vi "Maintenance.vi"() -> ()   [LabVIEW 2020]
doc: "Maintanence VI for FLS imaging system.\n[Covers: REQ9]\n[Covers: REQ10]"
uses:
  <userlib>/_OpenG.lib/file/file.llb/openg_file.lvlib
  <vilib>/event_ctls.llb/usereventprio.ctl
  <instrlib>/niScope/Acquire/Fetch/niScope Multi Fetch Binary 16.vi
  <instrlib>/niScope/Controls/niScope trigger source.ctl
  <userlib>/_OpenG.lib/time/time.llb/openg_time.lvlib
  SubVI/GlobalVariables.vi
  SubVI/LabJack/LJ Pin Setting.ctl
  <vilib>/Utility/error.llb/DialogType.ctl
  <vilib>/Analysis/NI_AALBase.lvlib
  <vilib>/Utility/miscctls.llb/LVMinMaxIncTypeDef.ctl
  <vilib>/Analysis/baseanly.llb/Mean (DBL).vi
  LaguerreDeconLib/DeconEngineClass/LaguerreDeconEngineClass.lvclass
  <vilib>/Utility/miscctls.llb/LVPointTypeDef.ctl
  <vilib>/addons/_JKI.lib/Serialization/JSON/JKI JSON Serialization.lvlib
  SubVI/APD/APDClass.lvclass
  <vilib>/Utility/miscctls.llb/LVRowAndColumnTypeDef.ctl
  SubVI/APD/GainData.ctl
  SubVI/APD/iRFData.ctl
  <vilib>/addons/control/pid/NI_PID_autopid.lvlib
  <vilib>/addons/control/pid/NI_PID_pid.lvlib
  <vilib>/addons/control/pid/pid.llb/PID Advanced (DBL).vi
  <vilib>/addons/control/pid/autopid.llb/PID Online Autotuning (Step Closed Loop).vi
  <vilib>/Instr/_visa.llb/VISA Configure Serial Port (Instr).vi
  SubVI/DigitizerConfiguration/FLImDAQ.ctl
  <vilib>/addons/control/pid/autopid.llb/PID autotuning parameters.ctl
panel:
  in  "Duty Cycle (%)":u32=25
  in  "AB Rep Rate":u16 caption="Rep Rate" max=1000 step=1 format="%.0dHz"
  in  "Current":dbl=1.0 min=1.0 max=63.0 step=1.0 format="%#.1fA"
  out "GainIndicator":dbl caption="Gain"
  out "Noise\n(std of DC)":dbl format="%0.6f"
  in  "BG flag?":bool
  out "DC":dbl format="%0.2f"
  out "Amplitude":dbl
  in  "Gain High":dbl max=4.5
  in  "Gain low":dbl=3.0
  in  "Step":dbl=0.1
  in  "Num WF to acquire":u64=18446744073709551615
  in  "Channel":enum32{"Ch1", "Ch2", "Ch3"}(radio)
  in  "Task":enum32{"iRFAndGain", "Alignment"}(radio)
  in  "Aiming beam toggle":bool caption="445nm 100Hz"
  in  "Laser Rep Rate":u16=120 caption="Rep Rate" min=5 max=4000 step=1 format="%.0dHz"
  in  "355nm Laser toggle":bool caption="355nm 460Hz"
  out "appended path":path
  out "Current State":string
  out "WF max value":dbl
  out "Disclamer":picture
  out "Calibration #":i8
  out "BG #":i8
  in  "TCP Connect":bool
  out "Help":string
  in  "Auto gain":bool=TRUE
  out "Run #":i8
  in  "StopButton":bool caption="Stop"
  out "System Status:":bool
  in  "StartButton":bool caption="Start"
  in  "Ctrl V":dbl=0.05 min=0.0 max=5.5 step=0.1 format="%#.3f"
  out "System Hardware Connection Status":T1
  out "Waveform (no average)":dbl[](graph)
  in  "Tab Control":T2(tab)
  out "Ch1 Max CtrlV":dbl
  out "Ch1 iRF Graph":dbl[][](graph)
  out "Ch1 Gain":cluster{"CtrlV":dbl[], "Gain":dbl[]}(graph)
  out "Serial Number Ch1":string caption="Serial Number"
  out "DateTimeCh1":string caption="DateTime"
  out "Ch2 Gain":cluster{"CtrlV":dbl[], "Gain":dbl[]}(graph)
  out "Ch2 iRF Graph":dbl[][](graph)
  out "Ch2 Max CtrlV":dbl
  out "Serial Number Ch2":string caption="Serial Number"
  out "DateTimeCh2":string caption="DateTime"
  out "Ch3 iRF Graph":dbl[][](graph)
  out "Ch3 Gain":cluster{"CtrlV":dbl[], "Gain":dbl[]}(graph)
  out "Serial Number Ch3":string caption="Serial Number"
  out "Ch3 Max CtrlV":dbl
  out "DateTimeCh3":string caption="DateTime"
  out "display loop timing(ms)":u32
  out "Aquisition loop timing(ms)":u32
  out "DisplayLoop":i32
  out "processing loop":i32
  out "processing loop timing(ms)":dbl
  out "laser EM lamp V":dbl format="%0.6f"
  out "aquisition loop Error Out":errorcluster
  out "Aq Loop?":bool
  out "processing Error Out":errorcluster
  out "Triggering:Trigger Delay":dbl
  out "Foot Pedal":bool
  out "LJ Pinout":T3={"Ch1 Bias"="DAC0", "Ch2 Bias"="DAC1", "Ch3 Bias"="DAC2", "Ch4 Bias"="DAC0", "355 PWM"="FIO0", "AimingBeam PWM"="FIO2", "Laser Ready"="FIO3", "Interlock"="FIO1", "Laser Start/Stop"="FIO1", "Red LED"="FIO1", "Green LED"="DIO3", "Foot Pedal"="DIO15"}
  out "FLImDAQ":T4={"Digitizer 1"="", "Digitizer 2"="", "Channel"=enum."Channel 0", "trigger source"="VAL_EXTERNAL", "trigger level"=0.5, "trigger delay"=1.35e-07, "min sample rate"=12500000000.0, "min record length"=2500, "vertical range"=1.0, "vertical offset"=-0.25, "Waveform to Avg"=2000} caption="FLIm DAQ Configuration" {"trigger delay" format="%^#.4e"; "trigger level" min=0.0 max=3.5 step=0.5 format="%.2f"; "vertical offset" format="%.4f"; "vertical range" format="%.2f"; "min sample rate" format="%#.2p"}
  out "Dig1 Temp":dbl
  out "Dig2 Temp":dbl
  in  "Sys Reconfig":bool
  out "Fetch Record #":i32
  out "Record Backlog":i32
  out "Fetch:Records Done":i32
  out "dt (s)":dbl format="%#_6p"
  in  "SaveData?":bool
  out "data Size":i32[](array[numeric])
  out "numWFInQ":i32
  in  "Clear WF Chart History":bool
  out "Waveform Chart":dbl(graph)
  in  "SaveiRFData":bool
  out "iRFDataTable":string[][](table)
  in  "SetIRFCtrlV":bool
  in  "ClearIRFData":bool
  in  "AcquireIRF":bool
  out "iRFInstSting":string="To aquire gain data, please start data aquisition! \nPlace blue (Ch1&2) or Green(Ch3) Chroma slide as close as possible to the fiber port! \nPlease remove channel 3 bandpass filter as well!"
  out "iRFSigInRange":bool caption="Signal  In Range?"
  out "Current iRF":dbl[](graph)
  out "iRFCtrlV":dbl[](array[numeric])
  in  "SaveGainData":bool
  out "GainInstSting":string="To aquire gain data, please start data aquisition! \nPlace blue (Ch1&2) or Green(Ch3) Chroma slide as close as possible to the fiber port! \nPlease remove channel 3 bandpass filter as well!"
  in  "ClearGainData":bool
  out "Gain":dbl[](array[numeric])
  in  "ComputeGain":bool
  out "Int Corr AUC":dbl[](array[numeric])
  out "AUC Std":dbl[](array[numeric])
  out "GainSigInRange":bool caption="Signal  In Range?"
  in  "AcquireGain":bool
  out "GainDataTable":string[][](table)
  out "Intensity Factor":dbl[](array[numeric])
  out "AUC":dbl[](array[numeric])
  out "Ctrl V":dbl[](array[numeric])
  out "XY Graph":cluster{"Ctrl V":dbl[], dbl[]}(graph)
  out "Parameters":T6(graph)
  in  "Save PID":bool
  out "Targer and Max":cluster{"V target(1.0)":dbl, dbl}(graph)
  out "Completed?":bool
  out "Gain(Log10)":dbl(graph)
  in  "Gain(Log)":dbl=1.0
  in  "Ch1 PID gains":T6={"proportional gain (Kc)"=0.5, "integral time (Ti, min)"=0.0003, "derivative time (Td, min)"=1e-05} {"derivative time (Td, min)" format="%.6f"; "integral time (Ti, min)" format="%.6f"; "proportional gain (Kc)" format="%.6f"}
  in  "autotune? (F)":bool
  in  "PID dt (s)":dbl=-1.0
  out "dt out (s)":dbl format="%.3f"
  in  "V target(1.0)":dbl=1.0 format="%#_2f"
  in  "Accept?":bool
  out "tuned PID gains":T6={"proportional gain (Kc)"=1.0, "integral time (Ti, min)"=0.01, "derivative time (Td, min)"=0.0} {"derivative time (Td, min)" format="%_6f"; "integral time (Ti, min)" format="%.6f"; "proportional gain (Kc)" format="%.6f"}
  in  "autotuning parameters":T7={"type of controller"=2, "relay cycles"=100, "relay amplitude"=0.25, "control specifications"=1, "PV noise level"=0.01} {"PV noise level" format="%.5f"; "control specifications" items=["normal", "fast", "slow"]; "relay amplitude" format="%.2f"; "type of controller" items=["P", "PI", "PID"]}
  in  "Ch2 PID gains":T6={"proportional gain (Kc)"=0.5, "integral time (Ti, min)"=0.0003, "derivative time (Td, min)"=1e-05} {"derivative time (Td, min)" format="%.6f"; "integral time (Ti, min)" format="%.6f"; "proportional gain (Kc)" format="%.6f"}
  in  "Ch3 PID gains":T6={"proportional gain (Kc)"=0.5, "integral time (Ti, min)"=0.0003, "derivative time (Td, min)"=1e-05} {"derivative time (Td, min)" format="%.6f"; "integral time (Ti, min)" format="%.6f"; "proportional gain (Kc)" format="%.6f"}
  in  "gamma":dbl=1.0 format="%.2f"
  in  "alpha":dbl=nan format="%.2f"
  in  "Quit":bool
  # "440nm Laser Setting"
  # "355nm Laser Setting"
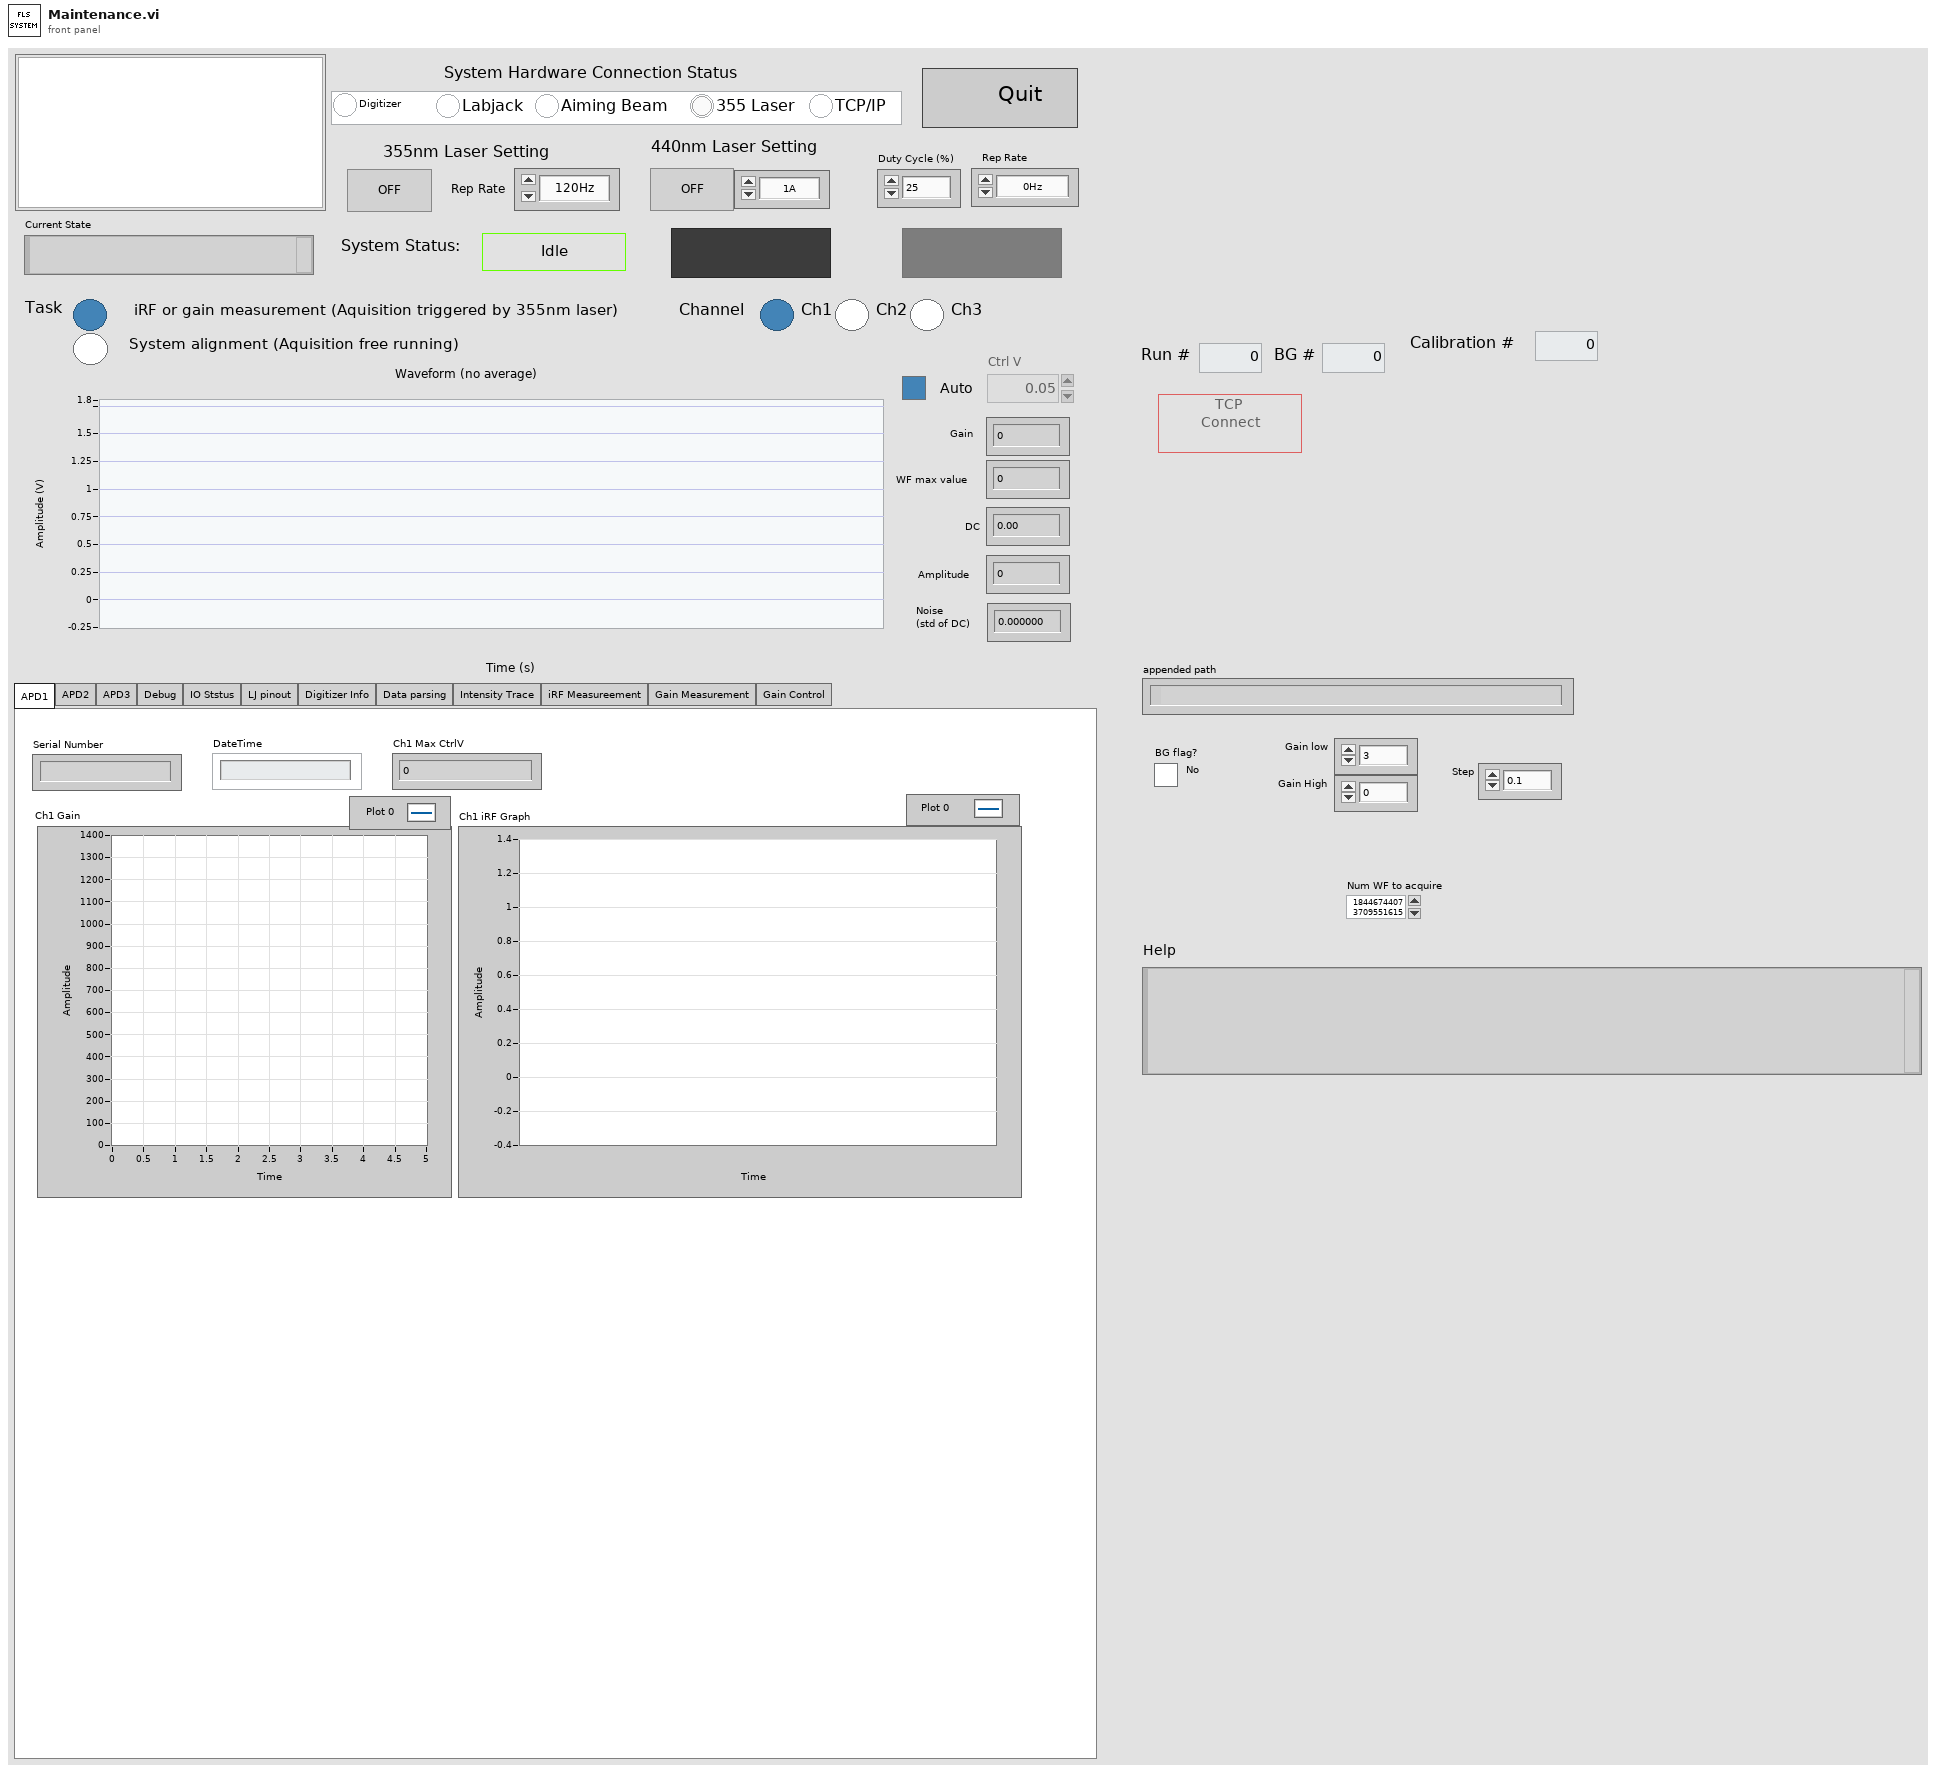
[diagram p1: front panel]
types:
  T1 = cluster{"Digitizer":bool, "Labjack":bool, "Aiming Beam":bool, "355 Laser":bool, "TCP/IP":bool}
  T2 = enum32{"APD1", "APD2", "APD3", "Debug", "IO Ststus", "LJ pinout", "Digitizer Info", "Data parsing", "Intensity Trace", "iRF Measureement", "Gain Measurement", "Gain Control"}
  T3 = typedef "LJ Pin Setting.ctl" = cluster{"Ch1 Bias":string, "Ch2 Bias":string, "Ch3 Bias":string, "Ch4 Bias":string, "355 PWM":string, "AimingBeam PWM":string, "Laser Ready":string, "Interlock":string, "Laser Start/Stop":string, "Red LED":string, "Green LED":string, "Foot Pedal":string}
  T4 = typedef "FLImDAQ.ctl" = cluster{"Digitizer 1":refnum<k15>, "Digitizer 2":refnum<k15>, "Channel":enum16{"Channel 0", "Channel 1", "Channel 0&1"}, "trigger source":T5, "trigger level":dbl, "trigger delay":dbl, "min sample rate":dbl, "min record length":i32, "vertical range":dbl, "vertical offset":dbl, "Waveform to Avg":i16}
  T5 = typedef "niScope trigger source.ctl" = string
  T6 = cluster{"proportional gain (Kc)":dbl, "integral time (Ti, min)":dbl, "derivative time (Td, min)":dbl}
  T7 = typedef "PID autotuning parameters.ctl" = cluster{"type of controller":u16, "relay cycles":i32, "relay amplitude":dbl, "control specifications":u16, "PV noise level":dbl}
  T8 = cluster{"CtrlV":dbl, "WFs":dbl[][], "WFavg":dbl[]}
  T9 = enum16{"open", "replace", "create", "open or create", "replace or create", "replace or create with confirmation"}
  T10 = typedef "LVPointTypeDef.ctl" = cluster{"Horizontal":i16, "Vertical":i16}
  T11 = enum8{"Enabled", "Disabled", "Disabled and Grayed Out"}
  T12 = enum32{"APD1", "APD2", "APD3", "Debug", "IO Ststus", "LJ pinout", "Digitizer Info", "Data parsing"}
  T13 = cluster{"CtrlV":dbl, "PeakV":dbl, "PeakV Std":dbl, "IntFactor":dbl, "IntCorrPeakV":dbl}
  T14 = enum16{"open", "open or create", "create or replace", "create", "open (read-only)"}
  T15 = enum32{"Invalid", "Standard", "Closed", "Hidden", "Minimized", "Maximized"}
  T16 = enum32{"invalid app kind", "Development System", "Run Time System", "Student Edition", "Embedded LabVIEW", "Evaluation", "Custom"}
  T17 = typedef "usereventprio.ctl" = enum32{"high priority", "normal priority"}
  T18 = enum32{"Bad", "Idle", "Run top level", "Running"}
  T19 = typedef "LVRowAndColumnTypeDef.ctl" = cluster{"Row":i32, "Column":i32}
  T20 = typedef "LVMinMaxIncTypeDef.ctl" = cluster{"Minimum":dbl, "Maximum":dbl, "Increment":dbl}
  T21 = cluster{"Aiming Beam COM Port":refnum<visa-resource-name>, "Min Current":dbl, "Max Current":dbl, "Default Current":dbl, "Frequency(Hz)":i32}
  T22 = cluster{"Core":cluster{"Current VI Reference":refnum<vi>, "Close Panel on Exit?":bool}, "SysConfigCluster":cluster{"Ch1Enable?":bool, "Ch2Enable?":bool, "Ch3Enable?":bool, "Ch1AutoGain?":bool, "Ch2AutoGain?":bool, "Ch3AutoGain?":bool, "AimingBeamEnable?":bool}, "System Status":cluster{"Digitizer":bool, "Labjack":bool, "Aiming Beam":bool, "355 Laser":bool, "TCP/IP":bool}, "IDs":cluster{"RunID":i8, "BG ID":i8, "Cali ID":i8}, "DefaultPath":path, "Pathes":cluster{"DataPath":path, "BG Path":path, "iRFPath":path, "CaliPath":path}, "FLImDAQ":cluster{"resource name":refnum<k15>, "resource name 2":refnum<k15>, "Channel":enum16{"Channel 0", "Channel 1", "Channel 0&1"}, "trigger source":T5, "trigger level":dbl, "trigger delay":dbl, "min sample rate":dbl, "min record length":i32, "vertical range":dbl, "vertical offset":dbl, "Waveform to Avg":i32}, "SysRunning?":bool, "AB Cluster":cluster{"Aiming Beam COM Port":refnum<visa-resource-name>, "Min Current":dbl, "Max Current":dbl, "Default Current":dbl, "Frequency(Hz)":i32}, "LJ Pinout":T3, "355 PWM setting":cluster{"DIO_EF_CLOCK1_DIVISOR":i16, "DIO_EF_CLOCK1_ROLL_VALUE":i32, "DIO#_EF_INDEX":i16, "DIO#_EF_OPTIONS":i16, "DIO#_EF_CONFIG_A":i32}, "AB PWM setting":cluster{"DIO_EF_CLOCK1_DIVISOR":i16, "DIO_EF_CLOCK1_ROLL_VALUE":i32, "DIO#_EF_INDEX":i16, "DIO#_EF_OPTIONS":i16, "DIO#_EF_CONFIG_A":i32}, "Last Trigger":u32, "niTClk sessions":refnum<k20>[], "Laser start tic":u32, "TCP attempt count":i32, "iRFAllGain":dbl[][], "SlowTimer":u32, "FastTimer":u32, "TempPath":path, "LED vi reference":refnum<vi>, "APDSerials":cluster{"Ch1Serial":string, "Ch2Serial":string, "Ch3Serial":string}, "LedViRefOpen":bool, "GainBGRaw":dbl[][], "GainDataTemp":cluster{"CtrlV":dbl, "AUC":dbl, "AUC Std":dbl, "IntFactor":dbl, "IntCorrAUC":dbl}, "iRFIdx":i32}
  T23 = cluster{"CtrlV":dbl, "AUC":dbl, "AUC Std":dbl, "IntFactor":dbl, "IntCorrAUC":dbl}
  T24 = cluster{"Ch1Serial":string, "Ch2Serial":string, "Ch3Serial":string}
  T25 = cluster{"DataPath":path, "BG Path":path, "iRFPath":path, "CaliPath":path}
  T26 = cluster{"DIO_EF_CLOCK1_DIVISOR":i16, "DIO_EF_CLOCK1_ROLL_VALUE":i32, "DIO#_EF_INDEX":i16, "DIO#_EF_OPTIONS":i16, "DIO#_EF_CONFIG_A":i32}
  T27 = cluster{"resource name":refnum<k15>, "resource name 2":refnum<k15>, "Channel":enum16{"Channel 0", "Channel 1", "Channel 0&1"}, "trigger source":T5, "trigger level":dbl, "trigger delay":dbl, "min sample rate":dbl, "min record length":i32, "vertical range":dbl, "vertical offset":dbl, "Waveform to Avg":i32}
  T28 = cluster{"Ch1Enable?":bool, "Ch2Enable?":bool, "Ch3Enable?":bool, "Ch1AutoGain?":bool, "Ch2AutoGain?":bool, "Ch3AutoGain?":bool, "AimingBeamEnable?":bool}
  T29 = cluster{"Current VI Reference":refnum<vi>, "Close Panel on Exit?":bool}
  T30 = typedef "DialogType.ctl" = u16
  T31 = typedef "LJ PWM Setting.ctl" = cluster{"DIO_EF_CLOCK1_DIVISOR":i16, "DIO_EF_CLOCK1_ROLL_VALUE":i32, "DIO#_EF_INDEX":i16, "DIO#_EF_OPTIONS":i16, "DIO#_EF_CONFIG_A":i32}
  T32 = typedef "AimingBeam.ctl" = cluster{"Aiming Beam COM Port":refnum<visa-resource-name>, "Min Current":dbl, "Max Current":dbl, "Default Current":dbl, "Frequency(Hz)":u32}
  T33 = typedef "LVBoundsTypeDef.ctl" = cluster{"Width":u32, "Height":u32}
  T34 = typedef "imagedata.ctl" = cluster{"image type":i32, "image depth":i32, "image":u8[], "mask":u8[], "colors":u32[], "Rectangle":cluster{"left":i16, "top":i16, "right":i16, "bottom":i16}}
  T35 = typedef "LVCursorListTypeDef.ctl" = cluster{"Name":string, "Color":u32, "Style":u8, "Point Style":u8, "Name Visible":bool, "Allow Drag":bool, "Cursor Mode":u32, "Plot":i32, "Index":i32, "Position":cluster{"X":dbl, "Y":dbl}, "X Scale":u32, "Y Scale":u32, "Watch Plots":i32[], "Watch All Plots":bool, "Plot Area":i32, "Label Offset":cluster{"X":dbl, "Y":dbl}}[]
  T36 = cluster{"Name":string, "Color":u32, "Style":u8, "Point Style":u8, "Name Visible":bool, "Allow Drag":bool, "Cursor Mode":u32, "Plot":i32, "Index":i32, "Position":cluster{"X":dbl, "Y":dbl}, "X Scale":u32, "Y Scale":u32, "Watch Plots":i32[], "Watch All Plots":bool, "Plot Area":i32, "Label Offset":cluster{"X":dbl, "Y":dbl}}
  T37 = cluster{"Name":string, "Color":u32, "Style":u8, "Point Style":u8, "Name Visible":bool, "Allow Drag":bool, "Cursor Mode":u32, "Plot":i32, "Index":i32, "Position":cluster{"X":dbl, "Y":dbl}, "X Scale":u32, "Y Scale":u32, "Watch Plots":i32[], "Watch All Plots":bool, "Plot Area":i32, "Label Offset":cluster{"X":dbl, "Y":dbl}}[]
  T38 = cluster{"Ch1APDSerial#":string, "Ch2APDSerial#":string, "Ch3APDSerial#":string, "Ch4APDSerial#":string}
  T39 = cluster{"Ch1APDSerial#":string, "Ch2APDSerial#":string, "Ch3APDSerial#":string}
  T40 = typedef "GainData.ctl" = cluster{"CtrlV":dbl[], "NumOfWFs":i32, "WF length":i32, "Gain":dbl[], "GainRaw":dbl[][], "GainBGRaw":dbl[][]}
  T41 = typedef "iRFData.ctl" = cluster{"dt":dbl, "NumOfWFs":i32, "WFLength":i32, "iRFCtrlV":dbl[], "iRFWFsAvg":dbl[][], "iRFRaw":dbl[][]}
  T42 = cluster{"CtrlV":dbl, "WFs":dbl[][], "WFavg":dbl[]}[]
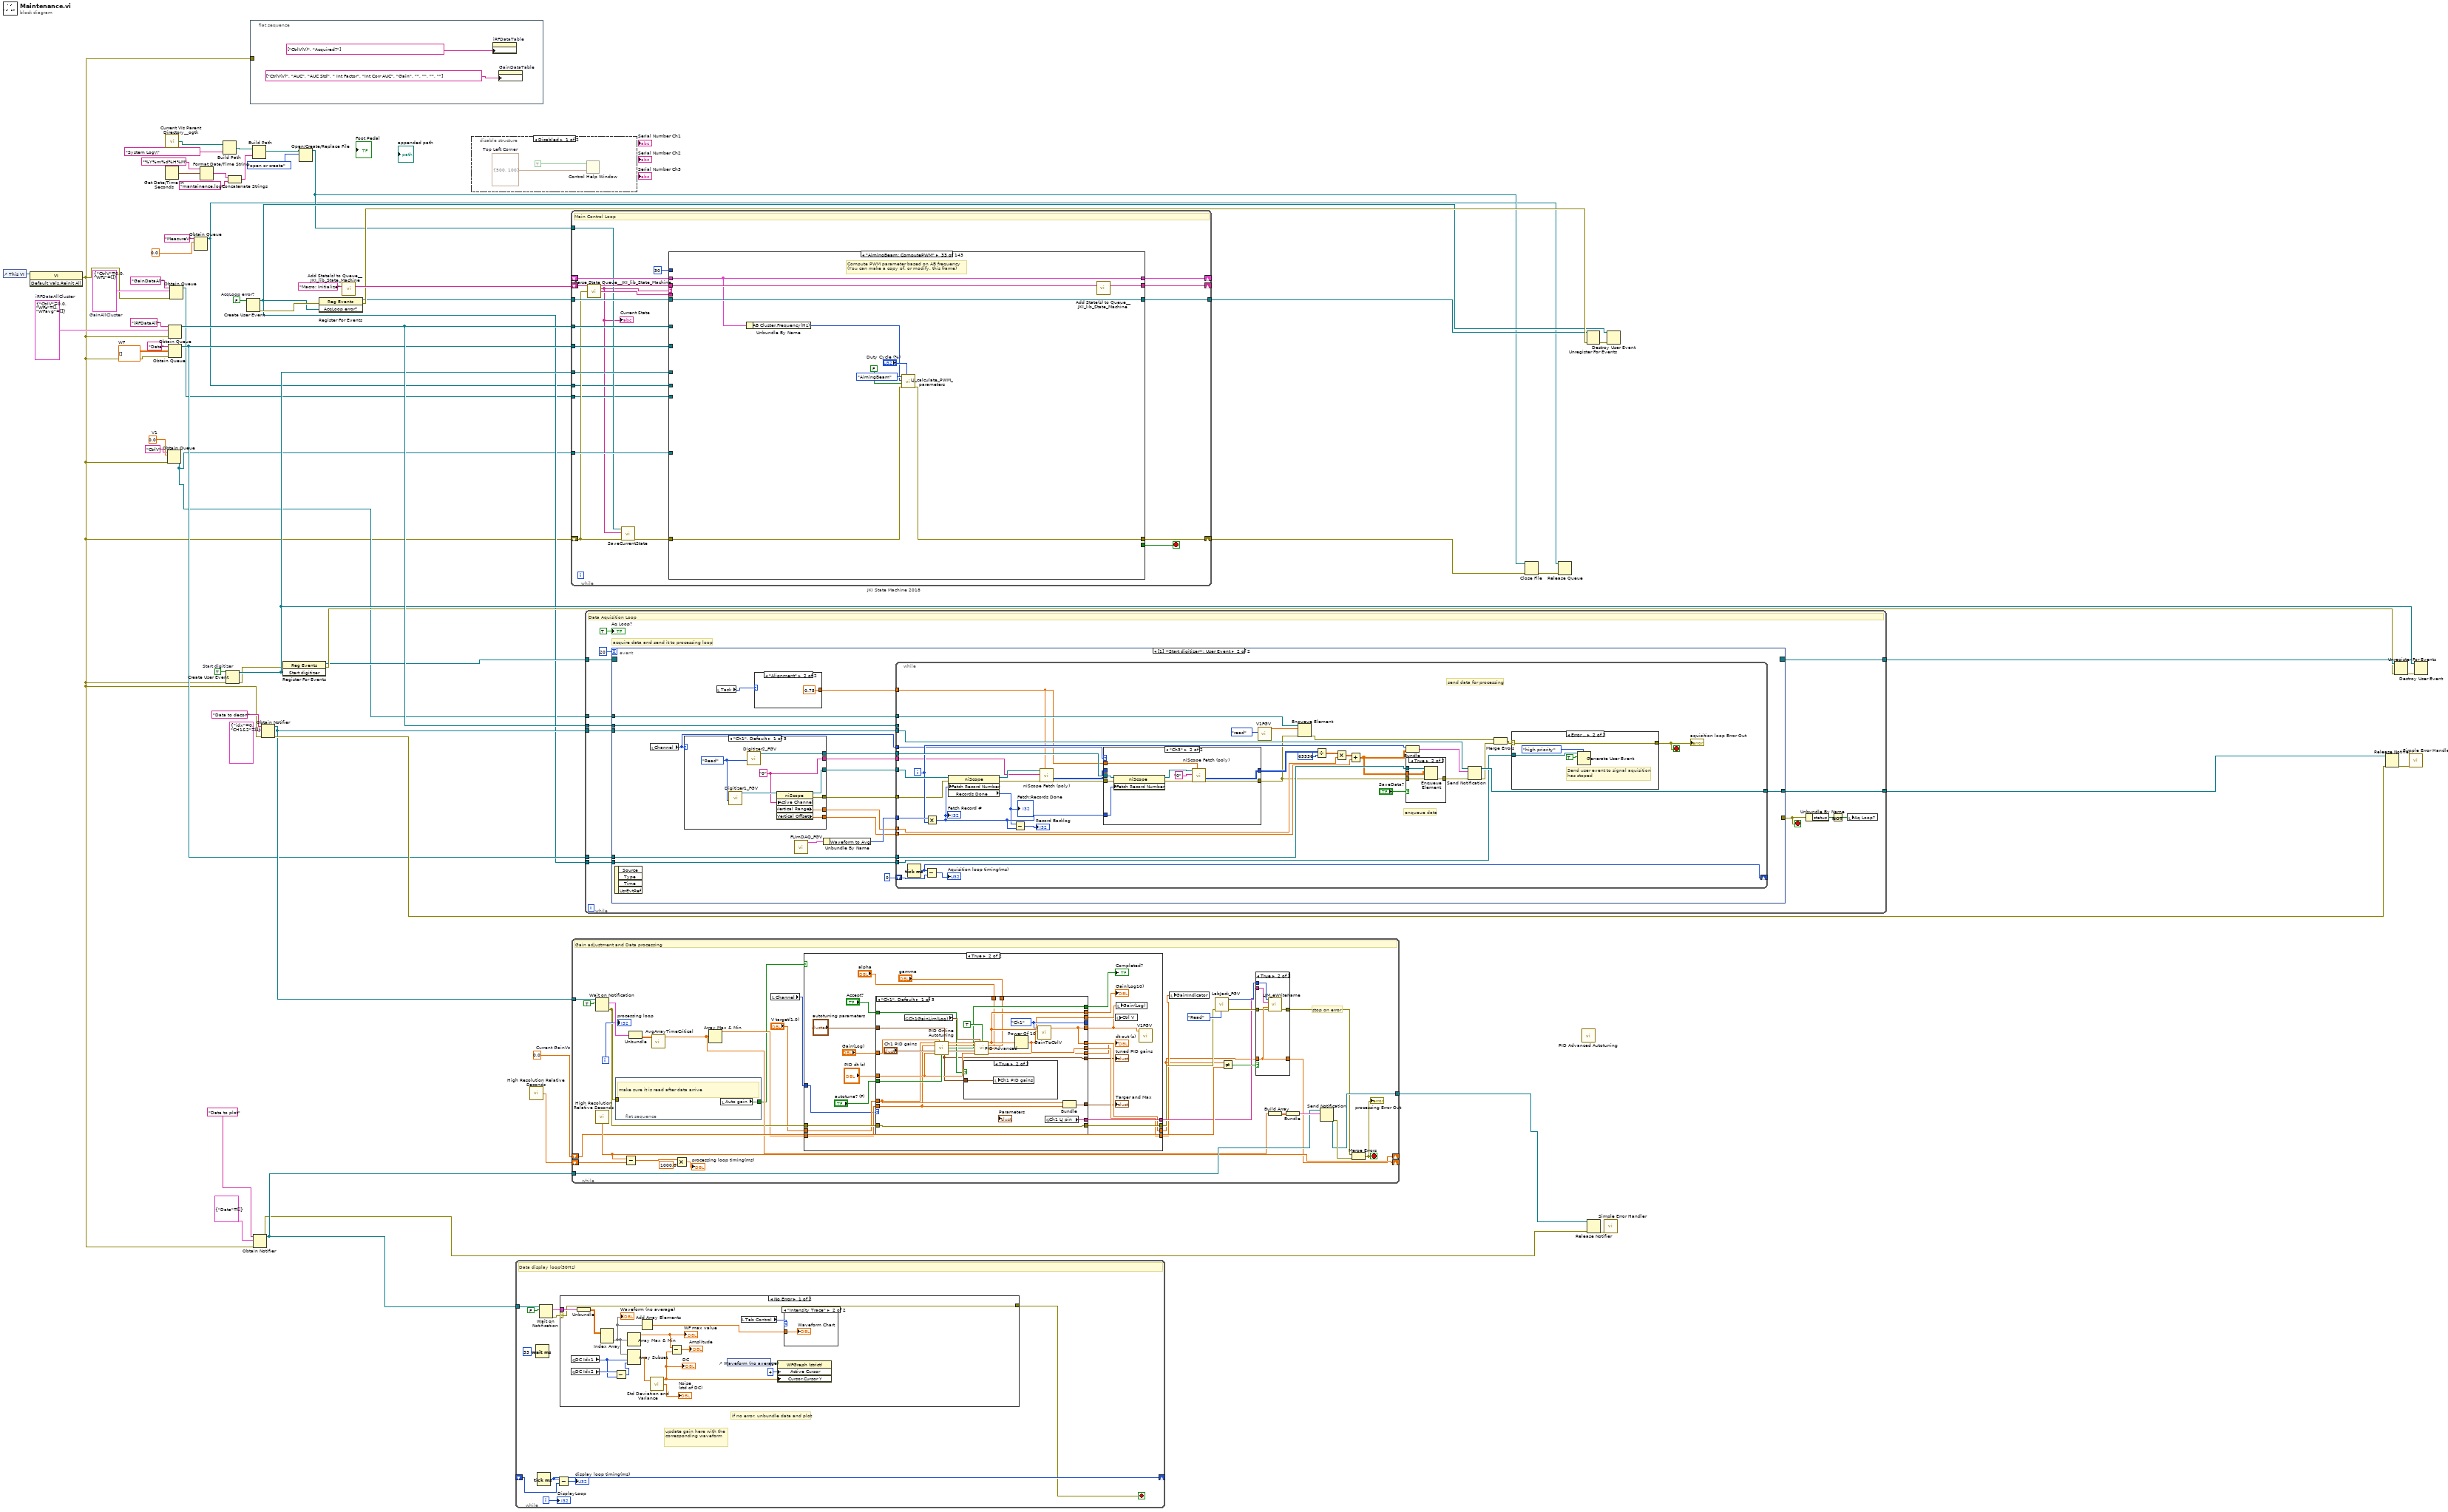
[diagram p0: block diagram]
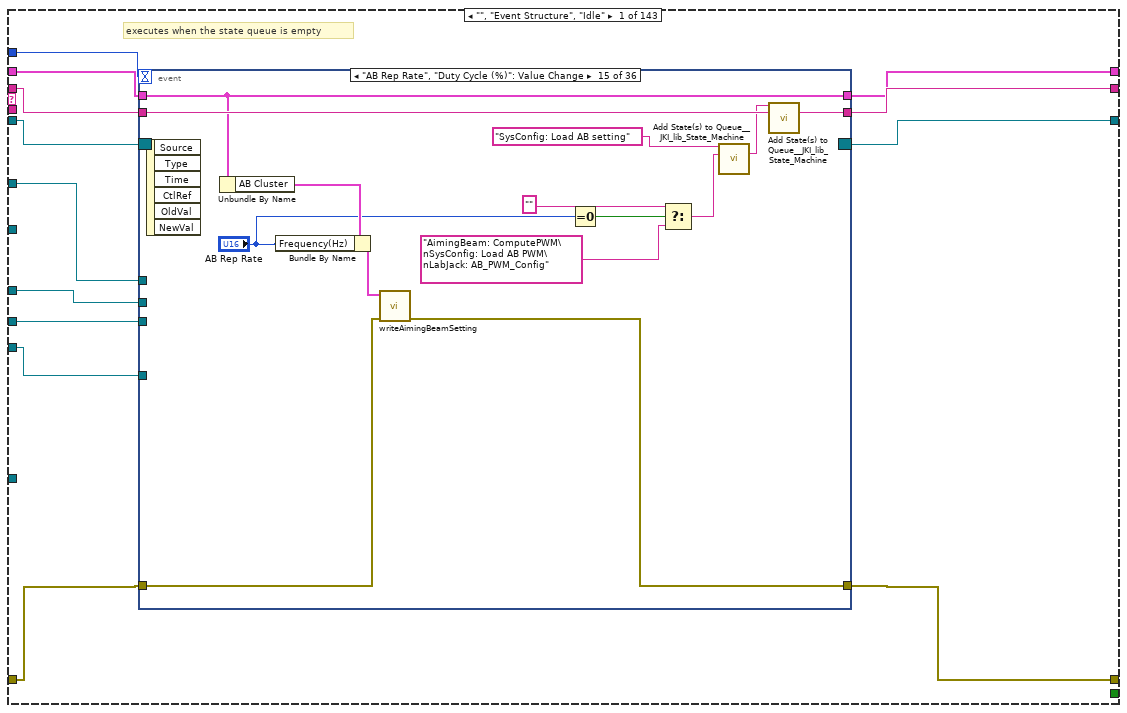
[diagram p3: hidden frame]
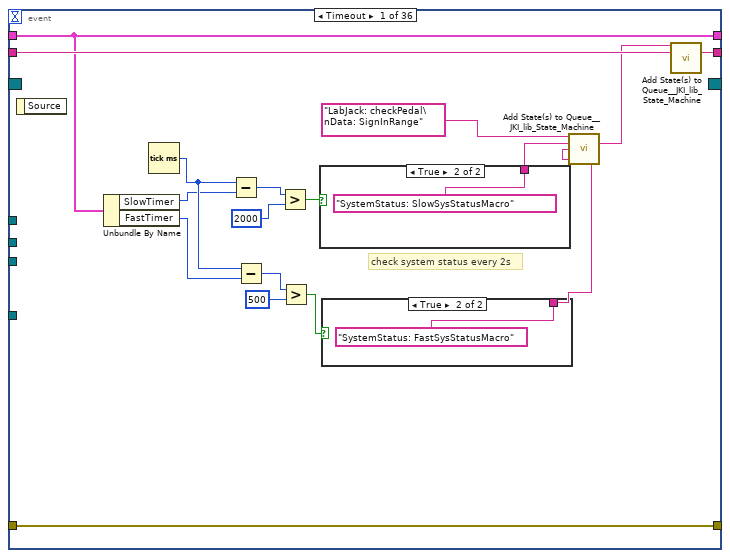
[diagram p4: hidden frame]
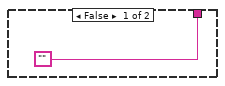
[diagram p5: hidden frame]
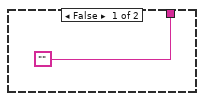
[diagram p6: hidden frame]
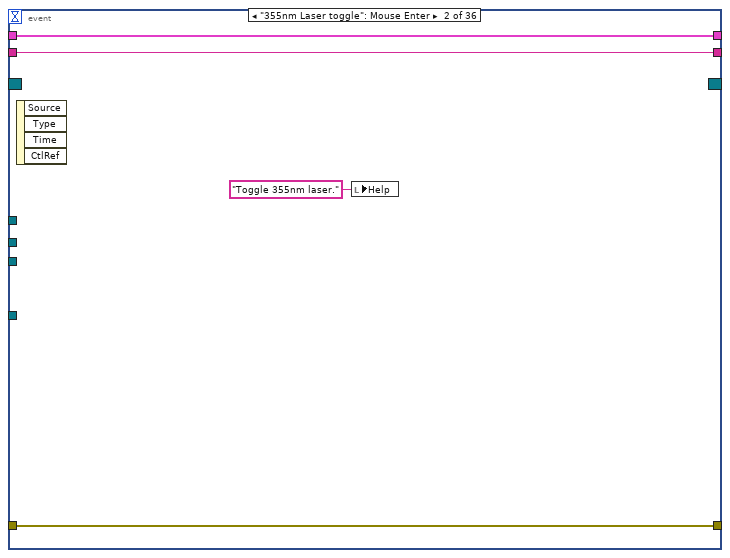
[diagram p7: hidden frame]
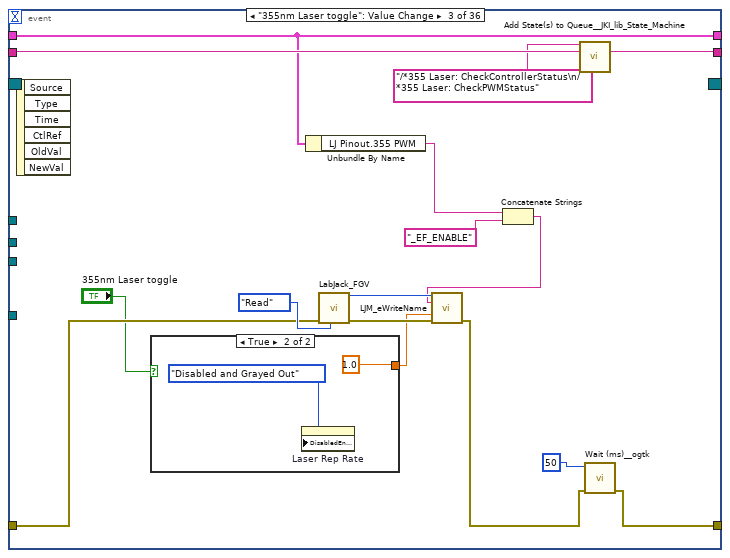
[diagram p8: hidden frame]
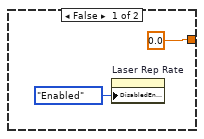
[diagram p9: hidden frame]
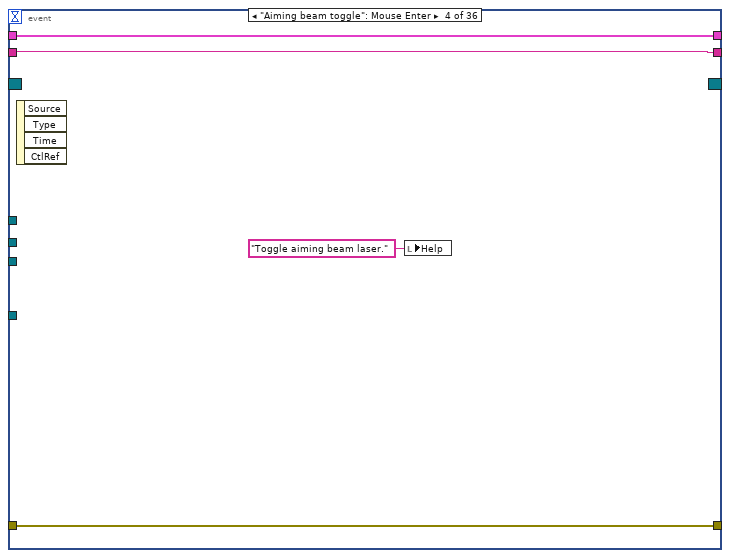
[diagram p10: hidden frame]
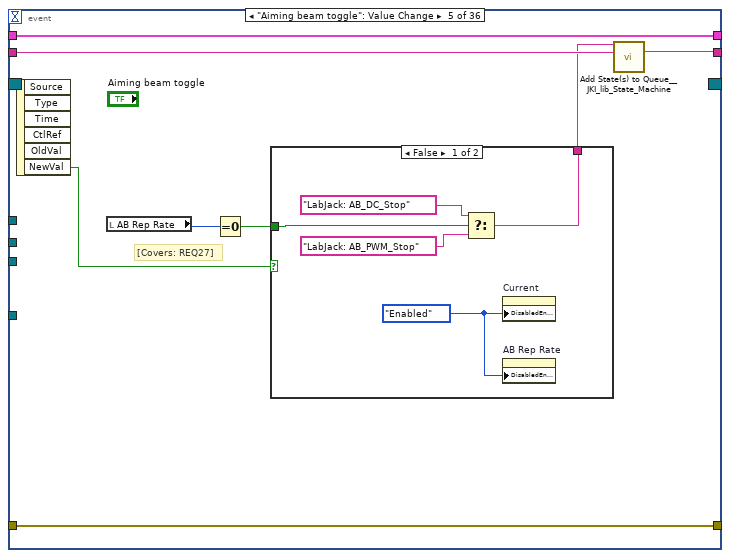
[diagram p11: hidden frame]
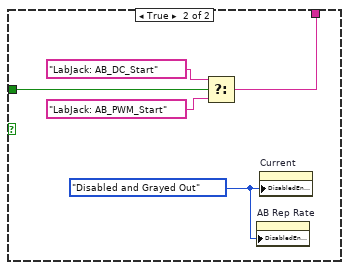
[diagram p12: hidden frame]
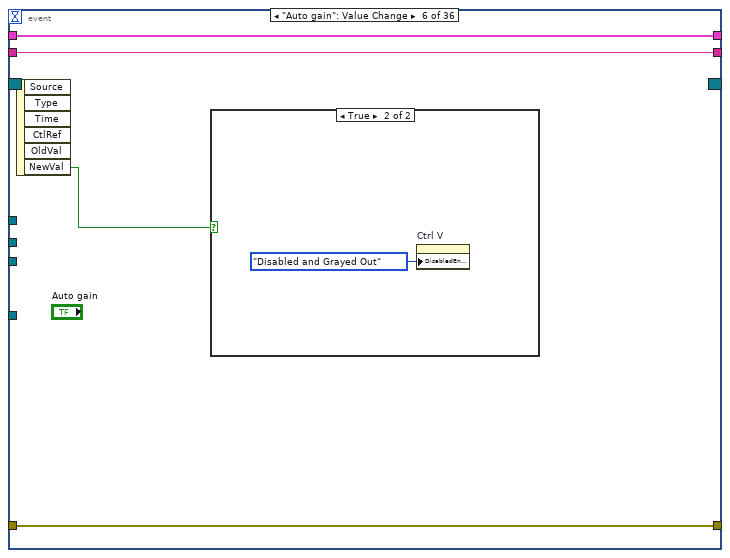
[diagram p13: hidden frame]
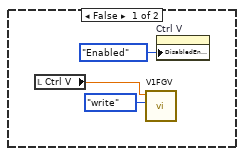
[diagram p14: hidden frame]
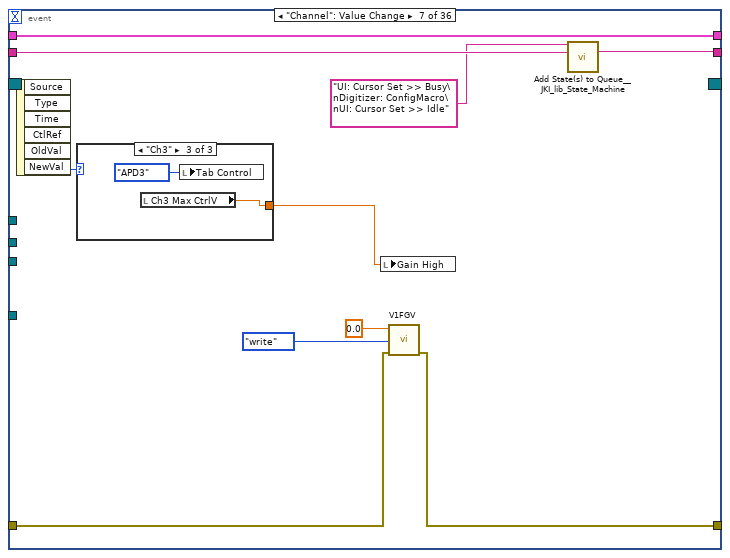
[diagram p15: hidden frame]
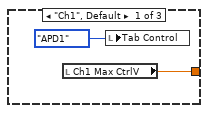
[diagram p16: hidden frame]
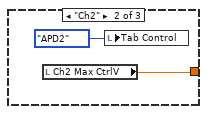
[diagram p17: hidden frame]
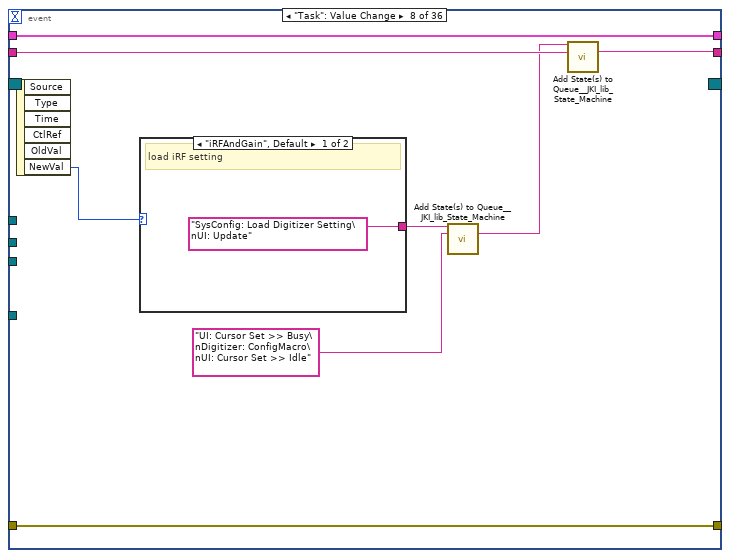
[diagram p18: hidden frame]
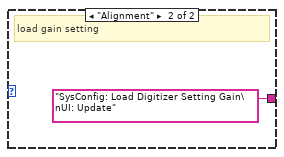
[diagram p19: hidden frame]
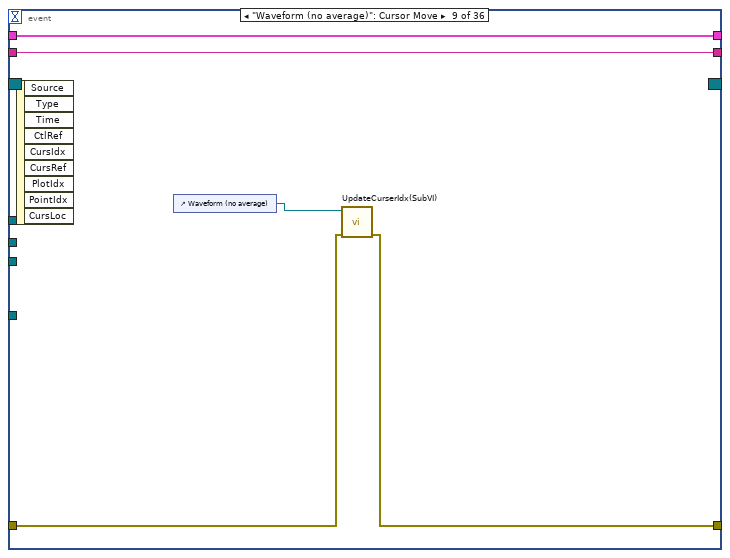
[diagram p20: hidden frame]
diagram:
  w3 = cluster{"CtrlV":dbl, "WFs":dbl[][]} {"CtrlV"=0.0, "WFs"=[]}  # GainAllCluster
  w5 = T8 {"CtrlV"=0.0, "WFs"=[], "WFavg"=[]}  # iRFDataAllCluster
  w22 = 0.0  # V1
  w26 = 0.0  # Current GainVs
  w43 = FALSE  # AcqLoop error?
  w53 = TRUE  # Start digitizer
  w56 = dbl[][] []  # WF
  n1 = control-ref of="This VI"() -> (w58:refnum<vi>)
  n2 = invoke on="Invoke Node" class="VI" method="Default Vals.Reinit All"(reference=w58) -> (error out=w1:errorcluster)  [unwired: 2 in, 2 out]
  n3 = call <userlib>:"Current VIs Parent Directory__ogtk.vi"() -> ("Parent Directory (+ Relative)"=w21:path)  [unwired: 5 in]
  n4 = Get Date/Time In Seconds() -> (seconds since 1Jan1904=w19:timestamp)
  n5 = Obtain Queue(name (unnamed)="CtrlV", element data type=w22, error in (no error)=w1) -> (queue out=w24:refnum<queue>)  [unwired: 2 in, 2 out]
  n6 = Obtain Queue(name (unnamed)="Data", element data type=w56, error in (no error)=w1) -> (queue out=w32:refnum<queue>)  [unwired: 2 in, 2 out]
  n7 = Obtain Queue(name (unnamed)="iRFDataAll", element data type=w5, error in (no error)=w1) -> (queue out=w54:refnum<queue>)  [unwired: 2 in, 2 out]
  n8 = Obtain Queue(name (unnamed)="GainDataAll", element data type=w3, error in (no error)=w1) -> (queue out=w2:refnum<queue>)  [unwired: 2 in, 2 out]
  n9 = Obtain Queue(name (unnamed)="MeasureV", element data type=0.0) -> (queue out=w6:refnum<queue>)  [unwired: 3 in, 2 out]
  n10 = Format Date/Time String(time format string (%c)="%Y%m%d%H%M", seconds (now)=w19) -> (date/time string=w16:string)  [unwired: 1 in]
  n11 = Build Path(base path=w21, name or relative path="System Log\\") -> (appended path=w12:path)
  n12 = Create User Event(user event datatype=w53, error in=w1) -> (user event=w42:refnum<user-event>, error out=w28:errorcluster)
  n13 = Concatenate Strings(w16, "mantainence.log" ("string")) -> (w14:string)
  n14 = Create User Event(user event datatype=w43) -> (user event=w27:refnum<user-event>, error out=w29:errorcluster)  [unwired: 1 in]
  n15 = flat-sequence {
    tunnel: w1 -> [_]
    frame #0 {
      n16 = property on="iRFDataTable" class="Tbl (strict)"("Column Headers[]"=string[] ["CtrlV(V)", "Acquired?"] ("Column Header Strings[]")) -> ()  [unwired: 2 in, 2 out]
      n17 = property on="GainDataTable" class="Tbl (strict)"("Column Headers[]"=string[] ["CtrlV(V)", "AUC", "AUC Std", " Int Factor", "Int Corr AUC", "Gain", "", "", "", ""] ("Column Header Strings[]")) -> ()  [unwired: 2 in, 2 out]
    }
  }
  n18 = Build Path(base path=w12, name or relative path=w14) -> (appended path=w17:path)
  n19 = Obtain Notifier(name (unnamed)="Data to plot", notification data type=cluster{"Data":dbl[][]} {"Data"=[]}, error in (no error)=w1) -> (notifier out=w36:refnum<notifier>, error out=w33:errorcluster)  [unwired: 1 in, 1 out]
  n20 = Obtain Notifier(name (unnamed)="Data to decon", notification data type=cluster{"idx":i32, "CH1&2":dbl[][]} {"idx"=0, "CH1&2"=[]}, error in (no error)=w1) -> (notifier out=w39:refnum<notifier>, error out=w47:errorcluster)  [unwired: 1 in, 1 out]
  n21 = register-events(error in=w28, w42) -> (reference out=w44:refnum<event-registration>, error out=w50:errorcluster)  [unwired: 1 in]
  n22 = Open/Create/Replace File(file path (use dialog)=w17, operation (0:open)=T9."open or create") -> (refnum out=w10:refnum<file>)  [unwired: 4 in, 2 out]
  n23 = register-events(error in=w29, w27) -> (reference out=w31:refnum<event-registration>, error out=w40:errorcluster)  [unwired: 1 in]
  n24 = call <vilib>:"Add State(s) to Queue__JKI_lib_State_Machine.vi"("State(s) in (\"\")"="Macro: Initialize") -> ("States Out"=w60:string)  [unwired: 14 in]
  n25 = disable-structure "Diagram Disable Structure" shown="Disabled" {
    frame Disabled {
      w63 = T10 {"Horizontal"=500, "Vertical"=100}  # Top Left Corner
      n26 = Control Help Window(0:w63, 1:TRUE ("Show")) -> ()
    }
    frame Enabled {
    }
  }
  n27 = while {
    tunnel: w36 -> [w74]
    shift-right: [w68] -> _
    shift-left: _ -> [w72]
    i -> [w66]
    stop <- w65 stop-if-true
    # "if no error, unbundle data and plot"
    # "update gain here with the corresponding waveform"
    # "Data display loop(30Hz)"
    n28 = Wait (ms)(milliseconds to wait=u32 33) -> ()  [unwired: 1 out]
    n29 = Tick Count (ms)() -> (millisecond timer value=w68:u32)
    n30 = Wait on Notification(notifier=w74, ignore previous (F)=FALSE) -> (notification=w69:cluster{"Data":dbl[][]}, error out=w67:errorcluster)  [unwired: 2 in, 2 out]
    n31 = Subtract(x=w68, y=w72) -> (x-y=→"display loop timing(ms)":u32)
    n32 = case shown="No Error" w67 {
      selector: w67 -> [w83 w92]
      tunnel: w69 -> [w90 _]
      tunnel: [w83 w92] -> w65
      frame No Error {
        n33 = global read "GlobalVariables.vi" "DC Idx1"() -> (w76:i32)
        n34 = global read "GlobalVariables.vi" "DC Idx2"() -> (w77:i32)
        n35 = Unbundle(w90) -> ("Data"=w87:dbl[][])
        n36 = Index Array(array=w87) -> (element=w86:dbl[])  [unwired: 2 in]
        "Waveform (no average)" <- w86
        n37 = Subtract(x=w77, y=w76) -> (x-y=w75:i32)
        n38 = Array Max & Min(array=w86) -> (max value=w89:dbl)  [unwired: 3 out]
        "WF max value" <- w89
        n39 = Array Subset(array=w86, index=w76, length=w75) -> (w82:dbl[])
        n40 = Add Array Elements(numeric array=w86) -> (sum=w85:dbl)
        n41 = call <vilib>:"Std Deviation and Variance.vi"("X"=w82) -> ("mean"=w78:dbl, "standard deviation"=→"Noise\n(std of DC)":dbl)  [unwired: 1 in, 1 out]
        "DC" <- w78
        n42 = Subtract(x=w89, y=w78) -> (x-y=→"Amplitude":dbl)
        n43 = control-ref of="Waveform (no average)"() -> (w80:refnum<vi>)
        n44 = local read "Tab Control"() -> (w84:T2)
        n45 = property class="WFGraph (strict)"(reference=w80, "Active Cursor"=u32 4, "Cursor.Cursor Y"=w78) -> ()  [unwired: 1 in, 2 out]
        n46 = case shown="\"Intensity Trace\"" w84 {
          tunnel: w85 -> [_ w91]
          frame "APD1", Default {
          }
          frame "Intensity Trace" {
            "Waveform Chart" <- w91
          }
        }
      }
      frame Error {
      }
    }
    "DisplayLoop" <- w66
  }
  n47 = call <vilib>:"High Resolution Relative Seconds.vi"() -> ("relative seconds"=w23:dbl)
  n48 = while "JKI State Machine 2018" {
    shift-right: [w109] -> _
    shift-left: _ -> [w108]
    shift-right: [w99] -> w11
    shift-left: w1 -> [w98]
    shift-right: [w110] -> _
    shift-left: w60 -> [w111]
    tunnel: w54 -> [w106]
    tunnel: w32 -> [w105]
    tunnel: w42 -> [w104]
    tunnel: w31 -> [w103]
    tunnel: [w102] -> w30
    tunnel: w24 -> [w100]
    tunnel: w10 -> [w96]
    tunnel: w6 -> [w95]
    tunnel: w2 -> [w94]
    stop <- w101 stop-if-true
    # "Main Control Loop"
    n49 = call <vilib>:"Parse State Queue__JKI_lib_State_Machine.vi"("State Queue"=w111, "Error In (no error)"=w98) -> ("Remaining States"=w113:string, "Current State"=w93:string, "Arguments"=w112:string)  [unwired: 11 in]
    "Current State" <- w93
    n50 = call "SaveCurrentState.vi"("error in (no error)"=w98, "Current State"=w93, "Byte Stream File in"=w96) -> ("error out"=w97:errorcluster)  [unwired: 8 in]
    n51 = case shown="\"AimingBeam: ComputePWM\"" w93 {
      selector: w93 -> [_ _ _ _ _ _ _ _ _ _ _ _ _ _ _ _ _ _ _ _ _ _ w826 _ _ _ _ _ _ _ _ _ _ _ _ _ _ _ _ _ _ _ _ _ _ _ _ _ _ _ _ _ _ _ _ _ _ _ _ _ _ _ _ _ _ _ _ _ _ _ _ _ _ _ _ _ _ _ _ _ _ _ _ _ _ _ _ _ _ _ _ _ _ _ _ _ _ _ _ _ _ _ _ _ _ _ _ _ _ _ _ _ _ _ _ _ _ _ _ _ _ _ _ _ _ _ _ _ _ _ _ _ _ _ _ _ _ _ _ _ _ _ _]
      tunnel: w113 -> [w126 w458 w467 w473 w480 w489 w500 w509 w534 w549 w580 w586 w611 w632 w649 w661 w692 w725 w780 w812 w819 w824 w830 w855 w863 w887 w892 w904 w913 w930 w938 w954 w978 w983 w993 w1016 w1065 w1096 w1119 w1142 w1165 w1190 w1213 w1247 w1262 w1278 w1283 w1294 w1305 w1321 w1359 w1376 w1390 w1424 w1435 w1441 w1452 w1464 w1495 w1527 w1540 w1553 w1567 w1581 w1586 w1598 w1610 w1623 w1636 w1652 w1680 w1695 w1700 w1709 w1747 w1760 w1768 w1776 w1790 w1795 w1801 w1818 w1835 w1851 w1871 w1896 w1904 w1909 w1917 w1925 w1930 w1939 w1978 w2018 w2023 w2046 w2059 w2077 w2083 w2094 w2107 w2125 w2132 w2144 w2209 w2220 w2233 w2258 w2281 w2287 w2293 w2308 w2353 w2361 w2367 w2372 w2378 w2386 w2395 w2405 w2411 w2417 w2422 w2428 w2441 w2475 w2484 w2495 w2517 w2539 w2566 w2631 w2648 w2703 w2752 w2768 w2778 w2801 w2806 w2828 w2836 w2845 w2850]
      tunnel: w112 -> [_ _ _ _ _ _ _ _ _ _ _ _ _ _ _ _ _ _ _ _ _ _ _ _ _ _ _ _ _ _ w937 _ _ _ _ _ _ _ _ _ _ _ _ _ _ _ _ _ _ _ _ _ _ _ _ _ _ w1462 _ _ _ _ _ _ _ _ _ _ _ _ _ _ _ _ _ _ _ _ _ _ _ _ _ _ _ _ _ _ _ _ _ _ _ _ _ w2037 _ _ _ _ _ _ w2127 w2139 _ _ _ _ w2277 _ _ _ _ _ _ _ w2373 _ w2387 w2400 _ _ _ _ _ _ _ _ _ _ _ _ _ _ _ _ _ w2792 _ _ _ _ _]
      tunnel: w108 -> [w124 w455 w463 w470 w476 w483 w497 w507 w518 w546 _ w583 w605 w623 w646 w652 w689 w719 w762 w785 w813 w821 w828 w838 w860 w885 w889 w894 w906 w915 w931 w950 w970 w980 w990 w1013 w1030 w1080 w1104 w1126 w1149 w1172 w1210 w1234 w1260 w1264 w1280 w1287 w1298 w1310 w1347 w1363 w1380 w1400 w1433 w1438 w1442 w1454 w1472 w1505 w1529 w1542 w1556 w1569 w1583 w1595 w1607 w1618 w1630 w1647 w1668 w1683 w1697 w1705 w1745 w1757 w1765 w1774 w1788 w1792 w1799 w1802 w1819 w1836 w1852 w1877 w1900 w1906 w1910 w1918 w1927 w1936 w1973 w1999 w2030 w2043 w2057 w2074 w2080 w2087 w2099 w2121 w2130 w2137 w2206 w2211 w2225 w2250 w2278 w2284 w2290 w2294 w2340 w2358 w2364 w2369 w2375 w2383 w2392 w2402 w2408 w2414 w2419 w2425 w2439 w2473 w2481 w2493 w2501 w2523 w2564 w2628 w2642 w2697 w2750 w2765 w2776 w2793 w2803 w2807 w2833 w2843 w2847]
      tunnel: [w123 w456 w465 w471 w478 w487 w498 w501 w532 w547 w578 w584 w601 w617 w647 w656 w690 w700 w768 w791 w816 w822 w832 w853 errorcluster {"status"=FALSE, "code"=0, "source"=""} ("error out") w884 w890 w899 w911 w922 w935 w949 w972 w981 w991 w1011 w1056 w1088 w1111 w1134 w1157 w1183 w1205 w1236 w1250 w1268 w1281 w1284 w1295 w1315 w1348 w1370 w1383 w1404 w1427 w1439 w1450 w1456 w1477 w1509 w1532 w1545 w1557 w1573 w1584 w1588 w1600 w1619 w1631 w1641 w1670 w1685 w1698 w1702 w1740 w1758 w1766 w1771 w1785 w1793 w1796 w1807 w1824 w1846 w1866 w1891 w1897 w1907 w1915 w1923 w1928 w1937 w1976 w2016 w2031 w2044 w2056 w2075 w2081 w2092 w2105 w2123 w2128 w2141 w2207 w2217 w2229 w2253 w2279 w2285 w2291 w2299 w2345 w2359 w2365 w2370 w2376 w2384 w2393 w2403 w2409 w2415 w2420 w2426 w2434 w2470 w2482 w2487 w2500 w2522 w2549 w2627 w2643 w2699 w2744 w2766 w2772 w2795 w2804 w2808 w2834 w2841 w2848] -> w99
      tunnel: w97 -> [w122 w456 w465 w471 w478 w487 w498 w501 w532 w547 w578 w584 w606 w627 w647 w658 w690 w699 w767 w800 w817 w822 w831 w853 w856 w884 w890 w900 w910 w921 w934 w951 w971 w981 w991 w1010 w1059 w1090 w1113 w1136 w1159 w1184 w1204 w1235 w1251 w1270 w1281 w1290 w1301 w1314 w1349 w1371 w1388 w1408 w1426 w1439 w1448 w1459 w1476 w1497 w1531 w1544 w1561 w1572 w1584 w1587 w1599 w1620 w1633 w1648 w1669 w1686 w1698 w1701 w1738 w1758 w1766 w1769 w1779 w1793 w1796 w1813 w1830 w1845 w1865 w1890 w1898 w1907 w1915 w1923 w1928 w1937 w1976 w2016 w2031 w2044 w2056 w2075 w2081 w2092 w2105 w2123 w2129 w2142 w2207 w2217 w2227 w2256 w2279 w2285 w2291 w2303 w2344 w2359 w2365 w2370 w2376 w2384 w2393 w2403 w2409 w2415 w2420 w2426 w2432 w2469 w2482 w2488 w2497 w2519 w2548 _ w2645 w2698 w2746 w2766 w2771 w2796 w2804 w2809 w2834 w2840 w2848]
      tunnel: [w125 w457 w466 w472 w479 w488 w499 w508 w533 w548 w579 w585 w610 w631 w648 w660 w691 w724 w779 w811 w818 w823 w829 w854 w862 w886 w891 w903 w912 w929 w938 w953 w977 w982 w992 w1015 w1064 w1095 w1118 w1141 w1164 w1189 w1212 w1246 w1261 w1277 w1282 w1293 w1304 w1320 w1358 w1375 w1389 w1423 w1434 w1440 w1451 w1463 w1494 w1526 w1539 w1552 w1566 w1580 w1585 w1597 w1609 w1622 w1635 w1651 w1679 w1694 w1699 w1708 w1746 w1759 w1767 w1775 w1789 w1794 w1800 w1817 w1834 w1850 w1870 w1895 w1903 w1908 w1916 w1924 w1929 w1938 w1977 w2017 w2032 w2045 w2058 w2076 w2082 w2093 w2106 w2124 w2131 w2143 w2208 w2219 w2232 w2257 w2280 w2286 w2292 w2307 w2352 w2360 w2366 w2371 w2377 w2385 w2394 w2404 w2410 w2416 w2421 w2427 w2440 w2474 w2483 w2494 w2516 w2538 w2565 w2630 w2647 w2702 w2751 w2767 w2777 w2800 w2805 w2827 w2835 w2844 w2849] -> w110
      tunnel: [_ _ _ _ _ _ _ _ _ _ _ _ _ _ _ _ _ _ _ _ _ _ _ _ _ TRUE _ _ _ _ _ _ _ _ _ _ _ _ _ _ _ _ _ _ _ _ _ _ _ _ _ _ _ _ _ _ _ _ _ _ _ _ _ _ _ _ _ _ _ _ _ _ _ _ _ _ _ _ _ _ _ _ _ _ _ _ _ _ _ _ _ _ _ _ _ _ _ _ _ _ _ _ _ _ _ _ _ _ _ _ _ _ _ _ _ _ _ _ _ _ _ _ _ _ _ _ _ _ _ _ _ _ _ _ _ _ _ _ _ _ _ _ _] -> w101
      tunnel: [w121 w455 w463 w470 w476 w483 w497 w507 w518 w546 w556 w583 w605 w623 w646 w653 w689 w718 w763 w785 w813 w821 w828 w837 w860 w885 w889 w895 w905 w915 w931 w950 w970 w980 w990 w1013 w1029 w1079 w1103 w1125 w1148 w1177 w1210 w1234 w1260 w1263 w1280 w1287 w1298 w1311 w1347 w1363 w1381 w1400 w1433 w1438 w1443 w1454 w1472 w1505 w1529 w1542 w1556 w1569 w1583 w1595 w1607 w1616 w1630 w1647 w1668 w1683 w1697 w1705 w1745 w1757 w1765 w1774 w1788 w1792 w1799 w1803 w1820 w1837 w1853 w1878 w1901 w1906 w1911 w1919 w1927 w1936 w1973 w1999 w2030 w2043 w2057 w2074 w2080 w2088 w2100 w2121 w2130 w2137 w2206 w2211 w2226 w2251 w2278 w2284 w2290 w2295 w2340 w2358 w2364 w2369 w2375 w2383 w2392 w2402 w2408 w2414 w2419 w2425 w2439 w2473 w2481 w2493 w2502 w2524 w2564 w2628 w2642 w2697 w2750 w2765 w2776 w2793 w2803 w2807 w2833 w2843 w2847] -> w109
      tunnel: 30 ("Timeout") -> [w120 _ _ _ _ _ _ _ _ _ _ _ _ _ _ _ _ _ _ _ _ _ _ _ _ _ _ _ _ _ _ _ _ _ _ _ _ _ _ _ _ _ _ _ _ _ _ _ _ _ _ _ _ _ _ _ _ _ _ _ _ _ _ _ _ _ _ _ _ _ _ _ _ _ _ _ _ _ _ _ _ _ _ _ _ _ _ _ _ _ _ _ _ _ _ _ _ _ _ _ _ _ _ _ _ _ _ _ _ _ _ _ _ _ _ _ _ _ _ _ _ _ _ _ _ _ _ _ _ _ _ _ _ _ _ _ _ _ _ _ _ _ _]
      tunnel: w106 -> [w114 _ _ _ _ _ _ _ _ _ _ _ _ w620 _ _ _ _ w771 _ _ _ _ _ _ _ _ _ _ _ _ _ _ _ _ _ _ _ _ _ _ _ _ _ _ _ _ _ _ _ _ _ _ _ _ _ _ _ _ _ _ _ _ _ _ _ _ _ _ _ _ _ _ _ w1741 _ _ _ w1784 _ _ _ _ _ _ _ _ _ _ _ _ _ _ _ _ _ _ _ _ _ _ _ _ _ _ _ _ _ _ _ _ _ _ _ _ _ _ _ _ _ _ _ _ _ _ _ _ _ _ _ _ _ _ w2700 _ _ _ _ _ _ _ _ _]
      tunnel: w105 -> [_ _ _ _ _ _ _ _ _ _ _ _ w608 w629 _ _ _ w721 w777 _ _ _ _ _ _ _ _ _ _ _ _ _ _ _ _ _ _ _ _ _ _ _ _ _ _ _ _ _ _ _ _ _ _ _ _ _ _ _ _ _ _ _ _ _ _ _ _ _ _ _ _ _ _ _ _ w1752 _ w1772 w1783 _ _ _ _ _ _ _ _ _ _ _ _ _ _ _ _ _ _ _ _ _ _ _ _ _ _ _ _ _ _ _ _ _ _ _ _ _ _ _ _ _ _ _ _ _ _ _ _ _ _ _ _ _ _ _ _ _ _ _ _ _ _ _ _]
      tunnel: w104 -> [w119 _ _ _ _ _ _ _ _ _ _ _ _ _ _ _ _ _ _ _ _ _ _ _ _ _ _ _ _ _ _ _ _ _ _ _ _ _ _ _ _ _ w1207 _ _ _ _ _ _ _ _ _ _ _ _ _ _ _ _ _ _ _ _ _ _ _ _ _ _ _ _ _ _ _ _ _ _ _ _ _ _ _ _ _ _ _ _ _ _ _ _ _ _ _ _ _ _ _ _ _ _ _ _ _ _ _ _ _ _ _ _ _ _ _ _ _ _ _ _ _ _ _ _ _ _ _ _ _ _ _ _ _ _ _ _ _ _ _ _ _ _ _ _]
      tunnel: w103 -> [w118 w454 w464 w469 w477 w486 w496 w506 w527 w545 w566 w582 w609 w630 w645 w659 w688 w723 w778 w810 w815 w820 w825 w842 w859 w883 w888 w896 w908 w920 w933 w952 w976 w979 w989 w1006 w1036 w1086 w1109 w1132 w1155 w1181 w1211 w1245 w1259 w1265 w1279 w1292 w1303 w1319 w1357 w1374 w1382 w1422 w1425 w1437 w1446 w1455 w1473 w1506 w1530 w1543 w1560 w1571 w1582 w1596 w1608 w1621 w1634 w1650 w1678 w1684 w1696 w1707 w1744 w1756 w1764 w1773 w1782 w1791 w1798 w1805 w1822 w1840 w1856 w1882 w1902 w1905 w1913 w1921 w1926 w1935 w1975 w2015 w2029 w2042 w2055 w2073 w2079 w2091 w2103 w2122 w2126 w2138 w2205 w2218 w2230 w2254 w2274 w2282 w2288 w2302 w2351 w2356 w2362 w2368 w2374 w2382 w2391 w2401 w2407 w2413 w2418 w2424 w2438 w2472 w2480 w2492 w2515 w2537 w2563 w2629 w2646 w2701 w2749 w2764 w2775 w2799 w2802 w2826 w2832 w2842 w2846]
      tunnel: [w116 w454 w464 w469 w477 w486 w496 w506 w527 w545 w566 w582 w609 w630 w645 w659 w688 w723 w778 w810 w815 w820 w825 w842 w859 w883 w888 w896 w908 w920 w933 w952 w976 w979 w989 w1006 w1036 w1086 w1109 w1132 w1155 w1181 w1211 w1245 w1259 w1265 w1279 w1292 w1303 w1319 w1357 w1374 w1382 w1422 w1425 w1437 w1446 w1455 w1473 w1506 w1530 w1543 w1560 w1571 w1582 w1596 w1608 w1621 w1634 w1650 w1678 w1684 w1696 w1707 w1744 w1756 w1764 w1773 w1782 w1791 w1798 w1805 w1822 w1840 w1856 w1882 w1902 w1905 w1913 w1921 w1926 w1935 w1975 w2015 w2029 w2042 w2055 w2073 w2079 w2091 w2103 w2122 w2126 w2138 w2205 w2218 w2230 w2254 w2274 w2282 w2288 w2302 w2351 w2356 w2362 w2368 w2374 w2382 w2391 w2401 w2407 w2413 w2418 w2424 w2438 w2472 w2480 w2492 w2515 w2537 w2563 w2629 w2646 w2701 w2749 w2764 w2775 w2799 w2802 w2826 w2832 w2842 w2846] -> w102
      tunnel: w100 -> [_ _ _ _ _ _ _ _ _ _ _ _ _ _ _ _ _ _ _ _ _ _ _ _ _ _ _ _ _ _ _ _ _ _ _ _ _ _ _ _ _ _ _ _ _ _ _ _ _ _ _ _ _ _ _ _ _ _ _ _ _ _ _ _ _ _ _ _ _ _ _ _ _ _ _ _ _ _ w1781 _ _ _ _ _ _ _ _ _ _ _ _ _ _ _ _ _ _ _ _ _ _ _ _ _ _ _ _ _ _ _ _ _ _ _ _ _ _ _ _ _ _ _ _ _ _ _ _ _ _ _ _ _ _ _ _ _ _ _ _ _ _ _ _]
      tunnel: w95 -> [w117 _ _ _ _ _ _ _ _ _ _ _ _ _ _ _ _ _ _ _ _ _ _ _ _ _ _ _ _ _ _ _ _ _ _ _ _ _ _ _ _ _ _ _ _ _ _ _ _ _ _ _ _ _ _ _ _ _ _ _ _ _ _ _ _ _ _ _ _ _ _ _ _ w1706 w1743 _ _ _ _ _ _ _ _ _ _ _ _ _ _ _ _ _ _ _ _ _ _ _ _ _ _ _ _ _ _ _ _ _ _ _ _ _ _ _ _ _ _ _ _ _ _ _ _ _ _ _ _ _ _ _ _ _ _ _ _ _ w2773 _ _ _ _ _ _]
      tunnel: w94 -> [w115 _ _ _ _ _ _ _ _ _ _ _ w598 _ _ w657 _ w704 _ _ _ _ _ _ _ _ _ _ _ _ _ _ _ _ _ _ _ _ _ _ _ _ _ _ _ _ _ _ _ _ _ _ _ _ _ _ _ _ _ _ _ _ _ _ _ _ _ _ _ _ _ _ _ _ w1737 _ _ _ w1778 _ _ _ _ _ _ _ _ _ _ _ _ _ _ _ _ _ _ _ _ _ _ _ _ _ _ _ _ _ _ _ _ _ _ _ _ _ _ _ _ _ _ _ _ _ _ _ _ _ _ _ _ _ w2644 _ _ _ _ _ _ _ _ _ _]
      frame "", "Event Structure", "Idle" {
        # "executes when the state queue is empty"
        n52 = event shown="[14] \"AB Rep Rate\", \"Duty Cycle (%)\": Value Change" {
          selector: w118 -> [_ _ _ _ _ _ _ _ _ _ _ _ _ _ _ _ _ _ _ _ _ _ _ _ _ _ _ _ _ _ _ _ _ _ _ _]
          dyn-events: [_ _ _ _ _ _ _ _ _ _ _ _ _ _ _ _ _ _ _ _ _ _ _ _ _ _ _ _ _ _ _ _ _ _ _ _] -> w116
          timeout: w120 -> [_ _ _ _ _ _ _ _ _ _ _ _ _ _ _ _ _ _ _ _ _ _ _ _ _ _ _ _ _ _ _ _ _ _ _ _]
          tunnel: w126 -> [w142 w151 w160 w172 w180 w197 w210 w225 w232 w239 w252 w262 w267 w273 w289 w293 w297 w302 w306 w311 w324 w330 w335 w339 w343 w354 w361 w379 w396 w401 w408 w413 w421 w430 w444 w453]
          tunnel: [w143 w151 w159 w172 w179 w197 w209 w224 w232 w238 w252 w262 w266 w274 w288 w293 w298 w302 w307 w311 w325 w329 w335 w339 w342 w355 w360 w378 w396 w402 w407 w412 w421 w430 w444 w452] -> w125
          tunnel: w124 -> [w129 w149 w153 w174 w182 w196 w211 w223 w231 w235 w251 w261 w263 w275 w287 w291 w295 w300 w304 w309 w313 w331 w333 w337 w344 w353 w363 w380 w394 w403 w409 w414 w416 w425 w442 w450]
          tunnel: [w131 w150 w156 w175 w183 w195 w202 w222 w228 w241 w247 w257 w265 w268 w283 w292 w296 w301 w305 w310 w321 w332 w334 w338 w345 w356 w364 w381 w395 w398 w410 w415 w420 w423 w443 w451] -> w123
          tunnel: w122 -> [w131 w150 w161 w175 w183 w195 w203 w222 w229 w240 w246 w256 w265 w269 w284 w292 w296 w301 w305 w310 w323 w332 w334 w338 w345 w356 w364 w381 w395 w397 w410 w415 w420 w422 w443 w451]
          tunnel: [w129 w149 w153 w174 w182 w196 w211 w223 w231 w234 w251 w261 w263 w275 w287 w291 w295 w300 w304 w309 w312 w331 w333 w337 w344 w353 w363 w380 w394 w404 w409 w414 w416 w426 w442 w450] -> w121
          tunnel: w119 -> [_ _ _ _ _ _ _ _ _ _ _ _ _ _ _ _ _ _ _ _ _ _ _ _ _ _ _ _ _ _ _ _ _ _ _ _]
          tunnel: w117 -> [_ _ _ _ _ _ _ _ _ _ _ _ _ _ _ _ _ _ _ _ _ _ _ _ _ _ _ _ _ _ _ _ _ _ _ _]
          tunnel: w115 -> [_ _ _ _ _ _ _ _ _ _ _ _ _ _ _ _ _ _ _ _ _ _ _ _ _ _ _ _ _ _ _ _ _ w424 _ _]
          tunnel: w114 -> [_ _ _ _ _ _ _ _ _ _ _ _ _ _ _ _ _ _ _ _ _ _ _ _ _ _ _ _ _ w399 _ _ _ _ _ _]
          event Timeout {
            # "check system status every 2s"
            n53 = event-data() -> ()  [unwired: 1 in, 1 out]
            n54 = Unbundle By Name(w129) -> ("SlowTimer"=w127:u32, "FastTimer"=w128:u32)
            n55 = Tick Count (ms)() -> (millisecond timer value=w132:u32)
            n56 = Subtract(x=w132, y=w127) -> (x-y=w137:u32)
            n57 = Subtract(x=w132, y=w128) -> (x-y=w133:u32)
            n58 = Greater?(x=w137, y=u32 2000) -> (0:w138:bool)
            n59 = Greater?(x=w133, y=u32 500) -> (0:w135:bool)
            n60 = case shown="True" w138 {
              tunnel: ["" ("Empty String Constant") "SystemStatus: SlowSysStatusMacro" ("State(s) in Front (\"\")")] -> w139
              frame False {
              }
              frame True {
              }
            }
            n61 = case shown="True" w135 {
              tunnel: ["" ("Empty String Constant") "SystemStatus: FastSysStatusMacro" ("State(s) in Front (\"\")")] -> w134
              frame False {
              }
              frame True {
              }
            }
            n62 = call <vilib>:"Add State(s) to Queue__JKI_lib_State_Machine.vi"("State(s) in Front (\"\")"="LabJack: checkPedal\nData: SignInRange" ("State(s) in Front (\"\")"), "State(s) in (\"\")"=w139, "State(s) at Back (\"\")"=w134) -> ("States Out"=w130:string)  [unwired: 12 in]
            n63 = call <vilib>:"Add State(s) to Queue__JKI_lib_State_Machine.vi"("State(s) in Front (\"\")"=w130, "State(s) in (\"\")"=w142) -> ("States Out"=w143:string)  [unwired: 13 in]
          }
          event "355nm Laser toggle": Mouse Enter {
            n64 = event-data() -> ()  [unwired: 1 in, 4 out]
            n65 = local write "Help"("Toggle 355nm laser." ("Help")) -> ()
          }
          event "355nm Laser toggle": Value Change {
            n66 = event-data() -> ()  [unwired: 1 in, 6 out]
            n67 = case shown="True" "355nm Laser toggle" {
              tunnel: [0.0 ("Value") 1.0 ("Value")] -> w163
              frame False {
                n68 = property on="Laser Rep Rate" class="DigNum (strict)"("DisabledEnum"=T11."Enabled" ("Disabled")) -> ()  [unwired: 2 in, 2 out]
              }
              frame True {
                n69 = property on="Laser Rep Rate" class="DigNum (strict)"("DisabledEnum"=T11."Disabled and Grayed Out" ("Disabled")) -> ()  [unwired: 2 in, 2 out]
              }
            }
            n70 = Unbundle By Name(w153) -> ("LJ Pinout.355 PWM"=w152:string)
            n71 = call "LabJack_FGV.vi"("Operation(Read)"=enum16{"Write", "Read"}."Read" ("Operation"), "error in (no error)"=w161) -> ("error out"=w165:errorcluster, "Read data"=w166:i32)  [unwired: 8 in]
            n72 = Concatenate Strings(w152, "_EF_ENABLE" ("string")) -> (w162:string)
            n73 = call "LJM_eWriteName.vi"("Handle In"=w166, "Name"=w162, "Value"=w163, "error in"=w165) -> ("error out"=w157:errorcluster)  [unwired: 10 in, 1 out]
            n74 = call <vilib>:"Add State(s) to Queue__JKI_lib_State_Machine.vi"("State(s) in Front (\"\")"="/*355 Laser: CheckControllerStatus\n/*355 Laser: CheckPWMStatus" ("State(s) in Front (\"\")"), "State(s) in (\"\")"=w160) -> ("States Out"=w159:string)  [unwired: 13 in]
            n75 = call <userlib>:"Wait (ms)__ogtk.vi"("error in (no error)"=w157, "milliseconds to wait"=u32 50) -> ("error out"=w156:errorcluster)  [unwired: 8 in, 1 out]
          }
          event "Aiming beam toggle": Mouse Enter {
            n76 = event-data() -> ()  [unwired: 1 in, 4 out]
            n77 = local write "Help"("Toggle aiming beam laser." ("Help")) -> ()
          }
          event "Aiming beam toggle": Value Change {
            # "[Covers: REQ27]"
            n78 = event-data() -> ("NewVal"=w181:bool)  [unwired: 1 in, 5 out]
            n79 = local read "AB Rep Rate"() -> (w177:u16)
            n80 = Equal To 0?(x=w177) -> (x = 0?=w176:bool)
            n81 = case shown="False" w181 {
              tunnel: [w184 w191] -> w178
              tunnel: w176 -> [w187 w189]
              frame False {
                w188 = T11."Enabled" ("Disabled")
                n82 = Select(t="LabJack: AB_DC_Stop" ("State(s) in Front (\"\")"), s=w187, f="LabJack: AB_PWM_Stop" ("State(s) in Front (\"\")")) -> (s? t:f=w184:string)
                n83 = property on="Current" class="DigNum (strict)"("DisabledEnum"=w188) -> ()  [unwired: 2 in, 2 out]
                n84 = property on="AB Rep Rate" class="DigNum (strict)"("DisabledEnum"=w188) -> ()  [unwired: 2 in, 2 out]
              }
              frame True {
                w193 = T11."Disabled and Grayed Out" ("Disabled")
                n85 = Select(t="LabJack: AB_DC_Start" ("State(s) in Front (\"\")"), s=w189, f="LabJack: AB_PWM_Start" ("State(s) in Front (\"\")")) -> (s? t:f=w191:string)
                n86 = property on="AB Rep Rate" class="DigNum (strict)"("DisabledEnum"=w193) -> ()  [unwired: 2 in, 2 out]
                n87 = property on="Current" class="DigNum (strict)"("DisabledEnum"=w193) -> ()  [unwired: 2 in, 2 out]
              }
            }
            n88 = call <vilib>:"Add State(s) to Queue__JKI_lib_State_Machine.vi"("State(s) in Front (\"\")"=w178, "State(s) in (\"\")"=w180) -> ("States Out"=w179:string)  [unwired: 13 in]
          }
          event "Auto gain": Value Change {
            n89 = event-data() -> ("NewVal"=w194:bool)  [unwired: 1 in, 5 out]
            n90 = case shown="True" w194 {
              frame False {
                n91 = local read "Ctrl V"() -> (w198:dbl)
                n92 = call "V1FGV.vi"("action (write)"=enum16{"write", "read"}."write" ("action"), "V1 in"=w198) -> ()  [unwired: 8 in, 2 out]
                n93 = property on="Ctrl V" class="DigNum (strict)"("DisabledEnum"=T11."Enabled" ("Disabled")) -> ()  [unwired: 2 in, 2 out]
              }
              frame True {
                n94 = property on="Ctrl V" class="DigNum (strict)"("DisabledEnum"=T11."Disabled and Grayed Out" ("Disabled")) -> ()  [unwired: 2 in, 2 out]
              }
            }
          }
          event "Channel": Value Change {
            n95 = event-data() -> ("NewVal"=w207:enum32{"Ch1", "Ch2", "Ch3"})  [unwired: 1 in, 5 out]
            n96 = case shown="\"Ch3\"" w207 {
              tunnel: [w213 w215 w217] -> w206
              frame "Ch1", Default {
                n97 = local read "Ch1 Max CtrlV"() -> (w213:dbl)
                n98 = local write "Tab Control"(T12."APD1" ("Tab Control")) -> ()
              }
              frame "Ch2" {
                n99 = local read "Ch2 Max CtrlV"() -> (w215:dbl)
                n100 = local write "Tab Control"(T12."APD2" ("Tab Control")) -> ()
              }
              frame "Ch3" {
                n101 = local read "Ch3 Max CtrlV"() -> (w217:dbl)
                n102 = local write "Tab Control"(T12."APD3" ("Tab Control")) -> ()
              }
            }
            n103 = local write "Gain High"(w206) -> ()
            n104 = call "V1FGV.vi"("Error In"=w203, "action (write)"=enum16{"write", "read"}."write" ("action"), "V1 in"=0.0) -> ("Error Out"=w202:errorcluster)  [unwired: 7 in, 1 out]
            n105 = call <vilib>:"Add State(s) to Queue__JKI_lib_State_Machine.vi"("State(s) in Front (\"\")"="UI: Cursor Set >> Busy\nDigitizer: ConfigMacro\nUI: Cursor Set >> Idle" ("State(s) in Front (\"\")"), "State(s) in (\"\")"=w210) -> ("States Out"=w209:string)  [unwired: 13 in]
          }
          event "Task": Value Change {
            n106 = event-data() -> ("NewVal"=w221:enum32{"iRFAndGain", "Alignment"})  [unwired: 1 in, 5 out]
            n107 = case shown="\"iRFAndGain\", Default" w221 {
              tunnel: ["SysConfig: Load Digitizer Setting\nUI: Update" ("State(s) in Front (\"\")") "SysConfig: Load Digitizer Setting Gain\nUI: Update" ("State(s) in Front (\"\")")] -> w220
              frame "iRFAndGain", Default {
                # "load iRF setting"
              }
              frame "Alignment" {
                # "load gain setting"
              }
            }
            n108 = call <vilib>:"Add State(s) to Queue__JKI_lib_State_Machine.vi"("State(s) in Front (\"\")"=w220, "State(s) in (\"\")"="UI: Cursor Set >> Busy\nDigitizer: ConfigMacro\nUI: Cursor Set >> Idle" ("State(s) in Front (\"\")")) -> ("States Out"=w218:string)  [unwired: 13 in]
            n109 = call <vilib>:"Add State(s) to Queue__JKI_lib_State_Machine.vi"("State(s) in Front (\"\")"=w218, "State(s) in (\"\")"=w225) -> ("States Out"=w224:string)  [unwired: 13 in]
          }
          event "Waveform (no average)": Cursor Move {
            n110 = event-data() -> ()  [unwired: 1 in, 9 out]
            n111 = control-ref of="Waveform (no average)"() -> (w230:refnum<vi>)
            n112 = call "UpdateCurserIdx(SubVI).vi"("error in (no error)"=w229, "WaveformGraph in"=w230) -> ("error out"=w228:errorcluster)  [unwired: 9 in]
          }
          event "Current": Value Change {
            n113 = event-data() -> ()  [unwired: 1 in, 6 out]
            n114 = Unbundle By Name(w235) -> ("AB Cluster"=w236:T21)
            n115 = Bundle By Name(cluster=w236, "Default Current"="Current") -> (w233:T21)
            n116 = Bundle By Name(cluster=w235, "AB Cluster"=w233) -> (w234:T22)
            n117 = call "writeAimingBeamSetting.vi"("error in"=w240, "Aiming Beam Cluster"=w233) -> ("error out"=w241:errorcluster)  [unwired: 9 in]
            n118 = call <vilib>:"Add State(s) to Queue__JKI_lib_State_Machine.vi"("State(s) in Front (\"\")"="SysConfig: Load AB setting\n/*AimingBeam: Set Current" ("State(s) in Front (\"\")"), "State(s) in (\"\")"=w239) -> ("States Out"=w238:string)  [unwired: 13 in]
          }
          event "Ctrl V": Value Change; "Ctrl V": Key Down {
            n119 = event-data() -> ()  [unwired: 1 in, 4 out]
            n120 = local read "Channel"() -> (w249:enum32{"Ch1", "Ch2", "Ch3"})
            n121 = case shown="\"Ch3\"" w249 {
              tunnel: [enum16{"Ch1", "Ch2", "Ch3"}."Ch1" ("Enum") enum16{"Ch1", "Ch2", "Ch3"}."Ch2" ("Enum") enum16{"Ch1", "Ch2", "Ch3"}."Ch3" ("Enum")] -> w248
              frame "Ch1", Default {
              }
              frame "Ch2" {
              }
              frame "Ch3" {
              }
            }
            n122 = formula code="float32 y=0.05;\nif (x>0&&x<3.8)\ny=0.1;\nif (x>=3.8&&x<4.4)\ny=0.02;\nif (x>=4.4)\ny=0.01;"("x"="Ctrl V") -> ("y"=w243:sgl)
            n123 = call "CtrlVtoGain.vi"("error in (no error)"=w246, "CtrlV(V)"="Ctrl V", "Channel"=w248) -> ("error out"=w247:errorcluster, "Gain"=→"GainIndicator":dbl)  [unwired: 7 in]
            n124 = call "V1FGV.vi"("action (write)"=enum16{"write", "read"}."write" ("action"), "V1 in"="Ctrl V") -> ()  [unwired: 8 in, 2 out]
            n125 = property on="Ctrl V" class="DigNum (strict)"("Increment"=w243) -> ()  [unwired: 2 in, 2 out]
          }
          event "Save PID": Value Change {
            n126 = event-data() -> ()  [unwired: 1 in, 6 out]
            n127 = local read "Ch1 PID gains"() -> (w260:T6)
            n128 = local read "Ch2 PID gains"() -> (w259:T6)
            n129 = local read "Ch3 PID gains"() -> (w258:T6)
            n130 = call "writePIDSetting.vi"("Error In"=w256, "Ch3 PID gains"=w258, "Ch2 PID gains"=w259, "Ch1 PID gains"=w260) -> ("Error Out"=w257:errorcluster)  [unwired: 7 in]
          }
          event "Quit": Value Change {
            # "Exit Button Value Change (pressed) Event\n(when pressed.  quite)"
            n131 = event-data() -> ()  [unwired: 1 in, 1 out]
            n132 = call <vilib>:"Add State(s) to Queue__JKI_lib_State_Machine.vi"("State(s) in Front (\"\")"="LED: Off\nMacro: Exit", "State(s) in (\"\")"=w267) -> ("States Out"=w266:string)  [unwired: 13 in]
          }
          event "Laser Rep Rate": Value Change {
            n133 = event-data() -> ()  [unwired: 1 in, 6 out]
            n134 = call "LJ_calculate_PWM_parameters.vi"("Error In"=w269, "Laser Rep Rate (Hz)"="Laser Rep Rate", "Laser"=enum16{"355nm", "AimingBeam"}."355nm") -> ("Error Out"=w268:errorcluster)  [unwired: 7 in, 1 out]
            n135 = call <vilib>:"Add State(s) to Queue__JKI_lib_State_Machine.vi"("State(s) in Front (\"\")"="SysConfig: Load 355 PWM\nLabJack: 355_PWM_Config" ("State(s) in Front (\"\")"), "State(s) in (\"\")"=w273) -> ("States Out"=w274:string)  [unwired: 13 in]
          }
          event "AB Rep Rate", "Duty Cycle (%)": Value Change {
            n136 = event-data() -> ()  [unwired: 1 in, 6 out]
            n137 = Unbundle By Name(w287) -> ("AB Cluster"=w286:T21)
            n138 = Bundle By Name(cluster=w286, "Frequency(Hz)"="AB Rep Rate") -> (w285:T21)
            n139 = call "writeAimingBeamSetting.vi"("error in"=w284, "Aiming Beam Cluster"=w285) -> ("error out"=w283:errorcluster)  [unwired: 9 in]
            n140 = Equal To 0?(x="AB Rep Rate") -> (x = 0?=w281:bool)
            n141 = Select(t="", s=w281, f="AimingBeam: ComputePWM\nSysConfig: Load AB PWM\nLabJack: AB_PWM_Config" ("State(s) in Front (\"\")")) -> (s? t:f=w277:string)
            n142 = call <vilib>:"Add State(s) to Queue__JKI_lib_State_Machine.vi"("State(s) in Front (\"\")"="SysConfig: Load AB setting" ("State(s) in Front (\"\")"), "State(s) in (\"\")"=w277) -> ("States Out"=w276:string)  [unwired: 13 in]
            n143 = call <vilib>:"Add State(s) to Queue__JKI_lib_State_Machine.vi"("State(s) in Front (\"\")"=w276, "State(s) in (\"\")"=w289) -> ("States Out"=w288:string)  [unwired: 13 in]
          }
          event "StartButton": Mouse Enter {
            n144 = event-data() -> ()  [unwired: 1 in, 4 out]
            n145 = local write "Help"("Press to start aquisition." ("Help")) -> ()
          }
          event "StartButton": Value Change {
            # "Initialize both digitizer aquisition and\n send user event to trigger aquisition loop"
            n146 = event-data() -> ()  [unwired: 1 in, 6 out]
            n147 = call <vilib>:"Add State(s) to Queue__JKI_lib_State_Machine.vi"("State(s) in Front (\"\")"="Macro: StartRun" ("State(s) in Front (\"\")"), "State(s) in (\"\")"=w297) -> ("States Out"=w298:string)  [unwired: 13 in]
          }
          event "StopButton": Mouse Enter {
            n148 = event-data() -> ()  [unwired: 1 in, 4 out]
            n149 = local write "Help"("Press to stop data aquisition." ("Help")) -> ()
          }
          event "StopButton": Value Change {
            n150 = event-data() -> ()  [unwired: 1 in, 6 out]
            n151 = call <vilib>:"Add State(s) to Queue__JKI_lib_State_Machine.vi"("State(s) in Front (\"\")"="Macro: StopRun" ("State(s) in Front (\"\")"), "State(s) in (\"\")"=w306) -> ("States Out"=w307:string)  [unwired: 13 in]
          }
          event "Sys Reconfig": Mouse Enter {
            n152 = event-data() -> ()  [unwired: 1 in, 4 out]
            n153 = local write "Help"("Click to reconfig digitizer settings." ("Help")) -> ()
          }
          event "Sys Reconfig": Value Change {
            # "everytime the user change data aquisition setting, need to reinitilize decon engine and realign iRF.\ncheck whether data length has changed, if changed, reinitialize Decon engine\nreset BG ready, need a new BG"
            # "update DAQ FGV"
            n154 = event-data() -> ()  [unwired: 1 in, 6 out]
            n155 = call "SystemConfigEditorV6.vi"("error in"=w323) -> ("error out"=w322:errorcluster, "FLImDAQ out"=w319:T4)  [unwired: 1 in]
            n156 = Unbundle By Name(w313) -> ("FLImDAQ.min record length"=w314:i32)
            n157 = Unbundle By Name(w319) -> ("min record length"=w320:i32)
            n158 = call "FLImDAQ_FGV.vi"("error in (no error)"=w322, "Operation (Read)"=enum16{"Write", "Read"}."Write" ("Operation"), "Write data"=w319) -> ("error out"=w321:errorcluster, "Read data"=w318:T4)  [unwired: 7 in]
            n159 = Equal?(x=w314, y=w320) -> (x = y?=w317:bool)
            n160 = case shown="False" w317 {
              tunnel: ["UI: Cursor Set >> Busy\nDigitizer: ConfigMacro\n/*UI: CaliAndiRFNotReady\n/*UI iRF not ready\nUI: Update\nUI: Cursor Set >> Idle" "UI: Cursor Set >> Busy\nDigitizer: ConfigCh3iRF\nUI: Update\nUI: Cursor Set >> Idle"] -> w316
              frame False {
              }
              frame True {
              }
            }
            n161 = Bundle By Name(cluster=w313, "FLImDAQ"=w318) -> (w312:T22)
            n162 = call <vilib>:"Add State(s) to Queue__JKI_lib_State_Machine.vi"("State(s) in Front (\"\")"=w316, "State(s) in (\"\")"=w324) -> ("States Out"=w325:string)  [unwired: 13 in]
          }
          event "Clear WF Chart History": Value Change {
            n163 = event-data() -> ()  [unwired: 1 in, 6 out]
            n164 = call <vilib>:"Add State(s) to Queue__JKI_lib_State_Machine.vi"("State(s) in Front (\"\")"="Graph: ClearHistory" ("State(s) in Front (\"\")"), "State(s) in (\"\")"=w330) -> ("States Out"=w329:string)  [unwired: 13 in]
          }
          event "System Hardware Connection Status", "StartButton", "StopButton", "355nm Laser toggle", "Aiming beam toggle", "Sys Reconfig": Mouse Leave {
            n165 = event-data() -> ()  [unwired: 1 in, 4 out]
            n166 = invoke on="Help" class="Str" method="Reinit To Default"() -> ()  [unwired: 3 in, 3 out]
          }
          event "System Hardware Connection Status.Digitizer": Mouse Enter {
            n167 = event-data() -> ()  [unwired: 1 in, 4 out]
            n168 = local write "Help"("Status of hardware connections. TCP/IP is optional." ("Help")) -> ()
          }
          event "TCP Connect": Value Change {
            n169 = event-data() -> ("NewVal"=w340:bool)  [unwired: 1 in, 5 out]
            n170 = case shown="False" w340 {
              tunnel: ["UI: Update" ("State(s) in Front (\"\")") "UI: Update" ("State(s) in Front (\"\")")] -> w341
              frame False {
              }
              frame True {
              }
            }
            n171 = call <vilib>:"Add State(s) to Queue__JKI_lib_State_Machine.vi"("State(s) in Front (\"\")"=w341, "State(s) in (\"\")"=w343) -> ("States Out"=w342:string)  [unwired: 13 in]
          }
          event User Event {
            # "if aquisition loop is error out. Stop digitizer, flash queue, update front panel indicator, stop both laser and parse and save data"
            n172 = event-data() -> ()  [unwired: 1 in, 5 out]
            n173 = case shown="True" FALSE {
              tunnel: ["" ("Empty String Constant") "Data: parseRunDataMacro" ("State(s) in Front (\"\")")] -> w351
              frame False {
                # "if flag is 0, do not save data"
              }
              frame True {
                # "if save data flag is true enqueue data"
              }
            }
            n174 = call <vilib>:"Add State(s) to Queue__JKI_lib_State_Machine.vi"("State(s) in Front (\"\")"="Digitizer: Abort\nLabJack: ZeroV" ("State(s) in Front (\"\")"), "State(s) in (\"\")"=w351, "State(s) at Back (\"\")"="LED: BreathOff\nMacro: SysReadyForAqui\nUI: Update" ("State(s) in Front (\"\")")) -> ("States Out"=w352:string)  [unwired: 12 in]
            n175 = call <vilib>:"Add State(s) to Queue__JKI_lib_State_Machine.vi"("State(s) in Front (\"\")"=w352, "State(s) in (\"\")"=w354) -> ("States Out"=w355:string)  [unwired: 13 in]
          }
          event "AcquireGain": Value Change {
            n176 = event-data() -> ()  [unwired: 1 in, 6 out]
            n177 = local read "GainSigInRange"() -> (w362:bool)
            n178 = case shown="True" w362 {
              tunnel: ["" ("State(s) in Front (\"\")") w367] -> w359
              frame False {
                n179 = One Button Dialog(message="Please make sure peak voltage is with in 0.3V to 1.4V and try again!") -> ()  [unwired: 1 in, 1 out]
              }
              frame True {
                n180 = local read "Laser Rep Rate"() -> (w371:u16)
                n181 = In Range and Coerce(upper limit=u16 500, x=w371, lower limit=u16 50) -> (In Range?=w368:bool)  [unwired: 1 out]
                n182 = case shown="True" w368 {
                  tunnel: ["" ("State(s) in Front (\"\")") "UI: Cursor Set >> Busy\nUtility: EnableGain? >> False\nUtility: setSaveFlag >> 0\nQueue: Flash\nUtility: setSaveFlag >> 1\nQueue: CheckNumOfWF\nData: parseSingleGainData\nUI: UpdateGainDataIndicators\nUtility: EnableGain? >> True\nUI: Cursor Set >> Idle\n" ("State(s) in Front (\"\")")] -> w367
                  frame False {
                    n183 = One Button Dialog(message="Please set 355nm laser rep rate between 20 and 250Hz ") -> ()  [unwired: 1 in, 1 out]
                  }
                  frame True {
                    n184 = local write "Num WF to acquire"(500) -> ()
                  }
                }
              }
            }
            n185 = call <vilib>:"Add State(s) to Queue__JKI_lib_State_Machine.vi"("State(s) in Front (\"\")"=w359, "State(s) in (\"\")"=w361) -> ("States Out"=w360:string)  [unwired: 13 in]
          }
          event "AcquireIRF": Value Change {
            n186 = event-data() -> ()  [unwired: 1 in, 6 out]
            n187 = local read "iRFSigInRange"() -> (w376:bool)
            n188 = case shown="True" w376 {
              tunnel: ["" ("State(s) in Front (\"\")") w384] -> w377
              frame False {
                n189 = One Button Dialog(message="Please make sure peak voltage is with in 0.5V to 1.4V and try again!") -> ()  [unwired: 1 in, 1 out]
              }
              frame True {
                n190 = local read "Laser Rep Rate"() -> (w388:u16)
                n191 = In Range and Coerce(upper limit=u16 500, x=w388, lower limit=u16 20) -> (In Range?=w385:bool)  [unwired: 1 out]
                n192 = case shown="True" w385 {
                  tunnel: ["" ("State(s) in Front (\"\")") "UI: Cursor Set >> Busy\nUtility: EnableGain? >> False\nUtility: setSaveFlag >> 0\nQueue: Flash\nUtility: setSaveFlag >> 1\nQueue: CheckNumOfWF\nData: parseIRFSingleIRFData\nUI: UpdateIRFDataTable\nUtility: EnableGain? >> True\nUI: Cursor Set >> Idle\n" ("State(s) in Front (\"\")")] -> w384
                  frame False {
                    n193 = One Button Dialog(message="Please set 355nm laser rep rate between 20 and 200Hz ") -> ()  [unwired: 1 in, 1 out]
                  }
                  frame True {
                    n194 = local write "Num WF to acquire"(500) -> ()
                  }
                }
              }
            }
            n195 = call <vilib>:"Add State(s) to Queue__JKI_lib_State_Machine.vi"("State(s) in Front (\"\")"=w377, "State(s) in (\"\")"=w379) -> ("States Out"=w378:string)  [unwired: 13 in]
          }
          event "Tab Control": Value Change {
            n196 = event-data() -> ()  [unwired: 1 in, 6 out]
            n197 = case shown="\"Data parsing\"" "Tab Control" {
              frame "APD1", Default {
              }
              frame "APD2" {
              }
              frame "APD3" {
              }
              frame "Debug" {
              }
              frame "IO Ststus" {
              }
              frame "LJ pinout" {
              }
              frame "Digitizer Info" {
              }
              frame "Data parsing" {
              }
              frame "Intensity Trace" {
              }
              frame "iRF Measureement" {
              }
              frame "Gain Measurement" {
              }
            }
          }
          event "ClearIRFData": Value Change {
            n198 = event-data() -> ()  [unwired: 1 in, 6 out]
            n199 = Bundle By Name(cluster=w403, "iRFIdx"=0) -> (w404:T22)
            n200 = Flush Queue(queue=w399, error in (no error)=w397) -> (error out=w398:errorcluster)  [unwired: 2 out]
            n201 = call <vilib>:"Add State(s) to Queue__JKI_lib_State_Machine.vi"("State(s) in Front (\"\")"="UI: InitIRFDataTable" ("State(s) in Front (\"\")"), "State(s) in (\"\")"=w401) -> ("States Out"=w402:string)  [unwired: 13 in]
          }
          event "SaveGainData": Value Change {
            n202 = event-data() -> ()  [unwired: 1 in, 6 out]
            n203 = call <vilib>:"Add State(s) to Queue__JKI_lib_State_Machine.vi"("State(s) in Front (\"\")"="UI: Cursor Set >> Busy\nAPD: LoadFromSerial\nAPD: writeGain\nFile: BackupOld\nAPD: SaveNew\nAPD: LoadFromSerialNoRawData\nUI: Cursor Set >> Idle" ("State(s) in Front (\"\")"), "State(s) in (\"\")"=w408) -> ("States Out"=w407:string)  [unwired: 13 in]
          }
          event "SaveiRFData": Value Change {
            n204 = event-data() -> ()  [unwired: 1 in, 6 out]
            n205 = call <vilib>:"Add State(s) to Queue__JKI_lib_State_Machine.vi"("State(s) in Front (\"\")"="UI: Cursor Set >> Busy\nAPD: LoadFromSerial\nAPD: writeiRF\nFile: BackupOld\nAPD: SaveNew\nAPD: LoadFromSerialNoRawData\nUI: Cursor Set >> Idle" ("State(s) in Front (\"\")"), "State(s) in (\"\")"=w413) -> ("States Out"=w412:string)  [unwired: 13 in]
          }
          event "SetIRFCtrlV": Value Change {
            # "set iRF V"
            n206 = event-data() -> ()  [unwired: 1 in, 6 out]
            n207 = local read "iRFCtrlV"() -> (w419:dbl[])
            n208 = Unbundle By Name(w416) -> ("iRFIdx"=w417:i32)
            n209 = Index Array(array=w419, index=w417) -> (element=w418:dbl)
            n210 = property on="Ctrl V" class="DigNum (strict)"("Val(Sgnl)"=w418) -> ()  [unwired: 2 in, 2 out]
          }
          event "ClearGainData": Value Change {
            w429 = dbl[] [] ("Gain")
            n211 = event-data() -> ()  [unwired: 1 in, 6 out]
            n212 = Flush Queue(queue=w424, error in (no error)=w422) -> (error out=w423:errorcluster)  [unwired: 2 out]
            n213 = local write "GainDataTable"(string[][] [] ("Table Control")) -> ()
            n214 = Bundle By Name(cluster=w425, "GainDataTemp"=T13 {"CtrlV"=-1.0, "PeakV"=0.0, "PeakV Std"=0.0, "IntFactor"=1.0, "IntCorrPeakV"=0.0}) -> (w426:T22)
            n215 = local write "Gain"(w429) -> ()
            n216 = local write "Ctrl V"(w429) -> ()
            n217 = local write "Intensity Factor"(w429) -> ()
            n218 = local write "AUC Std"(w429) -> ()
            n219 = local write "AUC"(w429) -> ()
            n220 = local write "Int Corr AUC"(w429) -> ()
          }
          event "ComputeGain": Value Change {
            # "Devide Int corrected Peak V by the 1st element"
            n221 = event-data() -> ()  [unwired: 1 in, 6 out]
            n222 = local read "Int Corr AUC"() -> (w441:dbl[])
            n223 = local read "Ctrl V"() -> (w433:dbl[])
            n224 = Reverse 1D Array(array=w441) -> (reversed array=w440:dbl[])
            n225 = Index Array(array=w440, index=0) -> (element=w438:dbl)
            n226 = local read "GainDataTable"() -> (w437:string[][])
            n227 = Divide(x=w441, y=w438) -> (x/y=w432:dbl[])
            "Gain" <- w432
            n228 = Bundle("Ctrl V"=w433, w432) -> (→"XY Graph":cluster{"Ctrl V":dbl[], dbl[]})  [unwired: 1 in]
            n229 = for {
              tunnel: w432 -> [w447] mode=indexing
              tunnel: [w445] -> w435 mode=indexing
              n230 = Number To Fractional String(number=w447, precision (6)=i16 3) -> (F-format string=w445:string)  [unwired: 2 in]
            }
            n231 = Insert Into Array(array=w437, index (col)=5 ("disabled index (col)"), new element=w435) -> (w434:string[][])  [unwired: 1 in]
            n232 = local write "GainDataTable"(w434) -> ()
          }
          event Panel Close? {
            # "Discard the event because we'll close the front panel ourselves in Macro: Exit"
            # "Close Panel button (pressed) Event\n(this executes Macro: Exit to terminate the VI)"
            n233 = event-data() -> ()  [unwired: 1 in, 1 out]
            n234 = event-data ("Event Filter Node")("Discard?"=TRUE) -> ()  [unwired: 1 in, 1 out]
            n235 = call <vilib>:"Add State(s) to Queue__JKI_lib_State_Machine.vi"("State(s) in Front (\"\")"="Macro: Exit", "State(s) in (\"\")"=w453) -> ("States Out"=w452:string)  [unwired: 13 in]
          }
        }
      }
      frame "---------- Macro ----------" {
        # "Do not put any code in this frame.\n(It is a separator no-op. You can make a copy of this frame to create a new Macro frame)"
        n236 = call <vilib>:"Add State(s) to Queue__JKI_lib_State_Machine.vi"("State(s) in (\"\")"=w458) -> ("States Out"=w457:string)  [unwired: 14 in]
      }
      frame "Macro: Initialize" {
        w460 = "Digitizer: Initialize\nDigitizer: ConfigMacro\nUI: Update\n/*AimingBeam: Initialize\n/*AimingBeam: Set Status>>Enable\n/*AimingBeam: Set Current\nUI: Update\nUI: Update\n355 Laser: Check Dewelling\nUtility: SetDefaultMaxV\nUI: InitIRFDataTable\nPID: loadPID\nUI: Cursor Set >> Idle\nLED: BreathOff\nMacro: SysReadyForAqui"  # Digitizer: Initialize Digitizer: ConfigMacro UI: Update /*AimingBeam: Initialize /*AimingBeam: Set Status>>Enable /*AimingBeam: Set Current UI: Update UI: Update 355 Laser: Check Dewelling Utility: SetDefaultMaxV UI: InitIRFDataTable PID: loadPID UI: Cursor Set >> Idle LED: BreathOff Macro: SysReadyForAqui
        # "load Labjack setting 1st as it contaisn laser pin infortmation"
        # "start laser 1st, need 7.5s for laser to get ready"
        # "Initialization Macro\n(This is called once, when the VI starts)"
        n237 = call <vilib>:"Add State(s) to Queue__JKI_lib_State_Machine.vi"("State(s) in Front (\"\")"="UI: showDisclaimer\nUI: Cursor Set >> Busy\nGraph: AddCursors\nData: Initialize\nInitialize Core Data\nUI: Initialize\nUI: Front Panel State >> Open\nUI: Update\nAPD: Initialize\nMacro: LoadSysConfig\nLabJack: Open\nLabJack: SetDefaultSub\nLED: OpenVIRef\nLED: BreathOrange\nUI: Update\n355 Laser: CheckControllerStatus\n355 Laser: Laser enable\n355 Laser: Dewelling>>5000\n355 Laser: CheckControllerStatus\nUI: Update\nLabJack: 355_PWM_Config\nLabJack: AB_PWM_Config\nUI: Update", "State(s) in (\"\")"=w460) -> ("States Out"=w459:string)  [unwired: 13 in]
        n238 = call <vilib>:"Add State(s) to Queue__JKI_lib_State_Machine.vi"("State(s) in Front (\"\")"=w459, "State(s) in (\"\")"=w467) -> ("States Out"=w466:string)  [unwired: 13 in]
        "Help" <- "Hover over controls to see help!" ("Help")
      }
      frame "Macro: LoadSysConfig" {
        # "System configuration Macro\n(Load configurations for different component of the system)"
        n239 = call <vilib>:"Add State(s) to Queue__JKI_lib_State_Machine.vi"("State(s) in Front (\"\")"="SysConfig: Load Digitizer Setting\nSysConfig: Load AB setting\nSysConfig: Load LJ Pinout\nSysConfig: Load 355 PWM\nSysConfig: Load APD Info", "State(s) in (\"\")"=w473) -> ("States Out"=w472:string)  [unwired: 13 in]
      }
      frame "Macro: StartRun" {
        # "start PWM before acquisition"
        # "Start Run Macro\n(Macro to start a aquisition run)"
        n240 = local read "Task"() -> (w475:enum32{"iRFAndGain", "Alignment"})
        n241 = case shown="\"iRFAndGain\", Default" w475 {
          tunnel: ["UI: Update\nLabJack: 355_PWM_Start\nLabJack: SetV\nDigitizer: Start\nUI: DuringAquisition\nLED: BreathGreen\nUI: Update" "UI: Update\nLabJack: SetV\nUtility: Dewelling >>250\nDigitizer: Start\nUI: DuringAquisition\nLED: BreathGreen\nUI: Update"] -> w474
          frame "iRFAndGain", Default {
          }
          frame "Alignment" {
          }
        }
        n242 = call <vilib>:"Add State(s) to Queue__JKI_lib_State_Machine.vi"("State(s) in Front (\"\")"=w474, "State(s) in (\"\")"=w480) -> ("States Out"=w479:string)  [unwired: 13 in]
      }
      frame "Macro: StopRun" {
        # "if system is running, send stop command, if not do nothing."
        # "stop aquisition\nupdate UI"
        # "Do not put any code in this frame.\n(It is a separator no-op. You can make a copy of this frame to create a new Macro frame)"
        n243 = Unbundle By Name(w483) -> ("SysRunning?"=w484:bool)
        n244 = case shown="True" w484 {
          tunnel: ["" ("Empty String Constant") w491] -> w485
          frame False {
          }
          frame True {
            n245 = local read "Task"() -> (w492:enum32{"iRFAndGain", "Alignment"})
            n246 = case shown="\"Alignment\"" w492 {
              tunnel: ["LabJack: 355_PWM_Stop" ("State(s) in Front (\"\")") "Digitizer: Abort" ("State(s) in Front (\"\")")] -> w491
              frame "iRFAndGain", Default {
                # "stop laser if taken iRF"
              }
              frame "Alignment" {
                # "do nothing if take gain"
              }
            }
          }
        }
        n247 = call <vilib>:"Add State(s) to Queue__JKI_lib_State_Machine.vi"("State(s) in Front (\"\")"=w485, "State(s) in (\"\")"=w489) -> ("States Out"=w488:string)  [unwired: 13 in]
      }
      frame "Macro: SysReadyForAqui" {
        # "System ready for aquisition macro.\n(Set UI and LED)"
        n248 = call <vilib>:"Add State(s) to Queue__JKI_lib_State_Machine.vi"("State(s) in Front (\"\")"="UI: ReadyForAquisition\nLED: Green" ("State(s) in Front (\"\")"), "State(s) in (\"\")"=w500) -> ("States Out"=w499:string)  [unwired: 13 in]
      }
      frame "Macro: AskOverWrite" {
        # "Ask user whther to over write existing APD data\n(It is a separator no-op. You can make a copy of this frame to create a new Data frame)"
        n249 = Two Button Dialog(message="Do you want to save new data? old file will be renamed as backup.", 2:"Save" ("T button name (\"OK\")")) -> (T button?=w503:bool)  [unwired: 1 in]
        n250 = case shown="True" w503 {
          tunnel: ["" ("Empty String Constant") "File: BackupOld\nAPD: SaveNew" ("State(s) in Front (\"\")")] -> w502
          frame False {
          }
          frame True {
            # "backup old file and save new file"
          }
        }
        n251 = call <vilib>:"Add State(s) to Queue__JKI_lib_State_Machine.vi"("State(s) in Front (\"\")"=w502, "State(s) in (\"\")"=w509) -> ("States Out"=w508:string)  [unwired: 13 in]
      }
      frame "Macro: Exit" {
        # "close LJ last"
        # "check whether hardware is initilized, if so close, if not do nothing"
        # "Exit Macro, close all hardware\n(This is called once, when the VI exits)"
        n252 = Unbundle By Name(w518) -> ("System Status.TCP/IP"=w517:bool, "System Status.Digitizer"=w516:bool, "System Status.Aiming Beam"=w515:bool, "System Status.355 Laser"=w514:bool, "System Status.Labjack"=w513:bool, "Core.Close Panel on Exit?"=w512:bool)
        n253 = case shown="True" w517 {
          tunnel: ["" ("Empty String Constant") ""] -> w525
          frame False {
          }
          frame True {
          }
        }
        n254 = case shown="True" w516 {
          tunnel: ["" ("Empty String Constant") "Digitizer: Close"] -> w526
          frame False {
          }
          frame True {
          }
        }
        n255 = case shown="True" w513 {
          tunnel: ["" ("Empty String Constant") "LabJack: SetDefaultAndClose"] -> w519
          frame False {
          }
          frame True {
          }
        }
        n256 = case shown="True" w515 {
          tunnel: ["" ("Empty String Constant") w540] -> w521
          frame False {
          }
          frame True {
            w540 = "/*AimingBeam: Set Status >> Disable\n/*AimingBeam: Close"  # /*AimingBeam: Set Status >> Disable /*AimingBeam: Close
          }
        }
        n257 = case shown="True" w514 {
          tunnel: ["" ("Empty String Constant") "355 Laser: Close\n355 Laser: CheckControllerStatus"] -> w520
          frame False {
          }
          frame True {
          }
        }
        n258 = Select(t="UI: Front Panel State >> Close", s=w512, f="" ("Empty String Constant")) -> (s? t:f=w522:string)
        n259 = call <vilib>:"Add State(s) to Queue__JKI_lib_State_Machine.vi"("State(s) in Front (\"\")"=w525, "State(s) in (\"\")"=w526, "State(s) at Back (\"\")"=w521) -> ("States Out"=w528:string)  [unwired: 12 in]
        n260 = call <vilib>:"Add State(s) to Queue__JKI_lib_State_Machine.vi"("State(s) in Front (\"\")"=w528, "State(s) in (\"\")"=w520, "State(s) at Back (\"\")"=w519) -> ("States Out"=w524:string)  [unwired: 12 in]
        n261 = call <vilib>:"Add State(s) to Queue__JKI_lib_State_Machine.vi"("State(s) in Front (\"\")"=w524, "State(s) in (\"\")"="UI: Update\nLED: CloseVIRef\nQueue: Destory\nData: Cleanup\nExit", "State(s) at Back (\"\")"=w522) -> ("States Out"=w529:string)  [unwired: 12 in]
        n262 = call <vilib>:"Add State(s) to Queue__JKI_lib_State_Machine.vi"("State(s) in Front (\"\")"=w529, "State(s) in (\"\")"=w534) -> ("States Out"=w533:string)  [unwired: 13 in]
      }
      frame "---------- Data ----------" {
        # "Template Separator\n(You can make a copy of, or modify, this frame)"
        n263 = call <vilib>:"Add State(s) to Queue__JKI_lib_State_Machine.vi"("State(s) in (\"\")"=w549) -> ("States Out"=w548:string)  [unwired: 14 in]
      }
      frame "Data: Initialize" {
        w552 = 0  # iRFIdx
        w554 = T23 {"CtrlV"=-1.0, "AUC"=0.0, "AUC Std"=0.0, "IntFactor"=1.0, "IntCorrAUC"=0.0}  # GainDataTemp
        w555 = dbl[][] []  # GainBGRaw
        w557 = FALSE  # LedViRefOpen
        w553 = T24 {"Ch1Serial"="", "Ch2Serial"="", "Ch3Serial"=""}  # APDSerials
        w558 = cluster{"RunID":i8, "BG ID":i8, "Cali ID":i8} {"RunID"=1, "BG ID"=1, "Cali ID"=1}  # IDs
        w559 = refnum<vi> refnum  # LED vi reference
        w560 = path ""  # TempPath
        w561 = T25 {"DataPath"=path "", "BG Path"=path "", "iRFPath"=path "", "CaliPath"=path ""}  # Pathes
        w562 = u32 0  # FastTimer
        w563 = u32 0  # SlowTimer
        w564 = dbl[][] []  # iRFAllGain
        w567 = T1 {"Digitizer"=FALSE, "Labjack"=FALSE, "Aiming Beam"=FALSE, "355 Laser"=FALSE, "TCP/IP"=FALSE}  # System Status
        w551 = T26 {"DIO_EF_CLOCK1_DIVISOR"=16, "DIO_EF_CLOCK1_ROLL_VALUE"=25000, "DIO#_EF_INDEX"=0, "DIO#_EF_OPTIONS"=1, "DIO#_EF_CONFIG_A"=6250}  # AB PWM setting
        w568 = T3 {"Ch1 Bias"="TDA11", "Ch2 Bias"="DAC10", "Ch3 Bias"="DAC0", "Ch4 Bias"="DAC0", "355 PWM"="FIO0", "AimingBeam PWM"="FIO2", "Laser Ready"="FIO3", "Interlock"="FIO1", "Laser Start/Stop"="FIO1", "Red LED"="FIO1", "Green LED"="FIO1", "Foot Pedal"="DIO15"}  # LJ Pinout
        w569 = 0  # TCP attempt count
        w550 = u32 0  # Laser start tic
        w570 = refnum<k20>[] []  # niTClk sessions
        w571 = u32 0  # Last Trigger
        w572 = T26 {"DIO_EF_CLOCK1_DIVISOR"=16, "DIO_EF_CLOCK1_ROLL_VALUE"=25000, "DIO#_EF_INDEX"=0, "DIO#_EF_OPTIONS"=1, "DIO#_EF_CONFIG_A"=6250}  # 355 PWM setting
        w573 = T21 {"Aiming Beam COM Port"="COM3", "Min Current"=0.0, "Max Current"=63.0, "Default Current"=20.0, "Frequency(Hz)"=0}  # AB Cluster
        w574 = T27 {"resource name"="", "resource name 2"="", "Channel"=enum."Channel 0", "trigger source"="VAL_EXTERNAL", "trigger level"=0.5, "trigger delay"=1.35e-07, "min sample rate"=12500000000.0, "min record length"=2500, "vertical range"=1.0, "vertical offset"=-0.25, "Waveform to Avg"=2000}  # FLImDAQ
        w575 = FALSE  # SysRunning?
        w565 = path ""  # DefaultPath
        w576 = T28 {"Ch1Enable?"=FALSE, "Ch2Enable?"=FALSE, "Ch3Enable?"=FALSE, "Ch1AutoGain?"=FALSE, "Ch2AutoGain?"=FALSE, "Ch3AutoGain?"=FALSE, "AimingBeamEnable?"=FALSE}  # SysConfigCluster
        w577 = T29 {"Current VI Reference"=refnum, "Close Panel on Exit?"=FALSE}  # Core
        # "Initialize the shift-register data, here.\n(data names are defined by what you wire into the bundle function)"
        n264 = call <vilib>:"Add State(s) to Queue__JKI_lib_State_Machine.vi"("State(s) in (\"\")"=w580) -> ("States Out"=w579:string)  [unwired: 14 in]
        n265 = Bundle("Core"=w577, "SysConfigCluster"=w576, "System Status"=w567, "IDs"=w558, "DefaultPath"=w565, "Pathes"=w561, "FLImDAQ"=w574, "SysRunning?"=w575, "AB Cluster"=w573, "LJ Pinout"=w568, "355 PWM setting"=w572, "AB PWM setting"=w551, "Last Trigger"=w571, "niTClk sessions"=w570, "Laser start tic"=w550, "TCP attempt count"=w569, "iRFAllGain"=w564, "SlowTimer"=w563, "FastTimer"=w562, "TempPath"=w560, "LED vi reference"=w559, "APDSerials"=w553, "LedViRefOpen"=w557, "GainBGRaw"=w555, "GainDataTemp"=w554, "iRFIdx"=w552) -> (w556:T22)  [unwired: 1 in]
      }
      frame "Data: SignInRange" {
        # "Check Whether Signal is in Range.\n(It is a separator no-op. You can make a copy of this frame to create a new Data frame)"
        n266 = local read "Task"() -> (w581:enum32{"iRFAndGain", "Alignment"})
        n267 = case shown="\"iRFAndGain\", Default" w581 {
          frame "iRFAndGain", Default {
            n268 = local read "Tab Control"() -> (w589:T2)
            n269 = case shown="\"iRF Measureement\"" w589 {
              tunnel: 1.4 ("upper limit") -> [_ w591 w595]
              tunnel: 0.1 ("lower limit") -> [_ w590 w594]
              frame "APD1", Default {
              }
              frame "Gain Measurement" {
                n270 = local read "WF max value"() -> (w593:dbl)
                n271 = In Range and Coerce(upper limit=w591, x=w593, lower limit=w590) -> (In Range?=→"GainSigInRange":bool)  [unwired: 1 out]
              }
              frame "iRF Measureement" {
                n272 = local read "WF max value"() -> (w597:dbl)
                n273 = In Range and Coerce(upper limit=w595, x=w597, lower limit=w594) -> (In Range?=→"iRFSigInRange":bool)  [unwired: 1 out]
              }
            }
          }
          frame "Alignment" {
          }
        }
        n274 = call <vilib>:"Add State(s) to Queue__JKI_lib_State_Machine.vi"("State(s) in (\"\")"=w586) -> ("States Out"=w585:string)  [unwired: 14 in]
      }
      frame "Data: parseRunDataGain" {
        w600 = cluster{"CtrlV":dbl, "WFs":dbl[][]} {"CtrlV"=0.0, "WFs"=[]}  # GainAllCluster
        # "data individual gian"
        # "Flash data from queue and save it in structure\n()"
        n275 = Flush Queue(queue=w608, error in (no error)=w606) -> (remaining elements=w607:cluster{"WF":dbl[][]}[], error out=w602:errorcluster)  [unwired: 1 out]
        n276 = for {
          tunnel: w607 -> [w613] mode=indexing
          tunnel: [w612] -> w599 mode=concatenating
          n277 = Unbundle By Name(w613) -> ("WF"=w612:dbl[][])
        }
        n278 = local read "Ctrl V"() -> (w604:dbl)
        n279 = Bundle By Name(cluster=w600, "CtrlV"=w604, "WFs"=w599) -> (w603:cluster{"CtrlV":dbl, "WFs":dbl[][]})
        n280 = Enqueue Element(queue=w598, element=w603, error in (no error)=w602) -> (error out=w601:errorcluster)  [unwired: 1 in, 2 out]
        n281 = call <vilib>:"Add State(s) to Queue__JKI_lib_State_Machine.vi"("State(s) in (\"\")"=w611) -> ("States Out"=w610:string)  [unwired: 14 in]
      }
      frame "Data: parseRunDataiRF" {
        w615 = T8 {"CtrlV"=0.0, "WFs"=[], "WFavg"=[]}  # DataAllCluster
        # "add remove dc and normalize"
        # "update graph"
        # "data individual gian"
        # "Flash data from queue and save it in structure\n()"
        n282 = Flush Queue(queue=w629, error in (no error)=w627) -> (remaining elements=w628:cluster{"WF":dbl[][]}[], error out=w618:errorcluster)  [unwired: 1 out]
        n283 = for {
          tunnel: w628 -> [w639] mode=indexing
          tunnel: [w638] -> w622 mode=concatenating
          n284 = Unbundle By Name(w639) -> ("WF"=w638:dbl[][])
        }
        n285 = Array Size(array=w622) -> (size(s)=→"data Size":i32[])
        n286 = Transpose 2D Array(2D array=w622) -> (transposed array=w625:dbl[][])
        n287 = for {
          tunnel: w625 -> [w637] mode=indexing
          tunnel: [w636] -> w616 mode=indexing
          n288 = call-poly <vilib>:"Mean.vi"("X"=w637) -> ("mean"=w636:dbl)  [unwired: 1 out]
        }
        n289 = local read "Ctrl V"() -> (w621:dbl)
        n290 = local read "Channel"() -> (w614:enum32{"Ch1", "Ch2", "Ch3"})
        n291 = Bundle By Name(cluster=w615, "CtrlV"=w621, "WFs"=w622, "WFavg"=w616) -> (w619:T8)
        n292 = Build Array(w616) -> (w624:dbl[][])
        n293 = Enqueue Element(queue=w620, element=w619, error in (no error)=w618) -> (error out=w617:errorcluster)  [unwired: 1 in, 2 out]
        n294 = case shown="\"Ch3\"" w614 {
          tunnel: w624 -> [w633 w634 w635]
          frame "Ch1", Default {
            n295 = local write "Ch1 iRF Graph"(w633) -> ()
          }
          frame "Ch2" {
            n296 = local write "Ch2 iRF Graph"(w634) -> ()
          }
          frame "Ch3" {
            n297 = local write "Ch3 iRF Graph"(w635) -> ()
          }
        }
        n298 = call <vilib>:"Add State(s) to Queue__JKI_lib_State_Machine.vi"("State(s) in (\"\")"=w632) -> ("States Out"=w631:string)  [unwired: 14 in]
      }
      frame "Data: parseRunDataMacro" {
        # "Sometimes it takes some time to parse run data"
        # "Parse data macro.\n(Set curse busy, parse data, then set cursor idle)"
        n299 = local read "Task"() -> (w644:enum32{"iRFAndGain", "Alignment"})
        n300 = case shown="\"Alignment\"" w644 {
          tunnel: ["Data: parseRunDataiRF" ("State(s) in Front (\"\")") "Data: parseRunDataGain" ("State(s) in Front (\"\")")] -> w643
          frame "iRFAndGain", Default {
          }
          frame "Alignment" {
          }
        }
        n301 = call <vilib>:"Add State(s) to Queue__JKI_lib_State_Machine.vi"("State(s) in Front (\"\")"="UI: Cursor Set >> Busy" ("State(s) in Front (\"\")"), "State(s) in (\"\")"=w643, "State(s) at Back (\"\")"="UI: Cursor Set>>Idle" ("State(s) in Front (\"\")")) -> ("States Out"=w642:string)  [unwired: 12 in]
        n302 = call <vilib>:"Add State(s) to Queue__JKI_lib_State_Machine.vi"("State(s) in Front (\"\")"=w642, "State(s) in (\"\")"=w649) -> ("States Out"=w648:string)  [unwired: 13 in]
      }
      frame "Data: parseGainBGAllGain" {
        # "Parse all data for all gain\n(parse data all gain)"
        n303 = Unbundle By Name(w652) -> ("SysRunning?"=w655:bool)
        n304 = case shown="False" w655 {
          tunnel: w658 -> [w672 w684]
          tunnel: w657 -> [w671 _]
          tunnel: [w667 w684] -> w656
          tunnel: ["" ("State(s) in Front (\"\")") "Idle\nData: parseGainBGAllGain" ("State(s) in Front (\"\")")] -> w654
          tunnel: w652 -> [w669 w683]
          tunnel: [w666 w683] -> w653
          frame False {
            # "save gain BG to temp"
            n305 = Flush Queue(queue=w671, error in (no error)=w672) -> (remaining elements=w673:cluster{"CtrlV":dbl, "WFs":dbl[][]}[], error out=w667:errorcluster)  [unwired: 1 out]
            n306 = for {
              tunnel: w673 -> [w681] mode=indexing
              tunnel: [w678] -> w668 mode=indexing
              tunnel: [w679] -> w665 mode=indexing
              tunnel: [w677] -> w664 mode=indexing
              n307 = Unbundle By Name(w681) -> ("CtrlV"=w679:dbl, "WFs"=w680:dbl[][])
              n308 = for {
                tunnel: w680 -> [w682] mode=indexing
                tunnel: [w682] -> w678 mode=concatenating
              }
              n309 = call-poly <vilib>:"Mean.vi"("X"=w678) -> ("mean"=w677:dbl)  [unwired: 1 out]
            }
            n310 = local read "Channel"() -> (w663:enum32{"Ch1", "Ch2", "Ch3"})
            n311 = Bundle(w665, w664) -> (w662:cluster{dbl[], dbl[]})  [unwired: 1 in]
            n312 = case shown="\"Ch3\"" w663 {
              tunnel: w662 -> [w674 w675 w676]
              frame "Ch1", Default {
                n313 = local write "Ch1 Gain"(w674) -> ()
              }
              frame "Ch2" {
                n314 = local write "Ch2 Gain"(w675) -> ()
              }
              frame "Ch3" {
                n315 = local write "Ch3 Gain"(w676) -> ()
              }
            }
            n316 = Bundle By Name(cluster=w669, "GainBGRaw"=w668) -> (w666:T22)
          }
          frame True {
            # "repeat if system is running"
          }
        }
        n317 = call <vilib>:"Add State(s) to Queue__JKI_lib_State_Machine.vi"("State(s) in Front (\"\")"=w654, "State(s) in (\"\")"=w661) -> ("States Out"=w660:string)  [unwired: 13 in]
      }
      frame "Data: parseDataAllGainMacro" {
        # "Do not put any code in this frame.\n(It is a separator no-op. You can make a copy of this frame to create a new Data frame)"
        n318 = local read "Task"() -> (w687:enum32{"iRFAndGain", "Alignment"})
        n319 = case shown="\"Alignment\"" w687 {
          tunnel: ["APD: writeiRF" ("State(s) in Front (\"\")") w695] -> w686
          frame "iRFAndGain", Default {
          }
          frame "Alignment" {
            n320 = case shown="True" "BG flag?" {
              tunnel: ["APD: writeGain" ("State(s) in Front (\"\")") "Data: parseGainBGAllGain" ("State(s) in Front (\"\")")] -> w695
              frame False {
              }
              frame True {
              }
            }
          }
        }
        n321 = call <vilib>:"Add State(s) to Queue__JKI_lib_State_Machine.vi"("State(s) in Front (\"\")"=w686, "State(s) in (\"\")"=w692) -> ("States Out"=w691:string)  [unwired: 13 in]
      }
      frame "Data: parseSingleGainData" {
        # "Parse gain data for a single gain.\n(Flush data from queue, calculate peak V and std)"
        n322 = Flush Queue(queue=w721, error in (no error)=w699) -> (remaining elements=w722:cluster{"WF":dbl[][]}[], error out=w701:errorcluster)  [unwired: 1 out]
        n323 = for {
          tunnel: w722 -> [w736] mode=indexing
          tunnel: [w735] -> w720 mode=concatenating
          tunnel: [w734] -> w706 mode=concatenating
          tunnel: [w733] -> w698 mode=concatenating
          n324 = Unbundle By Name(w736) -> ("WF"=w733:dbl[][])
          n325 = for {
            tunnel: w733 -> [w739] mode=indexing
            tunnel: [w738] -> w735 mode=indexing
            tunnel: [w737] -> w734 mode=indexing
            n326 = disable-structure shown="Enabled" {
              disable-tunnel: w739 -> [w742 w748]
              disable-tunnel: [w747 w760] -> w738
              disable-tunnel: [_ w749] -> w737
              frame Disabled {
                n327 = global read "GlobalVariables.vi" "DC Idx1"() -> (w745:i32)
                n328 = global read "GlobalVariables.vi" "DC Idx2"() -> (w746:i32)
                n329 = Subtract(x=w746, y=w745) -> (x-y=w744:i32)
                n330 = Array Subset(array=w742, index=w745, length=w744) -> (w743:dbl[])
                n331 = call-poly <vilib>:"Mean.vi"("X"=w743) -> ("mean"=w741:dbl)  [unwired: 1 out]
                n332 = Subtract(x=w742, y=w741) -> (x-y=w740:dbl[])
                n333 = Array Max & Min(array=w740) -> (max value=w747:dbl)  [unwired: 3 out]
              }
              frame Enabled {
                # "Compute AUC"
                # "DC remove"
                n334 = global read "GlobalVariables.vi" "DC Idx1"() -> (w755:i32)
                n335 = global read "GlobalVariables.vi" "DC Idx2"() -> (w757:i32)
                n336 = Subtract(x=w757, y=w755) -> (x-y=w756:i32)
                n337 = Array Subset(array=w748, index=w755, length=w756) -> (w754:dbl[])
                n338 = call-poly <vilib>:"Mean.vi"("X"=w754) -> ("mean"=w753:dbl)  [unwired: 1 out]
                n339 = Subtract(x=w748, y=w753) -> (x-y=w752:dbl[])
                n340 = global read "GlobalVariables.vi" "BG Idx2"() -> (w759:i32)
                n341 = global read "GlobalVariables.vi" "BG Idx1"() -> (w758:i32)
                n342 = Subtract(x=w759, y=w758) -> (x-y=w751:i32)
                n343 = Array Subset(array=w752, index=w758, length=w751) -> (w750:dbl[])
                n344 = Array Max & Min(array=w748) -> (max value=w749:dbl)  [unwired: 3 out]
                n345 = Add Array Elements(numeric array=w750) -> (sum=w760:dbl)
              }
            }
          }
        }
        n346 = call "V1FGV.vi"("action (write)"=enum16{"write", "read"}."read") -> ("V1 out"=w703:dbl)  [unwired: 9 in, 1 out]
        n347 = Unbundle By Name(w719) -> ("GainDataTemp.IntFactor"=w709:dbl, "GainDataTemp.CtrlV"=w714:dbl, "GainDataTemp.AUC"=w711:dbl)
        n348 = Equal?(x=w703, y=w714) -> (x = y?=w713:bool)
        n349 = call <vilib>:"Std Deviation and Variance.vi"("X"=w720) -> ("mean"=w712:dbl, "standard deviation"=w716:dbl)  [unwired: 1 in, 1 out]
        n350 = call-poly <vilib>:"Mean.vi"("X"=w706) -> ("mean"=w705:dbl)  [unwired: 1 out]
        n351 = case shown="True" w713 {
          tunnel: w712 -> [_ w732]
          tunnel: w711 -> [_ w731]
          tunnel: [w727 w728] -> w710
          tunnel: w709 -> [w727 w730]
          frame False {
            # "if new Ctrl V, use old int factor"
          }
          frame True {
            # "if current CtrlV is the same as last, this is intensity change point, calculate intensity factor"
            n352 = Divide(x=w732, y=w731) -> (x/y=w729:dbl)
            n353 = Multiply(x=w730, y=w729) -> (x*y=w728:dbl)
          }
        }
        n354 = Greater?(x=w705, y=1.2) -> (0:w707:bool)
        n355 = Divide(x=w712, y=w710) -> (x/y=w715:dbl)
        n356 = Bundle By Name(cluster=w719, "GainDataTemp.CtrlV"=w703, "GainDataTemp.AUC"=w712, "GainDataTemp.AUC Std"=w716, "GainDataTemp.IntFactor"=w710, "GainDataTemp.IntCorrAUC"=w715) -> (w718:T22)
        n357 = case shown="True" w707 {
          frame False {
          }
          frame True {
            # "Inform user data near maximum"
            n358 = One Button Dialog(message="Data near threshold! Move target away and retake data at the same gain to record intensity change! ") -> ()  [unwired: 1 in, 1 out]
          }
        }
        n359 = Bundle("V1 out"=w703, "WF"=w698) -> (w702:cluster{"V1 out":dbl, "WF":dbl[][]})  [unwired: 1 in]
        n360 = Enqueue Element(queue=w704, element=w702, error in (no error)=w701) -> (error out=w700:errorcluster)  [unwired: 1 in, 2 out]
        n361 = call <vilib>:"Add State(s) to Queue__JKI_lib_State_Machine.vi"("State(s) in (\"\")"=w725) -> ("States Out"=w724:string)  [unwired: 14 in]
      }
      frame "Data: parseIRFSingleIRFData" {
        w770 = T8 {"CtrlV"=0.0, "WFs"=[], "WFavg"=[]}  # iRFDataAllCluster
        # "Parse iRF data from a single gain\n(It is a separator no-op. You can make a copy of this frame to create a new Data frame)"
        n362 = Flush Queue(queue=w777, error in (no error)=w767) -> (remaining elements=w776:cluster{"WF":dbl[][]}[], error out=w769:errorcluster)  [unwired: 1 out]
        n363 = for {
          tunnel: w776 -> [w784] mode=indexing
          tunnel: [w783] -> w772 mode=concatenating
          n364 = Unbundle By Name(w784) -> ("WF"=w783:dbl[][])
        }
        n365 = Transpose 2D Array(2D array=w772) -> (transposed array=w774:dbl[][])
        n366 = for {
          tunnel: w774 -> [w782] mode=indexing
          tunnel: [w781] -> w766 mode=indexing
          # "Average WF"
          n367 = call-poly <vilib>:"Mean.vi"("X"=w782) -> ("mean"=w781:dbl)  [unwired: 1 out]
        }
        "Current iRF" <- w766
        n368 = call "V1FGV.vi"("action (write)"=enum16{"write", "read"}."read") -> ("V1 out"=w773:dbl)  [unwired: 9 in, 1 out]
        n369 = Bundle By Name(cluster=w770, "CtrlV"=w773, "WFs"=w772, "WFavg"=w766) -> (w761:T8)
        n370 = Enqueue Element(queue=w771, element=w761, error in (no error)=w769) -> (error out=w768:errorcluster)  [unwired: 1 in, 2 out]
        n371 = Unbundle By Name(w762) -> ("iRFIdx"=w765:i32)
        n372 = Increment(x=w765) -> (x+1=w764:i32)
        n373 = Bundle By Name(cluster=w762, "iRFIdx"=w764) -> (w763:T22)
        n374 = call <vilib>:"Add State(s) to Queue__JKI_lib_State_Machine.vi"("State(s) in (\"\")"=w780) -> ("States Out"=w779:string)  [unwired: 14 in]
      }
      frame "Data: saveiRF" {
        w809 = enum16{"write", "read"}."read" ("action")
        # "Get iRF from decon stracture and save it on disk.\n(It is a separator no-op. You can make a copy of this frame to create a new Data frame)"
        n375 = Unbundle By Name(w785) -> ("TempPath"=w786:path)
        n376 = call "Ch1DeconEngineFGV.vi"("action(read)"=w809) -> ("Error Out"=w807:errorcluster, "Ch1DeconEngine out"=w808:refnum<class "LaguerreDeconEngineClass.lvclass">)  [unwired: 9 in]
        n377 = call "Ch2DeconEngineFGV.vi"("action(read)"=w809) -> ("Error Out"=w805:errorcluster, "Ch2DeconEngine out"=w806:refnum<class "LaguerreDeconEngineClass.lvclass">)  [unwired: 9 in]
        n378 = call "Ch3DeconEngineFGV.vi"("action(read)"=w809) -> ("Error Out"=w803:errorcluster, "Ch3DeconEngine out"=w804:refnum<class "LaguerreDeconEngineClass.lvclass">)  [unwired: 9 in]
        n379 = Build Path(base path=w786, name or relative path="iRF" ("default name")) -> (appended path=w801:path)
        n380 = call "getIRF.vi"("error in (no error)"=w807, "LaguerreDeconEngineClass in"=w808) -> ("iRF"=w790:dbl[])  [unwired: 7 in, 2 out]
        n381 = call "getIRF.vi"("error in (no error)"=w805, "LaguerreDeconEngineClass in"=w806) -> ("iRF"=w789:dbl[])  [unwired: 7 in, 2 out]
        n382 = call "getIRF.vi"("error in (no error)"=w803, "LaguerreDeconEngineClass in"=w804) -> ("iRF"=w788:dbl[])  [unwired: 7 in, 2 out]
        n383 = Build Array(w790, w789, w788) -> (w796:dbl[][])
        n384 = TDMS Open(8:w800, 10:T14."create or replace" ("operation (0:open)"), 11:w801) -> (0:w797:errorcluster, 3:w798:refnum<k34>)  [unwired: 4 in]
        n385 = Bundle("iRF"=w790, "iRF"=w789, "iRF"=w788) -> (w787:cluster{"iRF":dbl[], "iRF":dbl[], "iRF":dbl[]})  [unwired: 1 in]
        n386 = global write "GlobalVariables.vi" "LastUseiRF"(w787) -> ()
        n387 = TDMS Write(0:w798, 5:"iRF" ("group name in (Untitled)"), 7:string[] ["Ch1", "Ch2", "Ch3"] ("channel name(s) in (Untitled)"), 9:w796, 11:w797) -> (4:w793:refnum<k34>, 15:w792:errorcluster)  [unwired: 1 in, 2 out]
        n388 = TDMS Close(8:w792, 11:w793) -> (0:w791:errorcluster)  [unwired: 1 out]
        n389 = call <vilib>:"Add State(s) to Queue__JKI_lib_State_Machine.vi"("State(s) in (\"\")"=w812) -> ("States Out"=w811:string)  [unwired: 14 in]
      }
      frame "Data: Cleanup" {
        # "Cleanup any data and references, here.\n(this is called automatically, by the Macro: Exit)"
        n390 = Unbundle By Name(w813) -> ("Core.Current VI Reference"=w814:refnum<vi>)
        n391 = Close Reference(reference=w814, error in (no error)=w817) -> (error out=w816:errorcluster)
        n392 = call <vilib>:"Add State(s) to Queue__JKI_lib_State_Machine.vi"("State(s) in (\"\")"=w819) -> ("States Out"=w818:string)  [unwired: 14 in]
      }
      frame "---------- Core ----------" {
        # "Do not put any code in this frame.\n(it is a separator no-op)"
        n393 = call <vilib>:"Add State(s) to Queue__JKI_lib_State_Machine.vi"("State(s) in (\"\")"=w824) -> ("States Out"=w823:string)  [unwired: 14 in]
      }
      frame Default {
        w835 = 42 items=["No error", "Argument error", "Memory is full", "Out of zone", "End of file", "File already open", "Generic file I/O error", "File not found", "File permission error", "Disk is full", "Duplicate path", "Too many files open", "System feature not enabled", "Resource file not found", "Cannot add resource", "Resource not found", "Image not found", "Image memory error", "Pen does not exist", "Config type invalid", "Config token not found", "Config parse error", "Config memory error", "Bad external code format", "Bad external code offset", "External code not present", "Null window", "Destroy window error", "Null menu", "Print aborted", "Bad print record", "Print driver error", "Windows error during printing", "Memory error during printing", "Print dialog error", "Generic print error", "Invalid device refnum", "Device not found", "Device parameter error", "Device unit error", "Cannot open device", "Device call aborted", "Generic error", "Cancelled by user", "Object ID too low", "Object ID too high", "Object not in heap", "Unknown heap", "Unknown object (invalid DefProc)", "Unknown object (DefProc not in table)", "Message out of range", "Invalid (null) method", "Unknown message", "Manager call not supported", "Bad address", "Network operation in progress", "Network operation timed out", "Connection is busy", "Network attribute not supported", "Network error", "Address in use", "System out of memory", "Connection aborted", "Connection refused", "Not connected", "Already connected", "Connection closed", "Initialization error (interapplication manager)", "Bad occurrence", "Wait on unbound occurrence handler", "Occurrence queue overflow", "Datalog type conflict", "Unused", "Unrecognized type (interapplication manager)", "Memory corrupt", "Failed to make temporary DLL", "Old CIN version", "Drag socket not found", "Failed to load drop-object", "Failed to register OLE object", "Failed to release OLE object", "Format specifier type mismatch", "Unknown format specifier", "Too few format specifiers", "Too many format specifiers", "Scan failed", "Newer CIN version", "Error converting to variant", "Runtime menu error", "Password tampered", "Variant attribute not found", "Incompatible variant data type", "Event data is not available", "Event Store is not present", "Occurrence is not found", "Event Queue is not created", "Event info is not available", "Refnum passed is NULL", "Error retrieving Class GUID", "Error retrieving CoClass GUID", "Error retrieving TypeLib GUID.", "Bad built application magic bytes.", "Specific driver is different from the specific driver associated with the Logical Name.", "There is no session opened to the class driver.", "Max Error", "MAX - Error with config objects", "MAX - Error loading configuration", "MAX - Group not supported"]
        # "Current State"
        # "Do not delete, rename, or modify this frame.\n(this is used to capture unhandled states and typos)"
        # "Handle mistyped state name (developer tool)"
        n394 = Format Into String(format string="Software Exception: Unhandled State \"%s\"." ("message"), error in=w831, w826) -> (resulting string=w834:string, error out=w833:errorcluster)  [unwired: 1 in]
        n395 = call <vilib>:"Error Cluster From Error Code.vi"("show call chain? (False)"=TRUE, "error in (no error)"=w833, "error message (\"\")"=w834, "error code (0)"=w835) -> ("error out"=w832:errorcluster)  [unwired: 5 in]
        n396 = call <vilib>:"Add State(s) to Queue__JKI_lib_State_Machine.vi"("State(s) in (\"\")"=w830) -> ("States Out"=w829:string)  [unwired: 14 in]
      }
      frame "Initialize Core Data" {
        # "Build default path based on the location of project"
        # "Do not delete, rename, or modify this frame.\n(this is used to determine panel behavior on exit)"
        # "originally closed?"
        # "exe?"
        # "If panel starts closed or is an EXE, then close it when we exit"
        n397 = call <vilib>:"Application Directory.vi"() -> ("Application Directory"=w839:path)
        n398 = property on="Property Node" class="App"() -> ("App.Kind"=w852:T16)  [unwired: 2 in, 2 out]
        n399 = property on="Property Node" class="VI"() -> ("FP.State"=w847:T15)  [unwired: 2 in, 2 out]
        n400 = control-ref of="Current VI Reference"() -> (w848:refnum<vi>)
        n401 = Equal?(x=w847, y=T15."Closed" ("Front Panel Window:State")) -> (x = y?=w845:bool)
        n402 = Equal?(x=w852, y=T16."Run Time System" ("Application:Kind")) -> (x = y?=w850:bool)
        n403 = Build Path(base path=w839, name or relative path="Data") -> (appended path=w843:path)
        n404 = Build Path(base path=w839, name or relative path="SystemTemp") -> (appended path=w840:path)
        n405 = Or(x=w845, y=w850) -> (x .or. y?=w849:bool)
        n406 = Bundle By Name(cluster=w838, "Core.Current VI Reference"=w848, "Core.Close Panel on Exit?"=w849, "DefaultPath"=w843, "TempPath"=w840) -> (w837:T22)
        n407 = call <vilib>:"Add State(s) to Queue__JKI_lib_State_Machine.vi"("State(s) in (\"\")"=w855) -> ("States Out"=w854:string)  [unwired: 14 in]
      }
      frame "Error Handler" {
        # "Unhandled Error -- Display it"
        # "Handle any errors here.\nYou can also output any states to clean-up after errors occur"
        # "Clear error"
        n408 = Unbundle By Name(w856) -> ("code"=w858:i32)
        n409 = case shown="5005" w858 {
          tunnel: ["Macro: Exit" w868 w874 ""] -> w857
          tunnel: w856 -> [w864 _ _ _]
          frame Default {
            w866 = T30 1 items=["no dialog", "OK message", "continue or stop message", "OK message + warnings", "continue/stop + warnings"] ("type of dialog (OK msg:1)")
            n410 = call <vilib>:"General Error Handler.vi"("type of dialog (OK msg:1)"=w866, "error in (no error)"=w864) -> ()  [unwired: 9 in, 5 out]
          }
          frame 5002 {
            n411 = Two Button Dialog(message="Laser interlock open! Please close interlock and try again! ", 1:"Safely Shutdown" ("F button name (\"Cancel\")"), 2:"OK" ("T button name (\"OK\")")) -> (T button?=w869:bool)
            n412 = case shown="True" w869 {
              tunnel: ["Macro: Exit" "355 Laser: CheckControllerStatus"] -> w868
              frame False {
              }
              frame True {
              }
            }
          }
          frame 5001 {
            n413 = Two Button Dialog(message="Unable to connect to imaging computer, do you want to run data aquisiton along? ", 1:"No" ("F button name (\"Cancel\")"), 2:"Yes" ("T button name (\"OK\")")) -> (T button?=w875:bool)
            n414 = case shown="True" w875 {
              tunnel: ["Macro: Exit" "" ("Empty String Constant")] -> w874
              frame False {
              }
              frame True {
              }
            }
          }
          frame 5005 {
          }
        }
        n415 = call <vilib>:"Add State(s) to Queue__JKI_lib_State_Machine.vi"("State(s) in Front (\"\")"=w857, "State(s) in (\"\")"=w863) -> ("States Out"=w862:string)  [unwired: 13 in]
      }
      frame "Exit" {
        # "Do not put any code in this frame.\n(No errors that occur here will be handled.)"
        n416 = call <vilib>:"Add State(s) to Queue__JKI_lib_State_Machine.vi"("State(s) in (\"\")"=w887) -> ("States Out"=w886:string)  [unwired: 14 in]
      }
      frame "---------- AimingBeam ----------" {
        # "Template Separator\n(You can make a copy of, or modify, this frame)"
        n417 = call <vilib>:"Add State(s) to Queue__JKI_lib_State_Machine.vi"("State(s) in (\"\")"=w892) -> ("States Out"=w891:string)  [unwired: 14 in]
      }
      frame "AimingBeam: Initialize" {
        # "set aiming beam button color"
        # "Open COM port for Aiming Beam\n(Require USB connection)"
        n418 = Unbundle By Name(w894) -> ("AB Cluster.Aiming Beam COM Port"=w893:refnum<visa-resource-name>)
        n419 = call-poly "VISA Configure Serial Port"("VISA resource name"=w893, "Enable Termination\nChar (T)"=TRUE ("Enable Termination\nChar (T)"), "baud rate (9600)"=u32 9600, "error in (no error)"=w900) -> ("error out"=w899:errorcluster)  [unwired: 10 in, 1 out]
        n420 = Unbundle By Name(w899) -> ("status"=w898:bool)
        n421 = Not(x=w898) -> (.not. x?=w897:bool)
        n422 = Bundle By Name(cluster=w894, "System Status.Aiming Beam"=w897) -> (w895:T22)
        n423 = call <vilib>:"Add State(s) to Queue__JKI_lib_State_Machine.vi"("State(s) in (\"\")"=w904) -> ("States Out"=w903:string)  [unwired: 14 in]
      }
      frame "AimingBeam: Close" {
        # "Close Aiming Beam COM port\n(Require USB connection to Aiming Beam Laser)"
        n424 = Unbundle By Name(w906) -> ("AB Cluster.Aiming Beam COM Port"=w907:refnum<visa-resource-name>)
        n425 = VISA Close(VISA resource name=w907, error in (no error)=w910) -> (error out=w911:errorcluster)
        n426 = Bundle By Name(cluster=w906, "System Status.Aiming Beam"=FALSE) -> (w905:T22)
        n427 = call <vilib>:"Add State(s) to Queue__JKI_lib_State_Machine.vi"("State(s) in (\"\")"=w913) -> ("States Out"=w912:string)  [unwired: 14 in]
      }
      frame "AimingBeam: Set Current" {
        # "Set Aiming Beam Current\n(You can make a copy of, or modify, this frame)"
        n428 = Unbundle By Name(w915) -> ("AB Cluster.Aiming Beam COM Port"=w914:refnum<visa-resource-name>, "AB Cluster.Max Current"=w919:dbl, "AB Cluster.Default Current"=w918:dbl, "AB Cluster.Min Current"=w917:dbl)
        n429 = In Range and Coerce(upper limit=w919, x=w918, lower limit=w917) -> (coerced(x)=w916:dbl)  [unwired: 1 out]
        n430 = local write "Current"(w916) -> ()
        n431 = Number To Fractional String(number=w916, precision (6)=i16 2) -> (F-format string=w923:string)  [unwired: 2 in]
        n432 = Concatenate Strings("slc:", w923, "\r" ("Carriage Return Constant"), "\n" ("Line Feed Constant")) -> (w926:string)
        n433 = VISA Write(VISA resource name=w914, write buffer=w926, error in (no error)=w921) -> (error out=w922:errorcluster)  [unwired: 2 out]
        n434 = call <vilib>:"Add State(s) to Queue__JKI_lib_State_Machine.vi"("State(s) in (\"\")"=w930) -> ("States Out"=w929:string)  [unwired: 14 in]
      }
      frame "AimingBeam: Set Status" {
        # "Enable Aiming Beam\n(Usage: \"AimingBeam: Set >> Enable|Disable\")"
        n435 = Unbundle By Name(w931) -> ("AB Cluster.Aiming Beam COM Port"=w932:refnum<visa-resource-name>)
        n436 = case shown="\"Enable\"" w937 {
          tunnel: [w939 w943] -> w936
          frame "Disable", Default {
            n437 = Concatenate Strings("cof", "\r" ("Carriage Return Constant"), "\n" ("Line Feed Constant")) -> (w939:string)
          }
          frame "Enable" {
            n438 = Concatenate Strings("con", "\r" ("Carriage Return Constant"), "\n" ("Line Feed Constant")) -> (w943:string)
          }
        }
        n439 = VISA Write(VISA resource name=w932, write buffer=w936, error in (no error)=w934) -> (error out=w935:errorcluster)  [unwired: 2 out]
      }
      frame "AimingBeam: GetPWMStatus" {
        # "Get aiming beam PWM status\n()"
        n440 = local read "AB Rep Rate"() -> (w948:u16)
        n441 = Greater Than 0?(x=w948) -> (x > 0?=w947:bool)
        n442 = case shown="True" w947 {
          tunnel: w951 -> [w955 w960]
          tunnel: w950 -> [_ w959]
          tunnel: [w955 w958] -> w949
          frame False {
          }
          frame True {
            n443 = Unbundle By Name(w959) -> ("LJ Pinout.AimingBeam PWM"=w956:string)
            n444 = call "LabJack_FGV.vi"("Operation(Read)"=enum16{"Write", "Read"}."Read" ("Operation"), "error in (no error)"=w960) -> ("error out"=w963:errorcluster, "Read data"=w964:i32)  [unwired: 8 in]
            n445 = Concatenate Strings(w956, "_EF_ENABLE" ("string")) -> (w962:string)
            n446 = call "LJM_eReadName.vi"("Handle In"=w964, "Name"=w962, "error in"=w963) -> ("Value"=w961:dbl, "error out"=w958:errorcluster)  [unwired: 10 in, 1 out]
            n447 = Greater Than 0?(x=w961) -> (x > 0?=w957:bool)
            n448 = case shown="True" w957 {
              frame False {
                # "PWM is off\nset color to gray"
                n449 = local write "Aiming beam toggle"(FALSE ("Aimging beam")) -> ()
              }
              frame True {
                # "PWM is on\nset color to light green"
                n450 = local write "Aiming beam toggle"(TRUE ("Aimging beam")) -> ()
              }
            }
          }
        }
        n451 = call <vilib>:"Add State(s) to Queue__JKI_lib_State_Machine.vi"("State(s) in (\"\")"=w954) -> ("States Out"=w953:string)  [unwired: 14 in]
      }
      frame "AimingBeam: ComputePWM" {
        # "Compute PWM parameter based on AB frequency\n(You can make a copy of, or modify, this frame)"
        n452 = Unbundle By Name(w970) -> ("AB Cluster.Frequency(Hz)"=w969:i32)
        n453 = call "LJ_calculate_PWM_parameters.vi"("Duty Cycle (%)"="Duty Cycle (%)", "Error In"=w971, "Show Confirmation"=FALSE, "Laser Rep Rate (Hz)"=w969, "Laser"=enum16{"355nm", "AimingBeam"}."AimingBeam") -> ("Error Out"=w972:errorcluster)  [unwired: 5 in, 1 out]
        n454 = call <vilib>:"Add State(s) to Queue__JKI_lib_State_Machine.vi"("State(s) in (\"\")"=w978) -> ("States Out"=w977:string)  [unwired: 14 in]
      }
      frame "---------- Digitizer ----------" {
        # "Template Separator\n(You can make a copy of, or modify, this frame)"
        n455 = call <vilib>:"Add State(s) to Queue__JKI_lib_State_Machine.vi"("State(s) in (\"\")"=w983) -> ("States Out"=w982:string)  [unwired: 14 in]
      }
      frame "Digitizer: ConfigMacro" {
        # "Digitizer Configuration Macro\n(Decide how to config digitizer)"
        n456 = case shown="\"Alignment\"" "Task" {
          tunnel: "Channel" -> [w995 w1000]
          tunnel: [w994 w999] -> w986
          frame "iRFAndGain", Default {
            n457 = case shown="\"Ch3\"" w995 {
              tunnel: ["Digitizer: ConfigCh1iRF" ("State(s) at Back (\"\")") "Digitizer: ConfigCh2iRF" ("State(s) at Back (\"\")") "Digitizer: ConfigCh3iRF" ("State(s) at Back (\"\")")] -> w994
              frame "Ch1", Default {
              }
              frame "Ch2" {
              }
              frame "Ch3" {
              }
            }
          }
          frame "Alignment" {
            n458 = case shown="\"Ch3\"" w1000 {
              tunnel: ["Digitizer: ConfigCh1Align" ("State(s) at Back (\"\")") "Digitizer: ConfigCh2Align" ("State(s) at Back (\"\")") "Digitizer: ConfigCh3Align" ("State(s) at Back (\"\")")] -> w999
              frame "Ch1", Default {
              }
              frame "Ch2" {
              }
              frame "Ch3" {
              }
            }
          }
        }
        n459 = call <vilib>:"Add State(s) to Queue__JKI_lib_State_Machine.vi"("State(s) in Front (\"\")"=w986, "State(s) in (\"\")"="Graph: SetXScale\nGraph: ClearHistory\nMacro: SysReadyForAqui" ("State(s) in (\"\")")) -> ("States Out"=w984:string)  [unwired: 13 in]
        n460 = call <vilib>:"Add State(s) to Queue__JKI_lib_State_Machine.vi"("State(s) in Front (\"\")"=w984, "State(s) in (\"\")"=w993) -> ("States Out"=w992:string)  [unwired: 13 in]
      }
      frame "Digitizer: Initialize" {
        # "Initialize digitizer.\nInitialize both digitizer and update status."
        n461 = call "FLImDAQ_FGV.vi"("error in (no error)"=w1010) -> ("error out"=w1004:errorcluster, "Read data"=w1009:T4)  [unwired: 9 in]
        n462 = property on="Digitizer" class="Bool (strict)"("Blinking"=TRUE) -> ()  [unwired: 2 in, 2 out]
        n463 = Unbundle By Name(w1009) -> ("Digitizer 1"=w1008:refnum<k15>, "Digitizer 2"=w1007:refnum<k15>)
        n464 = case shown="No Error" w1004 {
          selector: w1004 -> [w1017 w1021]
          tunnel: [w1020 w1021] -> w1012
          tunnel: w1007 -> [w1019 _]
          frame No Error {
            n465 = call <instrlib>:"niScope Initialize.vi"("resource name"=w1019, "reset device"=FALSE, "error in"=w1017) -> ("error out"=w1020:errorcluster)  [unwired: 11 in, 1 out]
          }
          frame Error {
          }
        }
        n466 = case shown="No Error" w1004 {
          selector: w1004 -> [w1023 w1026]
          tunnel: w1008 -> [w1025 _]
          tunnel: [w1022 w1026] -> w1005
          frame No Error {
            n467 = call <instrlib>:"niScope Initialize.vi"("resource name"=w1025, "reset device"=FALSE, "error in"=w1023) -> ("error out"=w1022:errorcluster)  [unwired: 11 in, 1 out]
          }
          frame Error {
          }
        }
        n468 = Merge Errors(w1005, w1012) -> (w1011:errorcluster)
        n469 = call <vilib>:"Add State(s) to Queue__JKI_lib_State_Machine.vi"("State(s) in (\"\")"=w1016) -> ("States Out"=w1015:string)  [unwired: 14 in]
      }
      frame "Digitizer: ConfigCh3iRF" {
        # "Hardcode channel to 0, which is Ch1 and Ch3."
        # "Synchronize is taking time ~3s."
        # "Config  digitizer\nCall subVi to config digitizer"
        n470 = Unbundle By Name(w1030) -> ("FLImDAQ"=w1031:T27)
        n471 = call "FLImDAQ_FGV.vi"() -> ("Read data"=w1055:T4)  [unwired: 10 in, 1 out]
        n472 = Bundle By Name(cluster=w1031, "Channel"=enum16{"Channel 0", "Channel 1", "Channel 0&1"}."Channel 0") -> (w1032:T27)
        n473 = Unbundle By Name(w1055) -> ("Digitizer 1"=w1058:refnum<k15>, "Digitizer 2"=w1057:refnum<k15>)
        n474 = property on="Digitizer" class="Bool (strict)"(error in=w1059, "Blinking"=TRUE) -> (error out=w1035:errorcluster)  [unwired: 1 in, 1 out]
        n475 = case shown="No Error" w1035 {
          selector: w1035 -> [w1075 w1078]
          tunnel: w1032 -> [w1074 _]
          tunnel: [w1077 w1078] -> w1034
          tunnel: w1058 -> [w1076 _]
          frame No Error {
            n476 = call "DigitizerConfig.vi"("error in (no error)"=w1075, "FLImDAQ"=w1074, "IVI Refnum in"=w1076) -> ("error out"=w1077:errorcluster)  [unwired: 7 in, 1 out]
          }
          frame Error {
          }
        }
        n477 = case shown="No Error" w1034 {
          selector: w1034 -> [w1068 w1073]
          tunnel: w1032 -> [w1067 _]
          tunnel: [w1071 w1073] -> w1041
          tunnel: w1057 -> [w1069 w1072]
          tunnel: [w1066 w1072] -> w1028
          frame No Error {
            n478 = call "DigitizerConfig.vi"("Config Trigger? (T)"=FALSE ("Config Trigge(T)r:"), "error in (no error)"=w1068, "FLImDAQ"=w1067, "IVI Refnum in"=w1069) -> ("error out"=w1071:errorcluster, "IVI Refnum out"=w1066:refnum<k15>)  [unwired: 6 in]
          }
          frame Error {
          }
        }
        n479 = call "Digitizer1_FGV.vi"("error in (no error)"=w1041, "Operation (Read)"=enum16{"Write", "Read"}."Read" ("Operation")) -> ("error out"=w1052:errorcluster, "Read data"=w1053:refnum<k15>)  [unwired: 8 in]
        n480 = call <instrlib>:"niScope Get Session Reference.vi"("instrument handle"=w1053, "error in"=w1052) -> ("session reference"=w1045:refnum<k20>, "error out"=w1043:errorcluster)  [unwired: 11 in, 1 out]
        n481 = call "Digitizer2_FGV.vi"("error in (no error)"=w1043, "Operation (Read)"=enum16{"Write", "Read"}."Read" ("Operation")) -> ("error out"=w1049:errorcluster, "Read data"=w1050:refnum<k15>)  [unwired: 8 in]
        n482 = call <instrlib>:"niScope Get Session Reference.vi"("instrument handle"=w1050, "error in"=w1049) -> ("session reference"=w1044:refnum<k20>, "error out"=w1042:errorcluster)  [unwired: 11 in, 1 out]
        n483 = Build Array(w1045, w1044) -> (w1048:refnum<k20>[])
        n484 = property class="niScope"(reference=w1028) -> ("Trigger Delay"=→"Triggering:Trigger Delay":dbl)  [unwired: 1 in, 2 out]
        n485 = call <instrlib>:"niTClk Configure For Homogeneous Triggers.vi"("error in (no error)"=w1042, "sessions"=w1048) -> ("error out"=w1047:errorcluster, "sessions out"=w1046:refnum<k20>[])  [unwired: 8 in]
        n486 = call <instrlib>:"niTClk Synchronize.vi"("error in (no error)"=w1047, "sessions"=w1046) -> ("error out"=w1040:errorcluster, "sessions out"=w1037:refnum<k20>[])  [unwired: 8 in]
        n487 = call <userlib>:"Wait (ms)__ogtk.vi"("error in (no error)"=w1040, "milliseconds to wait"=u32 1500) -> ("error out"=w1039:errorcluster)  [unwired: 8 in, 1 out]
        n488 = Unbundle By Name(w1039) -> ("status"=w1062:bool)
        n489 = Not(x=w1062) -> (.not. x?=w1061:bool)
        n490 = Bundle By Name(cluster=w1030, "System Status.Digitizer"=w1061, "niTClk sessions"=w1037) -> (w1029:T22)
        n491 = property on="Digitizer" class="Bool (strict)"(error in=w1039, "Blinking"=FALSE) -> (error out=w1056:errorcluster)  [unwired: 1 in, 1 out]
        n492 = call <vilib>:"Add State(s) to Queue__JKI_lib_State_Machine.vi"("State(s) in (\"\")"=w1065) -> ("States Out"=w1064:string)  [unwired: 14 in]
      }
      frame "Digitizer: ConfigCh1iRF" {
        # "Synchronize is taking time ~3s."
        # "Config  digitizer\nCall subVi to config digitizer"
        n493 = Unbundle By Name(w1080) -> ("FLImDAQ"=w1081:T27)
        n494 = call "FLImDAQ_FGV.vi"() -> ("Read data"=w1087:T4)  [unwired: 10 in, 1 out]
        n495 = property on="Digitizer" class="Bool (strict)"(error in=w1090, "Blinking"=TRUE) -> (error out=w1085:errorcluster)  [unwired: 1 in, 1 out]
        n496 = Unbundle By Name(w1087) -> ("Digitizer 1"=w1089:refnum<k15>)
        n497 = Bundle By Name(cluster=w1081, "Channel"=enum16{"Channel 0", "Channel 1", "Channel 0&1"}."Channel 0") -> (w1083:T27)
        n498 = case shown="No Error" w1085 {
          selector: w1085 -> [w1098 w1101]
          tunnel: w1083 -> [w1097 _]
          tunnel: [w1100 w1101] -> w1084
          tunnel: w1089 -> [w1099 _]
          frame No Error {
            n499 = call "DigitizerConfig.vi"("error in (no error)"=w1098, "FLImDAQ"=w1097, "IVI Refnum in"=w1099) -> ("error out"=w1100:errorcluster)  [unwired: 7 in, 1 out]
          }
          frame Error {
          }
        }
        n500 = Unbundle By Name(w1084) -> ("status"=w1093:bool)
        n501 = property on="Digitizer" class="Bool (strict)"(error in=w1084, "Blinking"=FALSE) -> (error out=w1088:errorcluster)  [unwired: 1 in, 1 out]
        n502 = Not(x=w1093) -> (.not. x?=w1092:bool)
        n503 = Bundle By Name(cluster=w1080, "System Status.Digitizer"=w1092) -> (w1079:T22)
        n504 = call <vilib>:"Add State(s) to Queue__JKI_lib_State_Machine.vi"("State(s) in (\"\")"=w1096) -> ("States Out"=w1095:string)  [unwired: 14 in]
      }
      frame "Digitizer: ConfigCh1Align" {
        # "Synchronize is taking time ~3s."
        # "Config  digitizer\nCall subVi to config digitizer"
        n505 = Unbundle By Name(w1104) -> ("FLImDAQ"=w1105:T27)
        n506 = call "FLImDAQ_FGV.vi"() -> ("Read data"=w1110:T4)  [unwired: 10 in, 1 out]
        n507 = property on="Digitizer" class="Bool (strict)"(error in=w1113, "Blinking"=TRUE) -> (error out=w1108:errorcluster)  [unwired: 1 in, 1 out]
        n508 = Unbundle By Name(w1110) -> ("Digitizer 1"=w1112:refnum<k15>)
        n509 = Bundle By Name(cluster=w1105, "Channel"=enum16{"Channel 0", "Channel 1", "Channel 0&1"}."Channel 0") -> (w1102:T27)
        n510 = case shown="No Error" w1108 {
          selector: w1108 -> [w1121 w1124]
          tunnel: w1102 -> [w1120 _]
          tunnel: [w1123 w1124] -> w1107
          tunnel: w1112 -> [w1122 _]
          frame No Error {
            n511 = call "DigitizerConfigGain.vi"("error in (no error)"=w1121, "FLImDAQ"=w1120, "IVI Refnum in"=w1122) -> ("error out"=w1123:errorcluster)  [unwired: 7 in, 1 out]
          }
          frame Error {
          }
        }
        n512 = Unbundle By Name(w1107) -> ("status"=w1116:bool)
        n513 = property on="Digitizer" class="Bool (strict)"(error in=w1107, "Blinking"=FALSE) -> (error out=w1111:errorcluster)  [unwired: 1 in, 1 out]
        n514 = Not(x=w1116) -> (.not. x?=w1115:bool)
        n515 = Bundle By Name(cluster=w1104, "System Status.Digitizer"=w1115) -> (w1103:T22)
        n516 = call <vilib>:"Add State(s) to Queue__JKI_lib_State_Machine.vi"("State(s) in (\"\")"=w1119) -> ("States Out"=w1118:string)  [unwired: 14 in]
      }
      frame "Digitizer: ConfigCh2iRF" {
        # "Synchronize is taking time ~3s."
        # "Config  digitizer\nCall subVi to config digitizer"
        n517 = Unbundle By Name(w1126) -> ("FLImDAQ"=w1127:T27)
        n518 = call "FLImDAQ_FGV.vi"() -> ("Read data"=w1133:T4)  [unwired: 10 in, 1 out]
        n519 = property on="Digitizer" class="Bool (strict)"(error in=w1136, "Blinking"=TRUE) -> (error out=w1131:errorcluster)  [unwired: 1 in, 1 out]
        n520 = Unbundle By Name(w1133) -> ("Digitizer 1"=w1135:refnum<k15>)
        n521 = Bundle By Name(cluster=w1127, "Channel"=enum16{"Channel 0", "Channel 1", "Channel 0&1"}."Channel 1") -> (w1129:T27)
        n522 = case shown="No Error" w1131 {
          selector: w1131 -> [w1144 w1147]
          tunnel: w1129 -> [w1143 _]
          tunnel: [w1146 w1147] -> w1130
          tunnel: w1135 -> [w1145 _]
          frame No Error {
            n523 = call "DigitizerConfig.vi"("error in (no error)"=w1144, "FLImDAQ"=w1143, "IVI Refnum in"=w1145) -> ("error out"=w1146:errorcluster)  [unwired: 7 in, 1 out]
          }
          frame Error {
          }
        }
        n524 = Unbundle By Name(w1130) -> ("status"=w1139:bool)
        n525 = property on="Digitizer" class="Bool (strict)"(error in=w1130, "Blinking"=FALSE) -> (error out=w1134:errorcluster)  [unwired: 1 in, 1 out]
        n526 = Not(x=w1139) -> (.not. x?=w1138:bool)
        n527 = Bundle By Name(cluster=w1126, "System Status.Digitizer"=w1138) -> (w1125:T22)
        n528 = call <vilib>:"Add State(s) to Queue__JKI_lib_State_Machine.vi"("State(s) in (\"\")"=w1142) -> ("States Out"=w1141:string)  [unwired: 14 in]
      }
      frame "Digitizer: ConfigCh2Align" {
        # "Synchronize is taking time ~3s."
        # "Config  digitizer\nCall subVi to config digitizer"
        n529 = Unbundle By Name(w1149) -> ("FLImDAQ"=w1150:T27)
        n530 = call "FLImDAQ_FGV.vi"() -> ("Read data"=w1156:T4)  [unwired: 10 in, 1 out]
        n531 = property on="Digitizer" class="Bool (strict)"(error in=w1159, "Blinking"=TRUE) -> (error out=w1154:errorcluster)  [unwired: 1 in, 1 out]
        n532 = Unbundle By Name(w1156) -> ("Digitizer 1"=w1158:refnum<k15>)
        n533 = Bundle By Name(cluster=w1150, "Channel"=enum16{"Channel 0", "Channel 1", "Channel 0&1"}."Channel 1") -> (w1152:T27)
        n534 = case shown="No Error" w1154 {
          selector: w1154 -> [w1167 w1170]
          tunnel: w1152 -> [w1166 _]
          tunnel: [w1169 w1170] -> w1153
          tunnel: w1158 -> [w1168 _]
          frame No Error {
            n535 = call "DigitizerConfigGain.vi"("error in (no error)"=w1167, "FLImDAQ"=w1166, "IVI Refnum in"=w1168) -> ("error out"=w1169:errorcluster)  [unwired: 7 in, 1 out]
          }
          frame Error {
          }
        }
        n536 = Unbundle By Name(w1153) -> ("status"=w1162:bool)
        n537 = property on="Digitizer" class="Bool (strict)"(error in=w1153, "Blinking"=FALSE) -> (error out=w1157:errorcluster)  [unwired: 1 in, 1 out]
        n538 = Not(x=w1162) -> (.not. x?=w1161:bool)
        n539 = Bundle By Name(cluster=w1149, "System Status.Digitizer"=w1161) -> (w1148:T22)
        n540 = call <vilib>:"Add State(s) to Queue__JKI_lib_State_Machine.vi"("State(s) in (\"\")"=w1165) -> ("States Out"=w1164:string)  [unwired: 14 in]
      }
      frame "Digitizer: ConfigCh3Align" {
        # "Synchronize is taking time ~3s."
        # "Config  digitizer\nCall subVi to config digitizer"
        n541 = call "FLImDAQ_FGV.vi"() -> ("Read data"=w1182:T4)  [unwired: 10 in, 1 out]
        n542 = Unbundle By Name(w1172) -> ("FLImDAQ"=w1178:T27)
        n543 = Unbundle By Name(w1182) -> ("Digitizer 1"=w1176:refnum<k15>, "Digitizer 2"=w1171:refnum<k15>)
        n544 = Bundle By Name(cluster=w1178, "Channel"=enum16{"Channel 0", "Channel 1", "Channel 0&1"}."Channel 0") -> (w1175:T27)
        n545 = property on="Digitizer" class="Bool (strict)"(error in=w1184, "Blinking"=TRUE) -> (error out=w1174:errorcluster)  [unwired: 1 in, 1 out]
        n546 = Unbundle By Name(w1172) -> ()  [unwired: 1 out]
        n547 = case shown="No Error" w1174 {
          selector: w1174 -> [w1193 w1195]
          tunnel: w1175 -> [w1192 _]
          tunnel: w1176 -> [w1194 _]
          tunnel: [w1191 w1195] -> w1173
          frame No Error {
            n548 = call "DigitizerConfigGain.vi"("error in (no error)"=w1193, "FLImDAQ"=w1192, "IVI Refnum in"=w1194) -> ("error out"=w1191:errorcluster)  [unwired: 7 in, 1 out]
          }
          frame Error {
          }
        }
        n549 = case shown="No Error" w1173 {
          selector: w1173 -> [w1197 w1202]
          tunnel: w1175 -> [w1200 _]
          tunnel: [w1201 w1202] -> w1180
          tunnel: w1171 -> [w1199 _]
          frame No Error {
            n550 = call <instrlib>:"niScope Reset.vi"("instrument handle"=w1199, "error in"=w1197) -> ("instrument handle out"=w1198:refnum<k15>, "error out"=w1196:errorcluster)  [unwired: 12 in]
            n551 = call "DigitizerConfigGain.vi"("error in (no error)"=w1196, "FLImDAQ"=w1200, "IVI Refnum in"=w1198) -> ("error out"=w1201:errorcluster)  [unwired: 7 in, 1 out]
          }
          frame Error {
          }
        }
        n552 = Unbundle By Name(w1180) -> ("status"=w1187:bool)
        n553 = property on="Digitizer" class="Bool (strict)"(error in=w1180, "Blinking"=FALSE) -> (error out=w1183:errorcluster)  [unwired: 1 in, 1 out]
        n554 = Not(x=w1187) -> (.not. x?=w1186:bool)
        n555 = Bundle By Name(cluster=w1172, "System Status.Digitizer"=w1186) -> (w1177:T22)
        n556 = call <vilib>:"Add State(s) to Queue__JKI_lib_State_Machine.vi"("State(s) in (\"\")"=w1190) -> ("States Out"=w1189:string)  [unwired: 14 in]
      }
      frame "Digitizer: Start" {
        # "send trigger to start acquisition loop"
        # "initilize aquisition"
        # "Template Separator\n(You can make a copy of, or modify, this frame)"
        n557 = local read "Channel"() -> (w1203:enum32{"Ch1", "Ch2", "Ch3"})
        n558 = case shown="\"Ch3\"" w1203 {
          tunnel: w1210 -> [_ w1220]
          tunnel: [w1214 w1222] -> w1206
          tunnel: w1204 -> [w1217 w1221]
          frame "Ch1", "Ch2", Default {
            n559 = call "Digitizer1_FGV.vi"("error in (no error)"=w1217, "Operation (Read)"=enum16{"Write", "Read"}."Read" ("Operation")) -> ("error out"=w1216:errorcluster, "Read data"=w1215:refnum<k15>)  [unwired: 8 in]
            n560 = call <instrlib>:"niScope Initiate Acquisition.vi"("instrument handle"=w1215, "error in"=w1216) -> ("error out"=w1214:errorcluster)  [unwired: 12 in, 1 out]
          }
          frame "Ch3" {
            n561 = local read "Task"() -> (w1219:enum32{"iRFAndGain", "Alignment"})
            n562 = case shown="\"Alignment\"" w1219 {
              tunnel: [w1226 w1227] -> w1222
              tunnel: w1221 -> [w1225 w1231]
              tunnel: w1220 -> [w1223 _]
              frame "iRFAndGain", Default {
                n563 = Unbundle By Name(w1223) -> ("niTClk sessions"=w1224:refnum<k20>[])
                n564 = call <instrlib>:"niTClk Initiate.vi"("error in (no error)"=w1225, "sessions"=w1224) -> ("error out"=w1226:errorcluster)  [unwired: 8 in, 1 out]
              }
              frame "Alignment" {
                n565 = call "Digitizer1_FGV.vi"("error in (no error)"=w1231) -> ("error out"=w1232:errorcluster, "Read data"=w1233:refnum<k15>)  [unwired: 9 in]
                n566 = call <instrlib>:"niScope Initiate Acquisition.vi"("instrument handle"=w1233, "error in"=w1232) -> ("error out"=w1230:errorcluster)  [unwired: 12 in, 1 out]
                n567 = call "Digitizer2_FGV.vi"("error in (no error)"=w1230) -> ("error out"=w1229:errorcluster, "Read data"=w1228:refnum<k15>)  [unwired: 9 in]
                n568 = call <instrlib>:"niScope Initiate Acquisition.vi"("instrument handle"=w1228, "error in"=w1229) -> ("error out"=w1227:errorcluster)  [unwired: 12 in, 1 out]
              }
            }
          }
        }
        n569 = Generate User Event(priority (normal)=usereventprio."high priority", user event=w1207, event data cluster=TRUE ("event data"), error in=w1206) -> (error out=w1205:errorcluster)  [unwired: 1 out]
        n570 = call <vilib>:"Add State(s) to Queue__JKI_lib_State_Machine.vi"("State(s) in (\"\")"=w1213) -> ("States Out"=w1212:string)  [unwired: 14 in]
      }
      frame "Digitizer: Abort" {
        # "Template Separator\n(You can make a copy of, or modify, this frame)"
        n571 = call "Digitizer1_FGV.vi"("error in (no error)"=w1235, "Operation (Read)"=enum16{"Write", "Read"}."Read" ("Operation")) -> ("error out"=w1242:errorcluster, "Read data"=w1239:refnum<k15>)  [unwired: 8 in]
        n572 = call "Digitizer2_FGV.vi"("error in (no error)"=w1235, "Operation (Read)"=enum16{"Write", "Read"}."Read" ("Operation")) -> ("error out"=w1238:errorcluster, "Read data"=w1240:refnum<k15>)  [unwired: 8 in]
        n573 = call <instrlib>:"niScope Abort.vi"("instrument handle"=w1239, "error in"=w1242) -> ("error out"=w1244:errorcluster)  [unwired: 12 in, 1 out]
        n574 = call <instrlib>:"niScope Abort.vi"("instrument handle"=w1240, "error in"=w1238) -> ("error out"=w1243:errorcluster)  [unwired: 12 in, 1 out]
        n575 = Merge Errors(w1244, w1243) -> (w1236:errorcluster)
        n576 = call <vilib>:"Add State(s) to Queue__JKI_lib_State_Machine.vi"("State(s) in (\"\")"=w1247) -> ("States Out"=w1246:string)  [unwired: 14 in]
      }
      frame "Digitizer: checkTemp" {
        w1255 = enum16{"Write", "Read"}."Read" ("Operation")
        # "Template Separator\n(You can make a copy of, or modify, this frame)"
        n577 = call "Digitizer1_FGV.vi"("error in (no error)"=w1251, "Operation (Read)"=w1255) -> ("error out"=w1257:errorcluster, "Read data"=w1258:refnum<k15>)  [unwired: 8 in]
        n578 = call "Digitizer2_FGV.vi"("error in (no error)"=w1251, "Operation (Read)"=w1255) -> ("error out"=w1253:errorcluster, "Read data"=w1254:refnum<k15>)  [unwired: 8 in]
        n579 = property on="Property Node" class="niScope"(reference=w1258, error in=w1257) -> (error out=w1249:errorcluster, "Device Temperature"=→"Dig1 Temp":dbl)  [unwired: 1 out]
        n580 = property on="Property Node" class="niScope"(reference=w1254, error in=w1253) -> (error out=w1248:errorcluster, "Device Temperature"=→"Dig2 Temp":dbl)  [unwired: 1 out]
        n581 = Merge Errors(w1249, w1248) -> (w1250:errorcluster)
        n582 = call <vilib>:"Add State(s) to Queue__JKI_lib_State_Machine.vi"("State(s) in (\"\")"=w1262) -> ("States Out"=w1261:string)  [unwired: 14 in]
      }
      frame "Digitizer: Close" {
        # "Close Digitizer"
        n583 = call "Digitizer1_FGV.vi"("error in (no error)"=w1270, "Operation (Read)"=enum16{"Write", "Read"}."Read" ("Operation")) -> ("error out"=w1272:errorcluster, "Read data"=w1276:refnum<k15>)  [unwired: 8 in]
        n584 = call "Digitizer2_FGV.vi"("error in (no error)"=w1270, "Operation (Read)"=enum16{"Write", "Read"}."Read" ("Operation")) -> ("error out"=w1271:errorcluster, "Read data"=w1274:refnum<k15>)  [unwired: 8 in]
        n585 = call <instrlib>:"niScope Close.vi"("instrument handle"=w1276, "error in"=w1272) -> ("error out"=w1269:errorcluster)  [unwired: 13 in]
        n586 = call <instrlib>:"niScope Close.vi"("instrument handle"=w1274, "error in"=w1271) -> ("error out"=w1268:errorcluster)  [unwired: 13 in]
        n587 = Merge Errors(w1269, w1268) -> (w1267:errorcluster)
        n588 = Unbundle By Name(w1267) -> ("status"=w1266:bool)
        n589 = Bundle By Name(cluster=w1264, "System Status.Digitizer"=w1266) -> (w1263:T22)
        n590 = call <vilib>:"Add State(s) to Queue__JKI_lib_State_Machine.vi"("State(s) in (\"\")"=w1278) -> ("States Out"=w1277:string)  [unwired: 14 in]
      }
      frame "---------- LabJack ----------" {
        # "Template Separator\n(You can make a copy of, or modify, this frame)"
        n591 = call <vilib>:"Add State(s) to Queue__JKI_lib_State_Machine.vi"("State(s) in (\"\")"=w1283) -> ("States Out"=w1282:string)  [unwired: 14 in]
      }
      frame "LabJack: AB_DC_Start" {
        # "Template Separator\n(You can make a copy of, or modify, this frame)"
        n592 = Unbundle By Name(w1287) -> ("LJ Pinout.AimingBeam PWM"=w1286:string)
        n593 = call "LabJack_FGV.vi"("Operation(Read)"=enum16{"Write", "Read"}."Read", "error in (no error)"=w1290) -> ("error out"=w1288:errorcluster, "Read data"=w1289:i32)  [unwired: 8 in]
        n594 = call "LJM_eWriteName.vi"("Handle In"=w1289, "Name"=w1286, "Value"=1.0, "error in"=w1288) -> ("error out"=w1284:errorcluster)  [unwired: 10 in, 1 out]
        n595 = call <vilib>:"Add State(s) to Queue__JKI_lib_State_Machine.vi"("State(s) in (\"\")"=w1294) -> ("States Out"=w1293:string)  [unwired: 14 in]
      }
      frame "LabJack: AB_DC_Stop" {
        # "Template Separator\n(You can make a copy of, or modify, this frame)"
        n596 = Unbundle By Name(w1298) -> ("LJ Pinout.AimingBeam PWM"=w1297:string)
        n597 = call "LabJack_FGV.vi"("Operation(Read)"=enum16{"Write", "Read"}."Read", "error in (no error)"=w1301) -> ("error out"=w1299:errorcluster, "Read data"=w1300:i32)  [unwired: 8 in]
        n598 = call "LJM_eWriteName.vi"("Handle In"=w1300, "Name"=w1297, "Value"=0.0, "error in"=w1299) -> ("error out"=w1295:errorcluster)  [unwired: 10 in, 1 out]
        n599 = call <vilib>:"Add State(s) to Queue__JKI_lib_State_Machine.vi"("State(s) in (\"\")"=w1305) -> ("States Out"=w1304:string)  [unwired: 14 in]
      }
      frame "LabJack: checkPedal" {
        # "Template Separator\n(You can make a copy of, or modify, this frame)"
        n600 = Unbundle By Name(w1310) -> ("LJ Pinout.Foot Pedal"=w1312:string)
        n601 = local read "Tab Control"() -> (w1309:T2)
        n602 = call "LabJack_FGV.vi"("Operation(Read)"=enum16{"Write", "Read"}."Read" ("Operation"), "error in (no error)"=w1314) -> ("error out"=w1316:errorcluster, "Read data"=w1317:i32)  [unwired: 8 in]
        n603 = Equal?(x=w1309, y=T12."IO Ststus" ("Tab Control")) -> (x = y?=w1307:bool)
        n604 = call "LJM_eReadName.vi"("Handle In"=w1317, "Name"=w1312, "error in"=w1316) -> ("Value"=w1306:dbl, "error out"=w1315:errorcluster)  [unwired: 10 in, 1 out]
        n605 = case shown="True" w1307 {
          tunnel: w1306 -> [_ w1326]
          frame False {
          }
          frame True {
            # "[Covers: REQ14]"
            # "If on IO tab, show foot pedal status"
            n606 = Equal To 0?(x=w1326) -> (x = 0?=w1325:bool)
            n607 = Select(t=FALSE, s=w1325, f=TRUE) -> (s? t:f=w1324:bool)
            n608 = local write "Foot Pedal"(w1324) -> ()
          }
        }
        n609 = case shown="1" w1306 {
          tunnel: [w1327 w1332] -> w1311
          tunnel: ["" ("State(s) in Front (\"\")") w1331] -> w1313
          tunnel: w1310 -> [w1327 w1330]
          frame 0, Default {
          }
          frame 1 {
            # "If Pedal pressed"
            n610 = Unbundle By Name(w1330) -> ("Last Trigger"=w1329:u32)
            n611 = Tick Count (ms)() -> (millisecond timer value=w1336:u32)
            n612 = Subtract(x=w1336, y=w1329) -> (x-y=w1335:u32)
            n613 = Greater Or Equal?(x=w1335, y=u32 2000) -> (x >= y?=w1333:bool)
            n614 = case shown="True" w1333 {
              tunnel: [w1337 w1342] -> w1332
              tunnel: ["" ("State(s) in Front (\"\")") w1341] -> w1331
              tunnel: w1330 -> [w1337 w1339]
              frame False {
              }
              frame True {
                n615 = Tick Count (ms)() -> (millisecond timer value=w1343:u32)
                n616 = Unbundle By Name(w1339) -> ("SysRunning?"=w1340:bool)
                n617 = case shown="True" w1340 {
                  tunnel: ["Macro: StartRun" ("State(s) in Front (\"\")") "Macro: StopRun" ("State(s) in Front (\"\")")] -> w1341
                  frame False {
                  }
                  frame True {
                  }
                }
                n618 = Bundle By Name(cluster=w1339, "Last Trigger"=w1343) -> (w1342:T22)
              }
            }
          }
        }
        n619 = call <vilib>:"Add State(s) to Queue__JKI_lib_State_Machine.vi"("State(s) in Front (\"\")"=w1313, "State(s) in (\"\")"=w1321) -> ("States Out"=w1320:string)  [unwired: 13 in]
      }
      frame "LabJack: ZeroV" {
        # "Just Zero V\nDO not update FGV and front panel\nWIll resume from last V"
        # "set bias to 0"
        # "Zero APD bias\n(You can make a copy of, or modify, this frame)"
        n620 = Unbundle By Name(w1347) -> ("LJ Pinout.Ch1 Bias"=w1353:string, "LJ Pinout.Ch2 Bias"=w1352:string, "LJ Pinout.Ch3 Bias"=w1351:string)
        n621 = Build Array(w1353, w1352, w1351) -> (w1346:string[])
        n622 = call "LabJack_FGV.vi"("Operation(Read)"=enum16{"Write", "Read"}."Read" ("Operation"), "error in (no error)"=w1349) -> ("error out"=w1354:errorcluster, "Read data"=w1355:i32)  [unwired: 8 in]
        n623 = call "LJM_eWriteNames.vi"("Handle In"=w1355, "aNames"=w1346, "aValuesIn"=dbl[] [0.0, 0.0, 0.0], "error in"=w1354) -> ("error out"=w1348:errorcluster)  [unwired: 9 in, 2 out]
        n624 = call <vilib>:"Add State(s) to Queue__JKI_lib_State_Machine.vi"("State(s) in (\"\")"=w1359) -> ("States Out"=w1358:string)  [unwired: 14 in]
      }
      frame "LabJack: SetV" {
        # "set bias to user specifid"
        # "Zero APD bias\n(You can make a copy of, or modify, this frame)"
        n625 = Unbundle By Name(w1363) -> ("LJ Pinout.Ch1 Bias"=w1367:string, "LJ Pinout.Ch2 Bias"=w1365:string, "LJ Pinout.Ch3 Bias"=w1364:string)
        n626 = local read "Channel"() -> (w1368:enum32{"Ch1", "Ch2", "Ch3"})
        n627 = call "V1FGV.vi"("Error In"=w1371, "action (write)"=enum16{"write", "read"}."read" ("action")) -> ("Error Out"=w1360:errorcluster, "V1 out"=w1366:dbl)  [unwired: 8 in]
        n628 = local write "Ctrl V"(w1366) -> ()
        n629 = case shown="\"Ch1\", Default" w1368 {
          tunnel: w1367 -> [w1377 _ _]
          tunnel: [w1377 w1378 w1379] -> w1362
          tunnel: w1365 -> [_ w1378 _]
          tunnel: w1364 -> [_ _ w1379]
          frame "Ch1", Default {
          }
          frame "Ch2" {
          }
          frame "Ch3" {
          }
        }
        n630 = call "LabJack_FGV.vi"("error in (no error)"=w1371) -> ("error out"=w1372:errorcluster, "Read data"=w1373:i32)  [unwired: 9 in]
        n631 = call "LJM_eWriteName.vi"("Handle In"=w1373, "Name"=w1362, "Value"=w1366, "error in"=w1372) -> ("error out"=w1369:errorcluster)  [unwired: 10 in, 1 out]
        n632 = Merge Errors(w1360, w1369) -> (w1370:errorcluster)
        n633 = call <vilib>:"Add State(s) to Queue__JKI_lib_State_Machine.vi"("State(s) in (\"\")"=w1376) -> ("States Out"=w1375:string)  [unwired: 14 in]
      }
      frame "LabJack: Open" {
        # "Initialize LabJack T7\nEstablish connection and initialize pins"
        n634 = call "LJ_Open.vi"("error in"=w1388) -> ("error out"=w1386:errorcluster, "Success?"=w1387:bool, "Handle Out"=w1384:i32)  [unwired: 8 in]
        n635 = call "LabJack_FGV.vi"("Operation(Read)"=enum16{"Write", "Read"}."Write" ("Operation"), "error in (no error)"=w1386, "Write data"=w1384) -> ("error out"=w1383:errorcluster)  [unwired: 7 in, 1 out]
        n636 = Bundle By Name(cluster=w1380, "System Status.Labjack"=w1387) -> (w1381:T22)
        n637 = call <vilib>:"Add State(s) to Queue__JKI_lib_State_Machine.vi"("State(s) in (\"\")"=w1390) -> ("States Out"=w1389:string)  [unwired: 14 in]
      }
      frame "LabJack: SetDefaultSub" {
        w1401 = enum16{"write", "read"}."write" ("action")
        w1414 = "_EF_ENABLE" ("string")
        # "1. Disable PWM\n2. Set all V to 0\n3. Set 355 relay to open\n4. Set LED to off"
        # "read once to set DIO to input"
        # "set all initila V to 0. Set footpedal to input. Set PWM to low. Set laser relay to open. Set LEDs to yellow."
        # "Set Labjack to correct input and output state and initial values"
        n638 = Unbundle By Name(w1400) -> ("LJ Pinout.355 PWM"=w1392:string, "LJ Pinout.AimingBeam PWM"=w1391:string, "LJ Pinout.Ch1 Bias"=w1398:string, "LJ Pinout.Ch2 Bias"=w1397:string, "LJ Pinout.Ch3 Bias"=w1396:string, "LJ Pinout.Laser Start/Stop"=w1395:string, "LJ Pinout.Red LED"=w1394:string, "LJ Pinout.Green LED"=w1393:string)
        n639 = call "V1FGV.vi"("Error In"=w1408, "action (write)"=w1401, "V1 in"=0.0) -> ("Error Out"=w1409:errorcluster, "V1 out"=w1402:dbl)  [unwired: 7 in]
        n640 = call "LabJack_FGV.vi"("Operation(Read)"=enum16{"Write", "Read"}."Read" ("Operation"), "error in (no error)"=w1408) -> ("error out"=w1417:errorcluster, "Read data"=w1418:i32)  [unwired: 8 in]
        n641 = local write "Ctrl V"(w1402) -> ()
        n642 = call "V2FGV.vi"("Error In"=w1409, "action(write)"=w1401, "V2 in"=0.0) -> ("Error Out"=w1406:errorcluster)  [unwired: 7 in, 1 out]
        n643 = Concatenate Strings(w1392, w1414) -> (w1413:string)
        n644 = Concatenate Strings(w1391, w1414) -> (w1412:string)
        n645 = call "V3FGV.vi"("Error In"=w1406, "action(write)"=w1401, "V3 in"=0.0) -> ("Error Out"=w1403:errorcluster)  [unwired: 7 in, 1 out]
        n646 = Build Array(w1392, w1391, w1413, w1412, w1398, w1397, w1396, w1395, w1394, w1393) -> (w1421:string[])
        n647 = Unbundle By Name(w1400) -> ("LJ Pinout.Foot Pedal"=w1399:string)
        n648 = call "LJM_eWriteNames.vi"("Handle In"=w1418, "aNames"=w1421, "aValuesIn"=dbl[] [0.0, 0.0, 0.0, 0.0, 0.0, 0.0, 0.0, 0.0, 0.0, 0.0], "error in"=w1417) -> ("Handle Out"=w1416:i32, "error out"=w1415:errorcluster)  [unwired: 9 in, 1 out]
        n649 = call "LJM_eReadName.vi"("Handle In"=w1416, "Name"=w1399, "error in"=w1415) -> ("error out"=w1405:errorcluster)  [unwired: 10 in, 2 out]
        n650 = Merge Errors(w1405, w1403) -> (w1404:errorcluster)
        n651 = call <vilib>:"Add State(s) to Queue__JKI_lib_State_Machine.vi"("State(s) in (\"\")"=w1424) -> ("States Out"=w1423:string)  [unwired: 14 in]
      }
      frame "LabJack: FootPedalConfig" {
        # "Setup footPedal\n(You can make a copy of, or modify, this frame)"
        n652 = call "LabJack_FGV.vi"("Operation(Read)"=enum16{"Write", "Read"}."Read" ("Operation"), "error in (no error)"=w1426) -> ("error out"=w1430:errorcluster, "Read data"=w1431:i32)  [unwired: 8 in]
        n653 = call "LJM_eWriteName.vi"("Handle In"=w1431, "Name"="DIO15", "Value"=1.0, "error in"=w1430) -> ("error out"=w1427:errorcluster)  [unwired: 10 in, 1 out]
        n654 = call <vilib>:"Add State(s) to Queue__JKI_lib_State_Machine.vi"("State(s) in (\"\")"=w1435) -> ("States Out"=w1434:string)  [unwired: 14 in]
      }
      frame "LabJack: SetDefaultAndClose" {
        # "Template Separator\n(You can make a copy of, or modify, this frame)"
        n655 = call <vilib>:"Add State(s) to Queue__JKI_lib_State_Machine.vi"("State(s) in Front (\"\")"="LabJack: SetDefaultSub\nLabJack: Close" ("State(s) in Front (\"\")"), "State(s) in (\"\")"=w1441) -> ("States Out"=w1440:string)  [unwired: 13 in]
      }
      frame "LabJack: Close" {
        # "Close LabJack Refnum"
        n656 = call "LabJack_FGV.vi"("Operation(Read)"=enum16{"Write", "Read"}."Read" ("Operation"), "error in (no error)"=w1448) -> ("error out"=w1444:errorcluster, "Read data"=w1445:i32)  [unwired: 8 in]
        n657 = Bundle By Name(cluster=w1442, "System Status.Labjack"=FALSE ("System Status.Gain Control")) -> (w1443:T22)
        n658 = call "LJM_Close.vi"("error in"=w1444, "Handle"=w1445) -> ("error out"=w1450:errorcluster)  [unwired: 9 in]
        n659 = call <vilib>:"Add State(s) to Queue__JKI_lib_State_Machine.vi"("State(s) in (\"\")"=w1452) -> ("States Out"=w1451:string)  [unwired: 14 in]
      }
      frame "LabJack: Interlock enable/disable" {
        w1461 = i8 0  # int8
        # "Interlock enable/disable\n(Usage: \"LabJack: Interlock enable/disable >> 1|0\")"
        n660 = Fract/Exp String To Number(string=w1462, default (0 dbl)=w1461) -> (number=w1460:i8)  [unwired: 2 in, 1 out]
        n661 = Unbundle By Name(w1454) -> ("LJ Pinout.Interlock"=w1453:string)
        n662 = call "LabJack_FGV.vi"("Operation(Read)"=enum16{"Write", "Read"}."Read" ("Operation")) -> ("Read data"=w1458:i32)  [unwired: 9 in, 1 out]
        n663 = call "LJM_eWriteName.vi"("Handle In"=w1458, "Name"=w1453, "Value"=w1460, "error in"=w1459) -> ("error out"=w1456:errorcluster)  [unwired: 10 in, 1 out]
        n664 = call <vilib>:"Add State(s) to Queue__JKI_lib_State_Machine.vi"("State(s) in (\"\")"=w1464) -> ("States Out"=w1463:string)  [unwired: 14 in]
      }
      frame "LabJack: 355_PWM_Config" {
        w1474 = 0.0 ("element")
        w1487 = "DIO_EF_CLOCK1_ENABLE"
        # "Config PWM frequency"
        n665 = Unbundle By Name(w1472) -> ("LJ Pinout.355 PWM"=w1466:string)
        n666 = Unbundle By Name(w1472) -> ("355 PWM setting.DIO_EF_CLOCK1_DIVISOR"=w1471:i16, "355 PWM setting.DIO_EF_CLOCK1_ROLL_VALUE"=w1470:i32, "355 PWM setting.DIO#_EF_INDEX"=w1469:i16, "355 PWM setting.DIO#_EF_OPTIONS"=w1468:i16, "355 PWM setting.DIO#_EF_CONFIG_A"=w1467:i32)
        n667 = Concatenate Strings(w1466, "_EF_ENABLE" ("string")) -> (w1483:string)
        n668 = Concatenate Strings(w1466, "_EF_INDEX") -> (w1486:string)
        n669 = Concatenate Strings(w1466, "_EF_OPTIONS") -> (w1485:string)
        n670 = Concatenate Strings(w1466, "_EF_CONFIG_A") -> (w1484:string)
        n671 = call "LabJack_FGV.vi"("Operation(Read)"=enum16{"Write", "Read"}."Read" ("Operation")) -> ("Read data"=w1481:i32)  [unwired: 9 in, 1 out]
        n672 = Build Array(w1474, w1474, w1471, w1470, 1.0 ("element"), 0.0 ("element"), w1469, w1468, w1467) -> (w1478:dbl[])
        n673 = Build Array("DIO_EF_CLOCK0_ENABLE", w1487, "DIO_EF_CLOCK1_DIVISOR", "DIO_EF_CLOCK1_ROLL_VALUE", w1487, w1483, w1486, w1485, w1484) -> (w1482:string[])
        n674 = call "LJM_eWriteNames.vi"("Handle In"=w1481, "aNames"=w1482, "aValuesIn"=w1478, "error in"=w1476) -> ("error out"=w1477:errorcluster)  [unwired: 9 in, 2 out]
        n675 = call <vilib>:"Add State(s) to Queue__JKI_lib_State_Machine.vi"("State(s) in (\"\")"=w1495) -> ("States Out"=w1494:string)  [unwired: 14 in]
      }
      frame "LabJack: AB_PWM_Config" {
        w1507 = 0.0 ("element")
        w1518 = "DIO_EF_CLOCK2_ENABLE"
        # "Set PWM to ground so AB is disabled"
        # "Config PWM frequency"
        n676 = Unbundle By Name(w1505) -> ("LJ Pinout.AimingBeam PWM"=w1496:string)
        n677 = Unbundle By Name(w1505) -> ("AB PWM setting.DIO_EF_CLOCK1_DIVISOR"=w1504:i16, "AB PWM setting.DIO_EF_CLOCK1_ROLL_VALUE"=w1503:i32, "AB PWM setting.DIO#_EF_INDEX"=w1502:i16, "AB PWM setting.DIO#_EF_OPTIONS"=w1501:i16, "AB PWM setting.DIO#_EF_CONFIG_A"=w1500:i32)
        n678 = Concatenate Strings(w1496, "_EF_ENABLE" ("string")) -> (w1514:string)
        n679 = Concatenate Strings(w1496, "_EF_INDEX") -> (w1517:string)
        n680 = Concatenate Strings(w1496, "_EF_OPTIONS") -> (w1516:string)
        n681 = Concatenate Strings(w1496, "_EF_CONFIG_A") -> (w1515:string)
        n682 = Build Array(w1507, w1507, w1504, w1503, 1.0 ("element"), 0.0 ("element"), w1502, w1501, w1500) -> (w1510:dbl[])
        n683 = call "LabJack_FGV.vi"("Operation(Read)"=enum16{"Write", "Read"}."Read" ("Operation"), "error in (no error)"=w1497) -> ("error out"=w1498:errorcluster, "Read data"=w1499:i32)  [unwired: 8 in]
        n684 = Build Array("DIO_EF_CLOCK0_ENABLE", w1518, "DIO_EF_CLOCK2_DIVISOR", "DIO_EF_CLOCK2_ROLL_VALUE", w1518, w1514, w1517, w1516, w1515) -> (w1513:string[])
        n685 = call "LJM_eWriteNames.vi"("Handle In"=w1499, "aNames"=w1513, "aValuesIn"=w1510, "error in"=w1498) -> ("error out"=w1509:errorcluster)  [unwired: 9 in, 2 out]
        n686 = call <vilib>:"Add State(s) to Queue__JKI_lib_State_Machine.vi"("State(s) in (\"\")"=w1527) -> ("States Out"=w1526:string)  [unwired: 14 in]
      }
      frame "LabJack: 355_PWM_Start" {
        # "Template Separator\n(You can make a copy of, or modify, this frame)"
        n687 = Unbundle By Name(w1529) -> ("LJ Pinout.355 PWM"=w1528:string)
        n688 = call "LabJack_FGV.vi"("Operation(Read)"=enum16{"Write", "Read"}."Read" ("Operation"), "error in (no error)"=w1531) -> ("error out"=w1536:errorcluster, "Read data"=w1537:i32)  [unwired: 8 in]
        n689 = Concatenate Strings(w1528, "_EF_ENABLE" ("string")) -> (w1534:string)
        n690 = call "LJM_eWriteName.vi"("Handle In"=w1537, "Name"=w1534, "Value"=1.0, "error in"=w1536) -> ("error out"=w1532:errorcluster)  [unwired: 10 in, 1 out]
        n691 = call <vilib>:"Add State(s) to Queue__JKI_lib_State_Machine.vi"("State(s) in (\"\")"=w1540) -> ("States Out"=w1539:string)  [unwired: 14 in]
      }
      frame "LabJack: AB_PWM_Start" {
        # "Template Separator\n(You can make a copy of, or modify, this frame)"
        n692 = Unbundle By Name(w1542) -> ("LJ Pinout.AimingBeam PWM"=w1541:string)
        n693 = call "LabJack_FGV.vi"("Operation(Read)"=enum16{"Write", "Read"}."Read" ("Operation"), "error in (no error)"=w1544) -> ("error out"=w1549:errorcluster, "Read data"=w1550:i32)  [unwired: 8 in]
        n694 = Concatenate Strings(w1541, "_EF_ENABLE" ("string")) -> (w1547:string)
        n695 = call "LJM_eWriteName.vi"("Handle In"=w1550, "Name"=w1547, "Value"=1.0, "error in"=w1549) -> ("error out"=w1545:errorcluster)  [unwired: 10 in, 1 out]
        n696 = call <vilib>:"Add State(s) to Queue__JKI_lib_State_Machine.vi"("State(s) in (\"\")"=w1553) -> ("States Out"=w1552:string)  [unwired: 14 in]
      }
      frame "LabJack: 355_PWM_Stop" {
        # "Template Separator\n(You can make a copy of, or modify, this frame)"
        n697 = Unbundle By Name(w1556) -> ("LJ Pinout.355 PWM"=w1555:string)
        n698 = call "LabJack_FGV.vi"("Operation(Read)"=enum16{"Write", "Read"}."Read" ("Operation"), "error in (no error)"=w1561) -> ("error out"=w1564:errorcluster, "Read data"=w1559:i32)  [unwired: 8 in]
        n699 = Concatenate Strings(w1555, "_EF_ENABLE" ("string")) -> (w1562:string)
        n700 = call "LJM_eWriteName.vi"("Handle In"=w1559, "Name"=w1562, "Value"=0.0, "error in"=w1564) -> ("error out"=w1557:errorcluster)  [unwired: 10 in, 1 out]
        n701 = local write "355nm Laser toggle"(FALSE ("355nm Laser toggle")) -> ()
        n702 = call <vilib>:"Add State(s) to Queue__JKI_lib_State_Machine.vi"("State(s) in (\"\")"=w1567) -> ("States Out"=w1566:string)  [unwired: 14 in]
      }
      frame "LabJack: AB_PWM_Stop" {
        # "Template Separator\n(You can make a copy of, or modify, this frame)"
        n703 = Unbundle By Name(w1569) -> ("LJ Pinout.AimingBeam PWM"=w1568:string)
        n704 = call "LabJack_FGV.vi"("Operation(Read)"=enum16{"Write", "Read"}."Read" ("Operation"), "error in (no error)"=w1572) -> ("error out"=w1577:errorcluster, "Read data"=w1578:i32)  [unwired: 8 in]
        n705 = Concatenate Strings(w1568, "_EF_ENABLE" ("string")) -> (w1575:string)
        n706 = call "LJM_eWriteName.vi"("Handle In"=w1578, "Name"=w1575, "Value"=0.0, "error in"=w1577) -> ("error out"=w1573:errorcluster)  [unwired: 10 in, 1 out]
        n707 = local write "Aiming beam toggle"(FALSE ("Aiming beam toggle")) -> ()
        n708 = call <vilib>:"Add State(s) to Queue__JKI_lib_State_Machine.vi"("State(s) in (\"\")"=w1581) -> ("States Out"=w1580:string)  [unwired: 14 in]
      }
      frame "---------- LED ----------" {
        # "Template Separator\n(You can make a copy of, or modify, this frame)"
        n709 = call <vilib>:"Add State(s) to Queue__JKI_lib_State_Machine.vi"("State(s) in (\"\")"=w1586) -> ("States Out"=w1585:string)  [unwired: 14 in]
      }
      frame "LED: BreathGreen" {
        w1589 = FALSE ("Wait Until Done")
        # "breath LED Green\n(Run VI in background using VI server to breath LED green )"
        n710 = Unbundle By Name(w1595) -> ("LED vi reference"=w1594:refnum<vi>)
        n711 = invoke class="VI" method="Ctrl Val.Set"(reference=w1594, error in=w1587, "Control Name"="Color", "Value"=0) -> (reference out=w1591:refnum<vi>, error out=w1590:errorcluster)  [unwired: 1 in, 3 out]
        n712 = invoke class="VI" method="Run VI"(reference=w1591, error in=w1590, "Wait until done"=w1589, "Auto Dispose Ref"=w1589) -> (error out=w1588:errorcluster)  [unwired: 1 in, 4 out]
        n713 = call <vilib>:"Add State(s) to Queue__JKI_lib_State_Machine.vi"("State(s) in (\"\")"=w1598) -> ("States Out"=w1597:string)  [unwired: 14 in]
      }
      frame "LED: BreathOrange" {
        w1601 = FALSE ("Wait Until Done")
        # "breath LED Green\n(Run VI in background using VI server to breath LED green )"
        n714 = Unbundle By Name(w1607) -> ("LED vi reference"=w1606:refnum<vi>)
        n715 = invoke class="VI" method="Ctrl Val.Set"(reference=w1606, error in=w1599, "Control Name"="Color", "Value"=1) -> (reference out=w1603:refnum<vi>, error out=w1602:errorcluster)  [unwired: 1 in, 3 out]
        n716 = invoke class="VI" method="Run VI"(reference=w1603, error in=w1602, "Wait until done"=w1601, "Auto Dispose Ref"=w1601) -> (error out=w1600:errorcluster)  [unwired: 1 in, 4 out]
        n717 = call <vilib>:"Add State(s) to Queue__JKI_lib_State_Machine.vi"("State(s) in (\"\")"=w1610) -> ("States Out"=w1609:string)  [unwired: 14 in]
      }
      frame "LED: OpenVIRef" {
        # "Open LED vi ref\n(You can make a copy of, or modify, this frame)"
        n718 = call <vilib>:"Application Directory.vi"() -> ("Application Directory"=w1615:path)
        n719 = Build Path(base path=w1615, name or relative path="SubVI") -> (appended path=w1613:path)
        n720 = Build Path(base path=w1613, name or relative path="LEDBreath.vi") -> (appended path=w1611:path)
        n721 = Open VI Reference(vi path=w1611, error in (no error)=w1620) -> (vi reference=w1617:refnum<vi>, error out=w1619:errorcluster)  [unwired: 4 in]
        n722 = case shown="No Error" w1619 {
          tunnel: w1618 -> [w1624 w1628]
          tunnel: w1617 -> [w1627 _]
          tunnel: [w1625 w1628] -> w1616
          frame No Error {
            n723 = Bundle By Name(cluster=w1624, "LED vi reference"=w1627, "LedViRefOpen"=TRUE) -> (w1625:T22)
          }
          frame Error {
          }
        }
        n724 = call <vilib>:"Add State(s) to Queue__JKI_lib_State_Machine.vi"("State(s) in (\"\")"=w1623) -> ("States Out"=w1622:string)  [unwired: 14 in]
      }
      frame "LED: CloseVIRef" {
        # "Template Separator\n(You can make a copy of, or modify, this frame)"
        n725 = Unbundle By Name(w1630) -> ("LedViRefOpen"=w1629:bool, "LED vi reference"=w1632:refnum<vi>)
        n726 = case shown="True" w1629 {
          tunnel: w1633 -> [w1637 w1640]
          tunnel: w1632 -> [_ w1638]
          tunnel: [w1637 w1639] -> w1631
          frame False {
          }
          frame True {
            n727 = Close Reference(reference=w1638, error in (no error)=w1640) -> (error out=w1639:errorcluster)
          }
        }
        n728 = call <vilib>:"Add State(s) to Queue__JKI_lib_State_Machine.vi"("State(s) in (\"\")"=w1636) -> ("States Out"=w1635:string)  [unwired: 14 in]
      }
      frame "LED: BreathOff" {
        # "System LED Breath Off\n(LED breath off"
        n729 = Unbundle By Name(w1647) -> ("LED vi reference"=w1649:refnum<vi>)
        n730 = invoke on="Invoke Node" class="VI" method="Ctrl Val.Set"(reference=w1649, error in=w1648, "Control Name"="Stop", "Value"=TRUE) -> (reference out=w1643:refnum<vi>, error out=w1644:errorcluster)  [unwired: 1 in, 3 out]
        n731 = case shown="No Error" w1644 {
          selector: w1644 -> [w1654 _]
          tunnel: [w1653 errorcluster {"status"=FALSE, "code"=0, "source"=""} ("error IO")] -> w1641
          tunnel: ["" ("State(s) in Front (\"\")") "LED: BreathOff" ("State(s) in Front (\"\")")] -> w1642
          tunnel: w1643 -> [w1655 _]
          frame No Error {
            # "No error, wait for VI to stop"
            n732 = while {
              tunnel: w1655 -> [w1663]
              shift-right: [w1657] -> w1653
              shift-left: w1654 -> [w1662]
              stop <- w1659 stop-if-true
              # "continue check whether vi is running"
              n733 = property class="VI"(reference=w1663, error in=w1662) -> (error out=w1657:errorcluster, "Exec.State"=w1661:T18)  [unwired: 1 out]
              n734 = Wait (ms)(milliseconds to wait=u32 50) -> ()  [unwired: 1 out]
              n735 = Equal?(x=w1661, y=T18."Idle") -> (x = y?=w1659:bool)
            }
          }
          frame Error {
            # "try again when error"
          }
        }
        n736 = call <vilib>:"Add State(s) to Queue__JKI_lib_State_Machine.vi"("State(s) in Front (\"\")"=w1642, "State(s) in (\"\")"=w1652) -> ("States Out"=w1651:string)  [unwired: 13 in]
      }
      frame "LED: Off" {
        # "set LED to red"
        # "Template Separator\n(You can make a copy of, or modify, this frame)"
        n737 = Unbundle By Name(w1668) -> ("LJ Pinout.Red LED"=w1667:string, "LJ Pinout.Green LED"=w1666:string)
        n738 = call "LabJack_FGV.vi"("Operation(Read)"=enum16{"Write", "Read"}."Read" ("Operation"), "error in (no error)"=w1669) -> ("error out"=w1676:errorcluster, "Read data"=w1675:i32)  [unwired: 8 in]
        n739 = call "LJM_eWriteName.vi"("Handle In"=w1675, "Name"=w1667, "Value"=0.0, "error in"=w1676) -> ("Handle Out"=w1673:i32, "error out"=w1672:errorcluster)  [unwired: 10 in]
        n740 = call "LJM_eWriteName.vi"("Handle In"=w1673, "Name"=w1666, "Value"=0.0, "error in"=w1672) -> ("error out"=w1670:errorcluster)  [unwired: 10 in, 1 out]
        n741 = call <vilib>:"Add State(s) to Queue__JKI_lib_State_Machine.vi"("State(s) in (\"\")"=w1680) -> ("States Out"=w1679:string)  [unwired: 14 in]
      }
      frame "LED: Green" {
        # "set LED to green"
        # "Template Separator\n(You can make a copy of, or modify, this frame)"
        n742 = Unbundle By Name(w1683) -> ("LJ Pinout.Red LED"=w1682:string, "LJ Pinout.Green LED"=w1681:string)
        n743 = call "LabJack_FGV.vi"("Operation(Read)"=enum16{"Write", "Read"}."Read" ("Operation"), "error in (no error)"=w1686) -> ("error out"=w1692:errorcluster, "Read data"=w1691:i32)  [unwired: 8 in]
        n744 = call "LJM_eWriteName.vi"("Handle In"=w1691, "Name"=w1682, "Value"=0.0, "error in"=w1692) -> ("Handle Out"=w1689:i32, "error out"=w1688:errorcluster)  [unwired: 10 in]
        n745 = call "LJM_eWriteName.vi"("Handle In"=w1689, "Name"=w1681, "Value"=9.0, "error in"=w1688) -> ("error out"=w1685:errorcluster)  [unwired: 10 in, 1 out]
        n746 = call <vilib>:"Add State(s) to Queue__JKI_lib_State_Machine.vi"("State(s) in (\"\")"=w1695) -> ("States Out"=w1694:string)  [unwired: 14 in]
      }
      frame "---------- Queue ----------" {
        # "Template Separator\n(You can make a copy of, or modify, this frame)"
        n747 = call <vilib>:"Add State(s) to Queue__JKI_lib_State_Machine.vi"("State(s) in (\"\")"=w1700) -> ("States Out"=w1699:string)  [unwired: 14 in]
      }
      frame "Queue: CheckCtrlVQ" {
        # "Check control V queue\n(if contorl V queue is not empty, aquire data)"
        n748 = Unbundle By Name(w1705) -> ("SysRunning?"=w1704:bool)
        n749 = case shown="False" w1704 {
          tunnel: w1701 -> [w1717 w1734]
          tunnel: w1706 -> [w1716 _]
          tunnel: [w1712 "" ("State with Arguments")] -> w1703
          tunnel: [w1710 w1734] -> w1702
          frame False {
            # "system idle"
            n750 = Get Queue Status(queue=w1716, error in (no error)=w1717) -> (queue out=w1714:refnum<queue>, error out=w1713:errorcluster, # elements in queue=w1711:i32)  [unwired: 1 in, 5 out]
            n751 = Greater Than 0?(x=w1711) -> (x > 0?=w1715:bool)
            n752 = case shown="True" w1715 {
              tunnel: w1714 -> [_ w1731]
              tunnel: w1713 -> [w1718 w1730]
              tunnel: ["" ("State with Arguments") w1722] -> w1712
              tunnel: w1711 -> [_ w1726]
              tunnel: [w1718 w1720] -> w1710
              frame False {
              }
              frame True {
                n753 = Dequeue Element(queue=w1731, error in (no error)=w1730) -> (element=w1727:dbl, error out=w1720:errorcluster)  [unwired: 1 in, 2 out]
                n754 = Equal?(x=w1726, y=1) -> (x = y?=w1724:bool)
                n755 = Number To Fractional String(number=w1727) -> (F-format string=w1728:string)  [unwired: 3 in]
                n756 = case shown="True" w1724 {
                  tunnel: ["" ("Empty String Constant") "Data: parseDataAllGainMacro\nMacro: AskOverWrite"] -> w1721
                  frame False {
                  }
                  frame True {
                    # "if last control V, parse all data and ask whether to over-write"
                  }
                }
                n757 = call <vilib>:"Build State String with Arguments__JKI_lib_State_Machine.vi"("Arguments (\"\")"=w1728, "State"="Aquisition: RecordData") -> ("State with Arguments"=w1723:string)  [unwired: 4 in]
                n758 = call <vilib>:"Add State(s) to Queue__JKI_lib_State_Machine.vi"("State(s) in Front (\"\")"=w1723, "State(s) in (\"\")"=w1721) -> ("States Out"=w1722:string)  [unwired: 13 in]
              }
            }
          }
          frame True {
            # "System running"
          }
        }
        n759 = call <vilib>:"Add State(s) to Queue__JKI_lib_State_Machine.vi"("State(s) in Front (\"\")"=w1703, "State(s) in (\"\")"=w1709) -> ("States Out"=w1708:string)  [unwired: 13 in]
      }
      frame "Queue: FlashDataAllQueue" {
        # "Flash control V queue and DataAll queue\n(You can make a copy of, or modify, this frame)"
        n760 = Flush Queue(queue=w1741, error in (no error)=w1738) -> (error out=w1739:errorcluster)  [unwired: 2 out]
        n761 = Flush Queue(queue=w1743, error in (no error)=w1738) -> (error out=w1742:errorcluster)  [unwired: 2 out]
        n762 = Flush Queue(queue=w1737, error in (no error)=w1738) -> (error out=w1736:errorcluster)  [unwired: 2 out]
        n763 = Merge Errors(w1739, w1742, w1736) -> (w1740:errorcluster)
        n764 = call <vilib>:"Add State(s) to Queue__JKI_lib_State_Machine.vi"("State(s) in (\"\")"=w1747) -> ("States Out"=w1746:string)  [unwired: 14 in]
      }
      frame "Queue: CheckNumOfWF" {
        # "Template Separator\n(You can make a copy of, or modify, this frame)"
        n765 = call "FLImDAQ_FGV.vi"() -> ("Read data"=w1750:T4)  [unwired: 10 in, 1 out]
        n766 = Unbundle By Name(w1750) -> ("Waveform to Avg"=w1749:i16)
        n767 = Get Queue Status(queue=w1752) -> (# elements in queue=w1751:i32)  [unwired: 2 in, 7 out]
        n768 = Multiply(x=w1751, y=w1749) -> (x*y=w1748:i32)
        "numWFInQ" <- w1748
        n769 = Greater Or Equal?(x=w1748, y="Num WF to acquire") -> (x >= y?=w1754:bool)
        n770 = case shown="False" w1754 {
          tunnel: ["Queue: CheckNumOfWF" ("State(s) in Front (\"\")") "" ("State(s) in Front (\"\")")] -> w1753
          frame False {
            n771 = Wait (ms)(milliseconds to wait=u32 5) -> ()  [unwired: 1 out]
          }
          frame True {
          }
        }
        n772 = call <vilib>:"Add State(s) to Queue__JKI_lib_State_Machine.vi"("State(s) in Front (\"\")"=w1753, "State(s) in (\"\")"=w1760) -> ("States Out"=w1759:string)  [unwired: 13 in]
      }
      frame "Queue: Create" {
        # "Template Separator\n(You can make a copy of, or modify, this frame)"
        n773 = call <vilib>:"Add State(s) to Queue__JKI_lib_State_Machine.vi"("State(s) in (\"\")"=w1768) -> ("States Out"=w1767:string)  [unwired: 14 in]
      }
      frame "Queue: Flash" {
        # "Clear queue contnet\n(clear queue content by flash it)"
        n774 = Flush Queue(queue=w1772, error in (no error)=w1769) -> (error out=w1771:errorcluster)  [unwired: 2 out]
        n775 = local write "numWFInQ"(0 ("numWFInQ")) -> ()
        n776 = call <vilib>:"Add State(s) to Queue__JKI_lib_State_Machine.vi"("State(s) in (\"\")"=w1776) -> ("States Out"=w1775:string)  [unwired: 14 in]
      }
      frame "Queue: Destory" {
        # "Destory Data Queue\nDistory data queue ref so the aquisition loop stop"
        n777 = Release Queue(queue=w1784, error in (no error)=w1779) -> (error out=w1787:errorcluster)  [unwired: 1 in, 2 out]
        n778 = Release Queue(queue=w1783, error in (no error)=w1779) -> (error out=w1786:errorcluster)  [unwired: 1 in, 2 out]
        n779 = Release Queue(queue=w1781, error in (no error)=w1779) -> (error out=w1780:errorcluster)  [unwired: 1 in, 2 out]
        n780 = Release Queue(queue=w1778, error in (no error)=w1779) -> (error out=w1777:errorcluster)  [unwired: 1 in, 2 out]
        n781 = Merge Errors(w1787, w1786, w1780, w1777) -> (w1785:errorcluster)
        n782 = call <vilib>:"Add State(s) to Queue__JKI_lib_State_Machine.vi"("State(s) in (\"\")"=w1790) -> ("States Out"=w1789:string)  [unwired: 14 in]
      }
      frame "---------- SysConfig ----------" {
        # "Template Separator\n(You can make a copy of, or modify, this frame)"
        n783 = call <vilib>:"Add State(s) to Queue__JKI_lib_State_Machine.vi"("State(s) in (\"\")"=w1795) -> ("States Out"=w1794:string)  [unwired: 14 in]
      }
      frame "SysConfig: Load APD Info" {
        # "Macro to load APD data\n(load from serial number -> load all data -> get gain limit)"
        n784 = call <vilib>:"Add State(s) to Queue__JKI_lib_State_Machine.vi"("State(s) in Front (\"\")"="APD: LoadFromSerialNoRawData\nAPD: UpdateIndicator\nAPD: GetGainLimits" ("State(s) in Front (\"\")"), "State(s) in (\"\")"=w1801) -> ("States Out"=w1800:string)  [unwired: 13 in]
      }
      frame "SysConfig: Load Digitizer Setting" {
        w1804 = enum16{"Write", "Read"}."Write" ("Operation")
        # "Digitizers in FLImDAQ is not used\nLoad DAQ config\nSave to FGV"
        # "Template Separator\n(You can make a copy of, or modify, this frame)"
        n785 = call <userlib>:"Current VIs Parent Directory__ogtk.vi"() -> ("Parent Directory (+ Relative)"=w1815:path)  [unwired: 5 in]
        n786 = Build Path(base path=w1815, name or relative path="SubVI\\DigitizerConfiguration\\V6_Scope_iRFNew.config") -> (appended path=w1816:path)
        n787 = call "ReadDigitizerConfig(SubVI).vi"("error in (no error)"=w1813, "appended path"=w1816) -> ("error out"=w1808:errorcluster, "FLImDAQ"=w1806:T4)  [unwired: 8 in]
        n788 = call "FLImDAQ_FGV.vi"("error in (no error)"=w1808, "Operation (Read)"=w1804, "Write data"=w1806) -> ("error out"=w1811:errorcluster)  [unwired: 7 in, 1 out]
        n789 = Bundle By Name(cluster=w1802, "FLImDAQ"=w1806) -> (w1803:T22)
        n790 = Unbundle By Name(w1806) -> ("Digitizer 1"=w1809:refnum<k15>, "Digitizer 2"=w1810:refnum<k15>)
        n791 = call "Digitizer1_FGV.vi"("error in (no error)"=w1811, "Operation (Read)"=w1804, "Write data"=w1809) -> ("error out"=w1812:errorcluster)  [unwired: 7 in, 1 out]
        n792 = call "Digitizer2_FGV.vi"("error in (no error)"=w1812, "Operation (Read)"=w1804, "Write data"=w1810) -> ("error out"=w1807:errorcluster)  [unwired: 7 in, 1 out]
        n793 = call <vilib>:"Add State(s) to Queue__JKI_lib_State_Machine.vi"("State(s) in (\"\")"=w1818) -> ("States Out"=w1817:string)  [unwired: 14 in]
      }
      frame "SysConfig: Load Digitizer Setting Gain" {
        w1821 = enum16{"Write", "Read"}."Write" ("Operation")
        # "Digitizers in FLImDAQ is not used\nLoad DAQ config\nSave to FGV"
        # "Template Separator\n(You can make a copy of, or modify, this frame)"
        n794 = call <userlib>:"Current VIs Parent Directory__ogtk.vi"() -> ("Parent Directory (+ Relative)"=w1832:path)  [unwired: 5 in]
        n795 = Build Path(base path=w1832, name or relative path="SubVI\\DigitizerConfiguration\\V6_Scope_Gain.config") -> (appended path=w1833:path)
        n796 = call "ReadDigitizerConfig(SubVI).vi"("error in (no error)"=w1830, "appended path"=w1833) -> ("error out"=w1825:errorcluster, "FLImDAQ"=w1823:T4)  [unwired: 8 in]
        n797 = call "FLImDAQ_FGV.vi"("error in (no error)"=w1825, "Operation (Read)"=w1821, "Write data"=w1823) -> ("error out"=w1828:errorcluster)  [unwired: 7 in, 1 out]
        n798 = Bundle By Name(cluster=w1819, "FLImDAQ"=w1823) -> (w1820:T22)
        n799 = Unbundle By Name(w1823) -> ("Digitizer 1"=w1826:refnum<k15>, "Digitizer 2"=w1827:refnum<k15>)
        n800 = call "Digitizer1_FGV.vi"("error in (no error)"=w1828, "Operation (Read)"=w1821, "Write data"=w1826) -> ("error out"=w1829:errorcluster)  [unwired: 7 in, 1 out]
        n801 = call "Digitizer2_FGV.vi"("error in (no error)"=w1829, "Operation (Read)"=w1821, "Write data"=w1827) -> ("error out"=w1824:errorcluster)  [unwired: 7 in, 1 out]
        n802 = call <vilib>:"Add State(s) to Queue__JKI_lib_State_Machine.vi"("State(s) in (\"\")"=w1835) -> ("States Out"=w1834:string)  [unwired: 14 in]
      }
      frame "SysConfig: Load LJ Pinout" {
        # "Template Separator\n(You can make a copy of, or modify, this frame)"
        n803 = call <userlib>:"Current VIs Parent Directory__ogtk.vi"() -> ("Parent Directory (+ Relative)"=w1849:path)  [unwired: 5 in]
        n804 = Build Path(base path=w1849, name or relative path="SubVI\\LabJack\\LJ_pin_setting.config") -> (appended path=w1847:path)
        n805 = call "ReadLabjackConfig(SubVI).vi"("error in (no error)"=w1845, "appended path"=w1847) -> ("error out"=w1846:errorcluster, "Utility"=w1844:T3)  [unwired: 8 in]
        n806 = Unbundle By Name(w1844) -> ("Ch1 Bias"=w1843:string, "Ch2 Bias"=w1842:string, "Ch3 Bias"=w1841:string, "Red LED"=w1839:string, "Green LED"=w1838:string)
        n807 = global write "GlobalVariables.vi" "LED Green pin"(w1838) -> ()
        n808 = global write "GlobalVariables.vi" "LED Red pin"(w1839) -> ()
        n809 = global write "GlobalVariables.vi" "Ch1 LJ pin"(w1843) -> ()
        n810 = global write "GlobalVariables.vi" "Ch2 LJ pin"(w1842) -> ()
        n811 = global write "GlobalVariables.vi" "Ch3 LJ pin"(w1841) -> ()
        n812 = Bundle By Name(cluster=w1836, "LJ Pinout"=w1844) -> (w1837:T22)
        n813 = call <vilib>:"Add State(s) to Queue__JKI_lib_State_Machine.vi"("State(s) in (\"\")"=w1851) -> ("States Out"=w1850:string)  [unwired: 14 in]
      }
      frame "SysConfig: Load 355 PWM" {
        # "Template Separator\n(You can make a copy of, or modify, this frame)"
        n814 = call <userlib>:"Current VIs Parent Directory__ogtk.vi"() -> ("Parent Directory (+ Relative)"=w1869:path)  [unwired: 5 in]
        n815 = Build Path(base path=w1869, name or relative path="SubVI\\LabJack\\PWM_setting_355.config") -> (appended path=w1867:path)
        n816 = call "ReadPWMConfig(SubVI).vi"("error in (no error)"=w1865, "appended path"=w1867) -> ("error out"=w1866:errorcluster, "PWM Setting"=w1864:T31)  [unwired: 8 in]
        n817 = Unbundle By Name(w1864) -> ("DIO_EF_CLOCK1_DIVISOR"=w1861:i16, "DIO_EF_CLOCK1_ROLL_VALUE"=w1860:i32)
        n818 = Multiply(x=w1861, y=w1860) -> (x*y=w1862:i32)
        n819 = Bundle By Name(cluster=w1852, "355 PWM setting"=w1864) -> (w1853:T22)
        n820 = Divide(x=80000000.0, y=w1862) -> (x/y=w1854:dbl)
        n821 = Number To Decimal String(number=w1854) -> (decimal integer string=w1859:string)  [unwired: 1 in]
        n822 = Concatenate Strings("355nm " ("string"), w1859, "Hz" ("string")) -> (w1857:string)
        n823 = local write "Laser Rep Rate"(w1854) -> ()
        n824 = property on="355nm Laser toggle" class="Bool (strict)"("Caption.Text"=w1857) -> ()  [unwired: 2 in, 2 out]
        n825 = call <vilib>:"Add State(s) to Queue__JKI_lib_State_Machine.vi"("State(s) in (\"\")"=w1871) -> ("States Out"=w1870:string)  [unwired: 14 in]
      }
      frame "SysConfig: Load AB PWM" {
        # "Load AB PWM setting\n(load setting, update AB toggle text)"
        n826 = call <userlib>:"Current VIs Parent Directory__ogtk.vi"() -> ("Parent Directory (+ Relative)"=w1894:path)  [unwired: 5 in]
        n827 = Build Path(base path=w1894, name or relative path="SubVI\\LabJack\\PWM_setting_AB.config") -> (appended path=w1892:path)
        n828 = call "ReadPWMConfig(SubVI).vi"("error in (no error)"=w1890, "appended path"=w1892) -> ("error out"=w1891:errorcluster, "PWM Setting"=w1889:T31)  [unwired: 8 in]
        n829 = Unbundle By Name(w1889) -> ("DIO_EF_CLOCK1_DIVISOR"=w1886:i16, "DIO_EF_CLOCK1_ROLL_VALUE"=w1875:i32, "DIO#_EF_CONFIG_A"=w1876:i32)
        n830 = Divide(x=w1876, y=w1875) -> (x/y=w1874:dbl)
        n831 = Multiply(x=w1886, y=w1875) -> (x*y=w1887:i32)
        n832 = Multiply(x=w1874, y=100.0) -> (x*y=w1872:dbl)
        n833 = Bundle By Name(cluster=w1877, "AB PWM setting"=w1889) -> (w1878:T22)
        n834 = Divide(x=80000000.0, y=w1887) -> (x/y=w1879:dbl)
        n835 = Number To Decimal String(number=w1879, width (-)=i16 2) -> (decimal integer string=w1885:string)
        n836 = local write "Duty Cycle (%)"(w1872) -> ()
        n837 = local write "AB Rep Rate"(w1879) -> ()
        n838 = Concatenate Strings("445nm " ("string"), w1885, "Hz " ("string")) -> (w1883:string)
        n839 = property on="Aiming beam toggle" class="Bool (strict)"("Caption.Text"=w1883) -> ()  [unwired: 2 in, 2 out]
        n840 = call <vilib>:"Add State(s) to Queue__JKI_lib_State_Machine.vi"("State(s) in (\"\")"=w1896) -> ("States Out"=w1895:string)  [unwired: 14 in]
      }
      frame "SysConfig: Load AB setting" {
        # "Template Separator\n(You can make a copy of, or modify, this frame)"
        n841 = call "readAimingBeamSetting.vi"("error in (no error)"=w1898) -> ("error out"=w1897:errorcluster, "Aiming Beam Setting"=w1899:T32)  [unwired: 9 in]
        n842 = Bundle By Name(cluster=w1900, "AB Cluster"=w1899) -> (w1901:T22)
        n843 = call <vilib>:"Add State(s) to Queue__JKI_lib_State_Machine.vi"("State(s) in (\"\")"=w1904) -> ("States Out"=w1903:string)  [unwired: 14 in]
      }
      frame "---------- SystemStatus ----------" {
        # "Template Separator\n(You can make a copy of, or modify, this frame)"
        n844 = call <vilib>:"Add State(s) to Queue__JKI_lib_State_Machine.vi"("State(s) in (\"\")"=w1909) -> ("States Out"=w1908:string)  [unwired: 14 in]
      }
      frame "SystemStatus: SlowSysStatusMacro" {
        # "store system check time"
        # "Template Separator\n(You can make a copy of, or modify, this frame)"
        n845 = Tick Count (ms)() -> (millisecond timer value=w1912:u32)
        n846 = Bundle By Name(cluster=w1910, "SlowTimer"=w1912) -> (w1911:T22)
        n847 = call <vilib>:"Add State(s) to Queue__JKI_lib_State_Machine.vi"("State(s) in Front (\"\")"="/*Digitizer: checkTemp" ("State(s) in Front (\"\")"), "State(s) in (\"\")"=w1917) -> ("States Out"=w1916:string)  [unwired: 13 in]
      }
      frame "SystemStatus: FastSysStatusMacro" {
        # "store system check time"
        # "Template Separator\n(You can make a copy of, or modify, this frame)"
        n848 = Tick Count (ms)() -> (millisecond timer value=w1920:u32)
        n849 = Bundle By Name(cluster=w1918, "FastTimer"=w1920) -> (w1919:T22)
        n850 = call <vilib>:"Add State(s) to Queue__JKI_lib_State_Machine.vi"("State(s) in Front (\"\")"="355 Laser: CheckPWMStatus\n/*AimingBeam: GetPWMStatus" ("State(s) in Front (\"\")"), "State(s) in (\"\")"=w1925) -> ("States Out"=w1924:string)  [unwired: 13 in]
      }
      frame "---------- UI ----------" {
        # "Do not put any code in this frame.\n(It is a separator no-op. You can make a copy of this frame to create a new UI frame)"
        n851 = call <vilib>:"Add State(s) to Queue__JKI_lib_State_Machine.vi"("State(s) in (\"\")"=w1930) -> ("States Out"=w1929:string)  [unwired: 14 in]
      }
      frame "UI: InitIRFDataTable" {
        # "Initial iRF table setup\n(Setup the table for iRF measurement, set the active cell to 1st roll)"
        n852 = while {
          tunnel: [w1955] -> w1934 mode=indexing
          shift-right: [w1955] -> _
          shift-left: 0.03 -> [w1961]
          stop <- w1956 continue-if-true
          # "Generate Gain less than 3"
          n853 = Greater Or Equal?(x=w1961, y=3.0) -> (x >= y?=w1964:bool)
          n854 = Select(t=0.02, s=w1964, f=0.02) -> (s? t:f=w1960:dbl)
          n855 = Add(x=w1960, y=w1961) -> (x+y=w1959:dbl)
          n856 = In Range and Coerce(upper limit=4.6, x=w1959, lower limit=0.05) -> (coerced(x)=w1955:dbl, In Range?=w1956:bool)
        }
        "iRFCtrlV" <- w1934
        n857 = for {
          tunnel: w1934 -> [w1954] mode=indexing
          tunnel: [w1950] -> w1933 mode=indexing
          tunnel: T19 {"Row"=0, "Column"=0} ("Active Cell:Active Cell") -> [w1945]
          i -> [w1944]
          n858 = Bundle By Name(cluster=w1945, "Row"=w1944, "Column"=0) -> (w1948:T19)
          n859 = Number To Fractional String(number=w1954, precision (6)=i16 2) -> (F-format string=w1952:string)  [unwired: 2 in]
          n860 = Equal To 0?(x=w1944) -> (x = 0?=w1943:bool)
          n861 = Select(t=u32 16773632 ("Active Cell:Cell Background Color"), s=w1943, f=u32 16448250 ("Active Cell:Cell Background Color")) -> (s? t:f=w1940:u32)
          n862 = property on="iRFDataTable" class="Tbl (strict)"("Active Cell"=w1948, "Cell BG Color"=w1940) -> ()  [unwired: 2 in, 2 out]
          n863 = Build Array(w1952, "No" ("element")) -> (w1950:string[])
          n864 = Bundle By Name(cluster=w1945, "Row"=w1944, "Column"=1) -> (w1946:T19)
          n865 = property on="iRFDataTable" class="Tbl (strict)"("Active Cell"=w1946, "Cell BG Color"=w1940) -> ()  [unwired: 2 in, 2 out]
        }
        "iRFDataTable" <- w1933
        n866 = call <vilib>:"Add State(s) to Queue__JKI_lib_State_Machine.vi"("State(s) in (\"\")"=w1939) -> ("States Out"=w1938:string)  [unwired: 14 in]
      }
      frame "UI: UpdateIRFDataTable" {
        w1968 = i32[] [0, 1]
        w1967 = T19 {"Row"=0, "Column"=0} ("Active Cell:Active Cell")
        # "Update iRF data table.\n(Change Status to yes, update table color)"
        n867 = local read "iRFDataTable"() -> (w1974:string[][])
        n868 = Unbundle By Name(w1973) -> ("iRFIdx"=w1966:i32)
        n869 = Decrement(x=w1966) -> (x-1=w1969:i32)
        n870 = Replace Array Subset(array=w1974, new element="Yes" ("new element/subarray"), index (row)=w1969, index (col)=1 ("disabled index (col)")) -> (w1970:string[][])
        n871 = for {
          tunnel: w1968 -> [w1986] mode=indexing
          tunnel: w1967 -> [w1988]
          tunnel: w1969 -> [w1987]
          # "Update cell BG color"
          n872 = Bundle By Name(cluster=w1988, "Row"=w1987, "Column"=w1986) -> (w1985:T19)
          n873 = property on="iRFDataTable" class="Tbl (strict)"("Active Cell"=w1985, "Cell BG Color"=u32 6618880 ("Active Cell:Cell Background Color")) -> ()  [unwired: 2 in, 2 out]
        }
        n874 = for {
          tunnel: w1968 -> [w1981] mode=indexing
          tunnel: w1967 -> [w1983]
          tunnel: w1966 -> [w1982]
          n875 = Bundle By Name(cluster=w1983, "Row"=w1982, "Column"=w1981) -> (w1980:T19)
          n876 = property on="iRFDataTable" class="Tbl (strict)"("Active Cell"=w1980, "Cell BG Color"=u32 16773632 ("Active Cell:Cell Background Color")) -> ()  [unwired: 2 in, 2 out]
        }
        n877 = local write "iRFDataTable"(w1970) -> ()
        n878 = call <vilib>:"Add State(s) to Queue__JKI_lib_State_Machine.vi"("State(s) in (\"\")"=w1978) -> ("States Out"=w1977:string)  [unwired: 14 in]
      }
      frame "UI: UpdateGainDataIndicators" {
        # "Update indicator for Gain data.\n(Update Arrays and tables)"
        n879 = Unbundle By Name(w1999) -> ("GainDataTemp.CtrlV"=w1990:dbl, "GainDataTemp.AUC"=w1989:dbl, "GainDataTemp.AUC Std"=w1998:dbl, "GainDataTemp.IntFactor"=w1997:dbl, "GainDataTemp.IntCorrAUC"=w1996:dbl)
        n880 = local read "Int Corr AUC"() -> (w2002:dbl[])
        n881 = Build Array(w1990, w1989, w1998, w1997, w1996) -> (w1995:dbl[])
        n882 = local read "Intensity Factor"() -> (w2005:dbl[])
        n883 = for {
          tunnel: w1995 -> [w2021] mode=indexing
          tunnel: [w2019] -> w1993 mode=indexing
          n884 = Number To Fractional String(number=w2021, precision (6)=i16 3) -> (F-format string=w2019:string)  [unwired: 2 in]
        }
        n885 = local read "AUC Std"() -> (w2008:dbl[])
        n886 = local read "AUC"() -> (w2014:dbl[])
        n887 = local read "Ctrl V"() -> (w2011:dbl[])
        n888 = Insert Into Array(array=w2014, index=0, new element=w1989) -> (→"AUC":dbl[])
        n889 = Insert Into Array(array=w2011, index=0, new element=w1990) -> (→"Ctrl V":dbl[])
        n890 = Insert Into Array(array=w2005, index=0, new element=w1997) -> (→"Intensity Factor":dbl[])
        n891 = Insert Into Array(array=w2002, index=0, new element=w1996) -> (→"Int Corr AUC":dbl[])
        n892 = Insert Into Array(array=w2008, index=0, new element=w1998) -> (→"AUC Std":dbl[])
        n893 = local read "GainDataTable"() -> (w1991:string[][])
        n894 = Insert Into Array(array=w1991, index (row)=0, new element=w1993) -> (→"GainDataTable":string[][])  [unwired: 1 in]
        n895 = call <vilib>:"Add State(s) to Queue__JKI_lib_State_Machine.vi"("State(s) in (\"\")"=w2018) -> ("States Out"=w2017:string)  [unwired: 14 in]
      }
      frame "UI: ShowDialog" {
        # "Show dialog ask user to adjust signal level\n(If OK aquire data, if abort stop auqisition)"
        n896 = local read "Task"() -> (w2022:enum32{"iRFAndGain", "Alignment"})
        n897 = case shown="\"Alignment\"" w2022 {
          tunnel: ["Please adjsut max signal level to around 1V." ("message") "Click OK to confirm data!" ("message")] -> w2028
          frame "iRFAndGain", Default {
          }
          frame "Alignment" {
          }
        }
        n898 = Two Button Dialog(message=w2028, 1:"Abort" ("F button name (\"Cancel\")"), 2:"OK" ("T button name (\"OK\")")) -> (T button?=w2025:bool)
        n899 = case shown="False" w2025 {
          tunnel: ["Macro: StopRun\nQueue: FlashDataAllQueue" ("State(s) in Front (\"\")") w2036] -> w2024
          tunnel: w2023 -> [_ w2036]
          frame False {
            # "Stop if abort"
          }
          frame True {
            # "Continue if OK"
          }
        }
        n900 = call <vilib>:"Add State(s) to Queue__JKI_lib_State_Machine.vi"("State(s) in Front (\"\")"=w2024) -> ("States Out"=w2032:string)  [unwired: 14 in]
      }
      frame "UI: WFAutoScale" {
        # "Set graph auto scale.\n(UI: WFAutoScale >> T/F)"
        n901 = Equal?(x=w2037, y="F") -> (x = y?=w2038:bool)
        n902 = Equal?(x=w2037, y="T") -> (x = y?=w2040:bool)
        n903 = case shown="True" w2040 {
          frame False {
          }
          frame True {
            n904 = property on="Waveform (no average)" class="WFGraph (strict)"("YScale.ScaleFit"=u8 2 ("Y Scale.Scale Fit")) -> ()  [unwired: 2 in, 2 out]
          }
        }
        n905 = case shown="True" w2038 {
          frame False {
          }
          frame True {
            n906 = property on="Waveform (no average)" class="WFGraph (strict)"("YScale.ScaleFit"=u8 0 ("Y Scale.Scale Fit")) -> (error out=w2048:errorcluster)  [unwired: 2 in, 1 out]
            n907 = property on="Waveform (no average)" class="WFGraph (strict)"(error in=w2048, "YScale.Maximum"=2.0 ("Y Scale.Range:Maximum")) -> (error out=w2047:errorcluster)  [unwired: 1 in, 1 out]
            n908 = property on="Waveform (no average)" class="WFGraph (strict)"(error in=w2047, "YScale.Minimum"=0.0 ("Y Scale.Range:Maximum")) -> ()  [unwired: 1 in, 2 out]
          }
        }
        n909 = call <vilib>:"Add State(s) to Queue__JKI_lib_State_Machine.vi"("State(s) in (\"\")"=w2046) -> ("States Out"=w2045:string)  [unwired: 14 in]
      }
      frame "UI: Initialize" {
        w2054 = T11."Disabled and Grayed Out" ("Disabled")
        # "Disable all button on startup"
        # "Initialize the User Interface, here.\n(this is called automatically, by the Macro: Init)"
        n910 = property on="Ctrl V" class="DigNum (strict)"("DisabledEnum"=w2054) -> ()  [unwired: 2 in, 2 out]
        n911 = property on="StopButton" class="Bool"("DisabledEnum"=w2054) -> ()  [unwired: 2 in, 2 out]
        n912 = property on="Sys Reconfig" class="Bool"("DisabledEnum"=w2054) -> ()  [unwired: 2 in, 2 out]
        n913 = property on="StartButton" class="Bool"("DisabledEnum"=w2054) -> ()  [unwired: 2 in, 2 out]
        n914 = property on="355nm Laser toggle" class="Bool (strict)"("DisabledEnum"=w2054) -> ()  [unwired: 2 in, 2 out]
        n915 = property on="Aiming beam toggle" class="Bool (strict)"("DisabledEnum"=w2054) -> ()  [unwired: 2 in, 2 out]
        n916 = property on="Ctrl V" class="DigNum (strict)"("Data Range"=T20 {"Minimum"=0.0, "Maximum"=5.5, "Increment"=0.1} ("Data Entry Limits")) -> ()  [unwired: 2 in, 2 out]
        n917 = call <vilib>:"Add State(s) to Queue__JKI_lib_State_Machine.vi"("State(s) in (\"\")"=w2059) -> ("States Out"=w2058:string)  [unwired: 14 in]
      }
      frame "UI: showDisclaimer" {
        # "Show disclamer window.\n(It is a separator no-op. You can make a copy of this frame to create a new UI frame)"
        n918 = call <vilib>:"Application Directory.vi"() -> ("Application Directory"=w2072:path)
        n919 = Build Path(base path=w2072, name or relative path="Disclamer.png") -> (appended path=w2070:path)
        n920 = property on="Disclamer" class="Pict"() -> ("Draw Area Size"=w2068:T33)  [unwired: 2 in, 2 out]
        n921 = call <vilib>:"Read PNG File.vi"("path to PNG file"=w2070) -> ("image data"=w2067:T34)  [unwired: 8 in, 2 out]
        n922 = disable-structure "Diagram Disable Structure" shown="Disabled" {
          frame Disabled {
            n923 = flat-sequence {
              frame #0 {
                n924 = call "disclaimer.vi"() -> ()  [unwired: 12 in]
              }
              frame #1 {
                n925 = Wait (ms)(milliseconds to wait=u32 250) -> ()  [unwired: 1 out]
              }
              frame #2 {
                n926 = call "SoftwareNote.vi"() -> ()  [unwired: 12 in]
              }
            }
          }
          frame Enabled {
          }
        }
        n927 = Unbundle By Name(w2067) -> ("Rectangle.right"=w2065:i16, "Rectangle.bottom"=w2063:i16)
        n928 = Unbundle By Name(w2068) -> ("Width"=w2066:u32, "Height"=w2064:u32)
        n929 = call <vilib>:"Draw Flattened Pixmap.vi"("image data"=w2067) -> ("new picture"=→"Disclamer":picture)  [unwired: 8 in]
        n930 = Divide(x=w2066, y=w2065) -> (x/y=w2062:dbl)
        n931 = Divide(x=w2064, y=w2063) -> (x/y=w2061:dbl)
        n932 = Max & Min(x=w2062, y=w2061) -> (min(x,y)=w2060:dbl)  [unwired: 1 out]
        n933 = property on="Disclamer" class="Pict"("ZoomFactor"=w2060) -> ()  [unwired: 2 in, 2 out]
        n934 = call <vilib>:"Add State(s) to Queue__JKI_lib_State_Machine.vi"("State(s) in (\"\")"=w2077) -> ("States Out"=w2076:string)  [unwired: 14 in]
      }
      frame "UI: SetButtonText" {
        # "Set button text of 355nm laser and aiming beam."
        n935 = call <vilib>:"Add State(s) to Queue__JKI_lib_State_Machine.vi"("State(s) in (\"\")"=w2083) -> ("States Out"=w2082:string)  [unwired: 14 in]
      }
      frame "UI: DuringAquisition" {
        w2084 = T11."Enabled" ("Disabled")
        w2089 = T11."Disabled and Grayed Out" ("Disabled")
        # "Do not put any code in this frame.\n(It is a separator no-op. You can make a copy of this frame to create a new UI frame)"
        n936 = property on="StopButton" class="Bool"("DisabledEnum"=w2084) -> ()  [unwired: 2 in, 2 out]
        n937 = property on="iRFSigInRange" class="Bool (strict)"("DisabledEnum"=w2084) -> ()  [unwired: 2 in, 2 out]
        n938 = property on="AcquireGain" class="Bool"("DisabledEnum"=w2084) -> ()  [unwired: 2 in, 2 out]
        n939 = property on="GainSigInRange" class="Bool (strict)"("DisabledEnum"=w2084) -> ()  [unwired: 2 in, 2 out]
        n940 = property on="AcquireIRF" class="Bool"("DisabledEnum"=w2084) -> ()  [unwired: 2 in, 2 out]
        n941 = Bundle By Name(cluster=w2087, "SysRunning?"=TRUE) -> (w2088:T22)
        n942 = property on="StartButton" class="Bool"("DisabledEnum"=w2089) -> ()  [unwired: 2 in, 2 out]
        n943 = property on="Sys Reconfig" class="Bool"("DisabledEnum"=w2089) -> ()  [unwired: 2 in, 2 out]
        n944 = property on="355nm Laser toggle" class="Bool (strict)"("DisabledEnum"=w2089) -> ()  [unwired: 2 in, 2 out]
        n945 = property on="Aiming beam toggle" class="Bool (strict)"("DisabledEnum"=w2089) -> ()  [unwired: 2 in, 2 out]
        n946 = local write "GainInstSting"("Please set control voltage and make sure data is in range.\nClick 'Acquire' button to record data." ("GainInstSting")) -> ()
        n947 = property on="Quit" class="Bool"("DisabledEnum"=w2089) -> ()  [unwired: 2 in, 2 out]
        n948 = local write "iRFInstSting"("1. Click 'Set CtrlV' to set APD bias voltage\n2. Click 'Acquire' button to record data." ("iRFInstSting")) -> ()
        n949 = property on="Laser Rep Rate" class="DigNum (strict)"("DisabledEnum"=w2089) -> ()  [unwired: 2 in, 2 out]
        n950 = property on="Channel" class="RadioBtnsControl (strict)"("DisabledEnum"=w2089) -> ()  [unwired: 2 in, 2 out]
        n951 = property on="Task" class="RadioBtnsControl (strict)"("DisabledEnum"=w2089) -> ()  [unwired: 2 in, 2 out]
        n952 = call <vilib>:"Add State(s) to Queue__JKI_lib_State_Machine.vi"("State(s) in (\"\")"=w2094) -> ("States Out"=w2093:string)  [unwired: 14 in]
      }
      frame "UI: ReadyForAquisition" {
        w2095 = T11."Disabled and Grayed Out" ("Disabled")
        w2101 = T11."Enabled" ("Disabled")
        # "Do not put any code in this frame.\n(It is a separator no-op. You can make a copy of this frame to create a new UI frame)"
        n953 = local read "Channel"() -> (w2097:enum32{"Ch1", "Ch2", "Ch3"})
        n954 = property on="StopButton" class="Bool"("DisabledEnum"=w2095) -> ()  [unwired: 2 in, 2 out]
        n955 = property on="AcquireGain" class="Bool"("DisabledEnum"=w2095) -> ()  [unwired: 2 in, 2 out]
        n956 = property on="iRFSigInRange" class="Bool (strict)"("DisabledEnum"=w2095) -> ()  [unwired: 2 in, 2 out]
        n957 = property on="GainSigInRange" class="Bool (strict)"("DisabledEnum"=w2095) -> ()  [unwired: 2 in, 2 out]
        n958 = property on="AcquireIRF" class="Bool"("DisabledEnum"=w2095) -> ()  [unwired: 2 in, 2 out]
        n959 = Bundle By Name(cluster=w2099, "SysRunning?"=FALSE) -> (w2100:T22)
        n960 = case shown="\"Ch2\"" w2097 {
          tunnel: ["To aquire gain data:\n1. Place blue Chroma slide as close as possible to the fiber port! \n2. Start data aquisition." ("GainInstSting") "To aquire gain data:\n1. Place blue Chroma slide as close as possible to the fiber port! \n2. Start data aquisition." ("GainInstSting") "To aquire gain data:\n1. Place green Chroma slide as close as possible to the fiber port! \n2. Remove Channel 3 bandpass filter!\n3. Start data aquisition." ("GainInstSting")] -> w2098
          tunnel: ["To aquire gain data:\n1. Install Thorlabs fiber stop! \n2. Start data aquisition." ("GainInstSting") "To aquire gain data:\n1. Install Thorlabs fiber stop! \n2. Start data aquisition." ("GainInstSting") "To aquire gain data:\n1. Install fiber probe!\n2. Place DASPI solution as close as possible to fiber probe.\n3. Remove Channel 3 bandpass filter. \n4. Start data aquisition." ("GainInstSting")] -> w2096
          frame "Ch1", Default {
          }
          frame "Ch2" {
          }
          frame "Ch3" {
          }
        }
        "GainInstSting" <- w2098
        "iRFInstSting" <- w2096
        n961 = property on="StartButton" class="Bool"("DisabledEnum"=w2101) -> ()  [unwired: 2 in, 2 out]
        n962 = property on="Sys Reconfig" class="Bool"("DisabledEnum"=w2101) -> ()  [unwired: 2 in, 2 out]
        n963 = property on="355nm Laser toggle" class="Bool (strict)"("DisabledEnum"=w2101) -> ()  [unwired: 2 in, 2 out]
        n964 = property on="Aiming beam toggle" class="Bool (strict)"("DisabledEnum"=w2101) -> ()  [unwired: 2 in, 2 out]
        n965 = property on="Quit" class="Bool"("DisabledEnum"=w2101) -> ()  [unwired: 2 in, 2 out]
        n966 = property on="Channel" class="RadioBtnsControl (strict)"("DisabledEnum"=w2101) -> ()  [unwired: 2 in, 2 out]
        n967 = property on="Laser Rep Rate" class="DigNum (strict)"("DisabledEnum"=w2101) -> ()  [unwired: 2 in, 2 out]
        n968 = property on="Task" class="RadioBtnsControl (strict)"("DisabledEnum"=w2101) -> ()  [unwired: 2 in, 2 out]
        n969 = call <vilib>:"Add State(s) to Queue__JKI_lib_State_Machine.vi"("State(s) in Front (\"\")"="LED: Green" ("State(s) in Front (\"\")"), "State(s) in (\"\")"=w2107) -> ("States Out"=w2106:string)  [unwired: 13 in]
      }
      frame "UI: Update" {
        # "Do not put any code in this frame.\n(It is a separator no-op. You can make a copy of this frame to create a new UI frame)"
        n970 = Unbundle By Name(w2121) -> ("System Status"=→"System Hardware Connection Status":T1, "IDs.RunID"=→"Run #":i8, "FLImDAQ"=→"FLImDAQ":T27, "SysRunning?"=→"System Status:":bool, "LJ Pinout"=→"LJ Pinout":T3, "IDs.BG ID"=→"BG #":i8, "IDs.Cali ID"=→"Calibration #":i8)
        n971 = call <vilib>:"Add State(s) to Queue__JKI_lib_State_Machine.vi"("State(s) in (\"\")"=w2125) -> ("States Out"=w2124:string)  [unwired: 14 in]
      }
      frame "UI: Cursor Set" {
        # "Argument"
        # "Set and Unset Cursor Busy.\n(Usage: \"UI: Cursor Set >> Busy|Idle\")"
        n972 = case shown="\"Idle\", Default" w2127 {
          tunnel: w2129 -> [w2134 w2136]
          tunnel: [w2133 w2135] -> w2128
          frame "Idle", Default {
            n973 = call <vilib>:"Unset Busy.vi"("error in (no error)"=w2134) -> ("error out"=w2133:errorcluster)  [unwired: 10 in]
          }
          frame "Busy" {
            n974 = call <vilib>:"Set Busy.vi"("error in (no error)"=w2136) -> ("error out"=w2135:errorcluster)  [unwired: 9 in, 1 out]
          }
        }
        n975 = call <vilib>:"Add State(s) to Queue__JKI_lib_State_Machine.vi"("State(s) in (\"\")"=w2132) -> ("States Out"=w2131:string)  [unwired: 14 in]
      }
      frame "UI: Front Panel State" {
        # "Argument"
        # "Set Front Panel Open or Closed\n(Usage: \"UI: Front Panel State >> Open|Close\")"
        n976 = Unbundle By Name(w2137) -> ("Core.Current VI Reference"=w2140:refnum<vi>)
        n977 = case shown="\"Open\", \"Standard\", Default" w2139 {
          tunnel: w2142 -> [w2150 w2163 w2174 w2186 w2198]
          tunnel: [w2151 w2164 w2175 w2187 w2199] -> w2141
          tunnel: w2140 -> [_ _ _ _ _]
          frame "Open", "Standard", Default {
            w2145 = T15."Standard" ("State")
            n978 = property on="Property Node" class="VI"(error in=w2150) -> (reference out=w2148:refnum<vi>, error out=w2149:errorcluster, "FP.State"=w2147:T15)  [unwired: 1 in]
            n979 = Not Equal?(x=w2147, y=w2145) -> (x != y?=w2146:bool)
            n980 = case shown="True" w2146 {
              tunnel: [w2155 w2157] -> w2151
              tunnel: w2149 -> [w2154 w2157]
              tunnel: w2148 -> [w2153 _]
              tunnel: w2145 -> [w2152 _]
              frame True {
                n981 = invoke on="Invoke Node" class="VI" method="FP.Open"(reference=w2153, error in=w2154, "Activate"=TRUE, "State"=w2152) -> (error out=w2155:errorcluster)  [unwired: 1 in, 4 out]
              }
              frame False {
              }
            }
          }
          frame "Close", "Closed" {
            n982 = property on="Property Node" class="VI"(error in=w2163) -> (reference out=w2161:refnum<vi>, error out=w2162:errorcluster, "FP.State"=w2159:T15)  [unwired: 1 in]
            n983 = Not Equal?(x=w2159, y=T15."Closed" ("Front Panel Window:State")) -> (x != y?=w2158:bool)
            n984 = case shown="True" w2158 {
              tunnel: [w2165 w2168] -> w2164
              tunnel: w2162 -> [w2165 w2167]
              tunnel: w2161 -> [_ w2166]
              frame False {
              }
              frame True {
                n985 = invoke on="Invoke Node" class="VI" method="FP.Close"(reference=w2166, error in=w2167) -> (error out=w2168:errorcluster)  [unwired: 1 in, 2 out]
              }
            }
          }
          frame "Hidden", "Hide" {
            w2169 = T15."Hidden" ("State")
            n986 = property on="Property Node" class="VI"(error in=w2174) -> (reference out=w2172:refnum<vi>, error out=w2173:errorcluster, "FP.State"=w2171:T15)  [unwired: 1 in]
            n987 = Not Equal?(x=w2171, y=w2169) -> (x != y?=w2170:bool)
            n988 = case shown="True" w2170 {
              tunnel: [w2179 w2180] -> w2175
              tunnel: w2173 -> [w2178 w2180]
              tunnel: w2172 -> [w2177 _]
              tunnel: w2169 -> [w2176 _]
              frame True {
                n989 = invoke on="Invoke Node" class="VI" method="FP.Open"(reference=w2177, error in=w2178, "State"=w2176) -> (error out=w2179:errorcluster)  [unwired: 2 in, 4 out]
              }
              frame False {
              }
            }
          }
          frame "Minimize", "Minimized" {
            w2181 = T15."Minimized" ("State")
            n990 = property on="Property Node" class="VI"(error in=w2186) -> (reference out=w2184:refnum<vi>, error out=w2185:errorcluster, "FP.State"=w2183:T15)  [unwired: 1 in]
            n991 = Not Equal?(x=w2183, y=w2181) -> (x != y?=w2182:bool)
            n992 = case shown="True" w2182 {
              tunnel: [w2191 w2192] -> w2187
              tunnel: w2185 -> [w2190 w2192]
              tunnel: w2184 -> [w2189 _]
              tunnel: w2181 -> [w2188 _]
              frame True {
                n993 = invoke on="Invoke Node" class="VI" method="FP.Open"(reference=w2189, error in=w2190, "State"=w2188) -> (error out=w2191:errorcluster)  [unwired: 2 in, 4 out]
              }
              frame False {
              }
            }
          }
          frame "Maximize", "Maximized" {
            w2193 = T15."Maximized" ("State")
            n994 = property on="Property Node" class="VI"(error in=w2198) -> (reference out=w2196:refnum<vi>, error out=w2197:errorcluster, "FP.State"=w2195:T15)  [unwired: 1 in]
            n995 = Not Equal?(x=w2195, y=w2193) -> (x != y?=w2194:bool)
            n996 = case shown="True" w2194 {
              tunnel: [w2203 w2204] -> w2199
              tunnel: w2197 -> [w2202 w2204]
              tunnel: w2196 -> [w2201 _]
              tunnel: w2193 -> [w2200 _]
              frame True {
                n997 = invoke on="Invoke Node" class="VI" method="FP.Open"(reference=w2201, error in=w2202, "State"=w2200) -> (error out=w2203:errorcluster)  [unwired: 2 in, 4 out]
              }
              frame False {
              }
            }
          }
        }
        n998 = call <vilib>:"Add State(s) to Queue__JKI_lib_State_Machine.vi"("State(s) in (\"\")"=w2144) -> ("States Out"=w2143:string)  [unwired: 14 in]
      }
      frame "---------- 355 Laser ----------" {
        # "Template Separator\n(You can make a copy of, or modify, this frame)"
        n999 = call <vilib>:"Add State(s) to Queue__JKI_lib_State_Machine.vi"("State(s) in (\"\")"=w2209) -> ("States Out"=w2208:string)  [unwired: 14 in]
      }
      frame "355 Laser: Check Dewelling" {
        # "if time laser start time is less than 7.5s before, wait 250ms then check again."
        # "Check laser timer\n(Check laser timer, make sure enough time lapsed after laser enable)"
        n1000 = Unbundle By Name(w2211) -> ("Laser start tic"=w2210:u32)
        n1001 = Tick Count (ms)() -> (millisecond timer value=w2216:u32)
        n1002 = Subtract(x=w2216, y=w2210) -> (x-y=w2215:u32)
        n1003 = Greater?(x=w2215, y=u32 5000) -> (0:w2213:bool)
        n1004 = case shown="False" w2213 {
          tunnel: ["355 Laser: Check Dewelling" ""] -> w2212
          frame False {
            n1005 = Wait (ms)(milliseconds to wait=u32 500) -> ()  [unwired: 1 out]
          }
          frame True {
          }
        }
        n1006 = call <vilib>:"Add State(s) to Queue__JKI_lib_State_Machine.vi"("State(s) in Front (\"\")"=w2212, "State(s) in (\"\")"=w2220) -> ("States Out"=w2219:string)  [unwired: 13 in]
      }
      frame "355 Laser: Laser enable" {
        # "Laser enable/disable\n(Usage: \"LabJack: Laser enable/disable >> 1|0\")"
        n1007 = Unbundle By Name(w2225) -> ("LJ Pinout.Laser Start/Stop"=w2231:string, "System Status.355 Laser"=w2224:bool)
        n1008 = case shown="False" w2224 {
          tunnel: w2227 -> [w2246 w2247]
          tunnel: w2231 -> [w2234 _]
          tunnel: [w2236 w2247] -> w2229
          tunnel: [w2235 u32 0 ("millisecond timer value")] -> w2228
          frame False {
            n1009 = call "LabJack_FGV.vi"("Operation(Read)"=enum16{"Write", "Read"}."Read" ("Operation")) -> ("Read data"=w2242:i32)  [unwired: 9 in, 1 out]
            n1010 = call "LJM_eWriteName.vi"("Handle In"=w2242, "Name"=w2234, "Value"=1.0, "error in"=w2246) -> ("Handle Out"=w2241:i32, "error out"=w2240:errorcluster)  [unwired: 10 in]
            n1011 = call <userlib>:"Wait (ms)__ogtk.vi"("error in (no error)"=w2240, "milliseconds to wait"=u32 250) -> ("error out"=w2239:errorcluster)  [unwired: 8 in, 1 out]
            n1012 = call "LJM_eWriteName.vi"("Handle In"=w2241, "Name"=w2234, "Value"=0.0, "error in"=w2239) -> ("error out"=w2237:errorcluster)  [unwired: 10 in, 1 out]
            n1013 = call <userlib>:"Tick Count (ms)__ogtk.vi"("error in (no error)"=w2237) -> ("error out"=w2236:errorcluster, "millisecond timer value"=w2235:u32)  [unwired: 9 in]
          }
          frame True {
          }
        }
        n1014 = Bundle By Name(cluster=w2225, "Laser start tic"=w2228) -> (w2226:T22)
        n1015 = call <vilib>:"Add State(s) to Queue__JKI_lib_State_Machine.vi"("State(s) in (\"\")"=w2233) -> ("States Out"=w2232:string)  [unwired: 14 in]
      }
      frame "355 Laser: Laser disable" {
        # "Laser enable/disable\n(Usage: \"LabJack: Laser enable/disable >> 1|0\")"
        n1016 = Unbundle By Name(w2250) -> ("LJ Pinout.Laser Start/Stop"=w2255:string, "System Status.355 Laser"=w2249:bool)
        n1017 = case shown="True" w2249 {
          tunnel: w2256 -> [w2259 w2273]
          tunnel: w2255 -> [_ w2261]
          tunnel: [w2259 w2263] -> w2253
          tunnel: [u32 0 ("millisecond timer value") w2262] -> w2252
          frame False {
          }
          frame True {
            n1018 = call "LabJack_FGV.vi"("Operation(Read)"=enum16{"Write", "Read"}."Read" ("Operation")) -> ("Read data"=w2269:i32)  [unwired: 9 in, 1 out]
            n1019 = call "LJM_eWriteName.vi"("Handle In"=w2269, "Name"=w2261, "Value"=1.0, "error in"=w2273) -> ("Handle Out"=w2268:i32, "error out"=w2267:errorcluster)  [unwired: 10 in]
            n1020 = call <userlib>:"Wait (ms)__ogtk.vi"("error in (no error)"=w2267, "milliseconds to wait"=u32 250) -> ("error out"=w2266:errorcluster)  [unwired: 8 in, 1 out]
            n1021 = call "LJM_eWriteName.vi"("Handle In"=w2268, "Name"=w2261, "Value"=0.0, "error in"=w2266) -> ("error out"=w2264:errorcluster)  [unwired: 10 in, 1 out]
            n1022 = call <userlib>:"Tick Count (ms)__ogtk.vi"("error in (no error)"=w2264) -> ("error out"=w2263:errorcluster, "millisecond timer value"=w2262:u32)  [unwired: 9 in]
          }
        }
        n1023 = Bundle By Name(cluster=w2250, "Laser start tic"=w2252) -> (w2251:T22)
        n1024 = call <vilib>:"Add State(s) to Queue__JKI_lib_State_Machine.vi"("State(s) in (\"\")"=w2258) -> ("States Out"=w2257:string)  [unwired: 14 in]
      }
      frame "355 Laser: Dewelling" {
        # "Wait some time (ms)\n(355 Laser: Dewelling >> #)"
        n1025 = Fract/Exp String To Number(string=w2277, default (0 dbl)=0) -> (number=w2275:i32)  [unwired: 2 in, 1 out]
        n1026 = Wait (ms)(milliseconds to wait=w2275) -> ()  [unwired: 1 out]
        n1027 = call <vilib>:"Add State(s) to Queue__JKI_lib_State_Machine.vi"("State(s) in (\"\")"=w2281) -> ("States Out"=w2280:string)  [unwired: 14 in]
      }
      frame "355 Laser: Init" {
        # "Initilize 355nm laser\n(Start laser, enable interlock)"
        n1028 = call <vilib>:"Add State(s) to Queue__JKI_lib_State_Machine.vi"("State(s) in Front (\"\")"="355 Laser: CheckControllerStatus", "State(s) in (\"\")"=w2287) -> ("States Out"=w2286:string)  [unwired: 13 in]
      }
      frame "355 Laser: Close" {
        # "Template Separator\n(You can make a copy of, or modify, this frame)"
        n1029 = call <vilib>:"Add State(s) to Queue__JKI_lib_State_Machine.vi"("State(s) in Front (\"\")"="355 Laser: CheckControllerStatus\n355 Laser: Laser disable\n355 Laser: Dewelling >>1000", "State(s) in (\"\")"=w2293) -> ("States Out"=w2292:string)  [unwired: 13 in]
      }
      frame "355 Laser: CheckControllerStatus" {
        # "if average < 1, laser on\nif average > 9, laser off\nif 1<average<9, interlock open, blink indicator"
        # "take 10 measuremt and look at average"
        # "Check 355 laser controller status\nBy probing Emisison Lamp negative terminal voltage"
        n1030 = Unbundle By Name(w2294) -> ("LJ Pinout.Laser Ready"=w2304:string)
        n1031 = call "LabJack_FGV.vi"("Operation(Read)"=enum16{"Write", "Read"}."Read" ("Operation")) -> ("Read data"=w2305:i32)  [unwired: 9 in, 1 out]
        n1032 = for {
          N: 10 -> [_]
          tunnel: w2305 -> [w2339]
          tunnel: w2304 -> [w2334]
          shift-right: [w2338] -> w2298
          shift-left: w2303 -> [w2337]
          tunnel: [w2335] -> w2296 mode=indexing
          n1033 = call "LJM_eReadName.vi"("Handle In"=w2339, "Name"=w2334, "error in"=w2337) -> ("Value"=w2335:dbl, "error out"=w2338:errorcluster)  [unwired: 10 in, 1 out]
          n1034 = Wait (ms)(milliseconds to wait=u32 50) -> ()  [unwired: 1 out]
        }
        n1035 = case shown="No Error" w2298 {
          selector: w2298 -> [w2313 w2332]
          tunnel: [w2315 FALSE] -> w2300
          tunnel: [w2314 w2332] -> w2299
          tunnel: [w2309 nan] -> w2297
          tunnel: w2296 -> [w2311 _]
          frame No Error {
            n1036 = call-poly <vilib>:"Mean.vi"("X"=w2311) -> ("mean"=w2309:dbl)  [unwired: 1 out]
            n1037 = Less?(x=w2309, y=9.3) -> (x < y?=w2310:bool)
            n1038 = case shown="False" w2310 {
              tunnel: [w2318 TRUE] -> w2315
              tunnel: w2309 -> [w2321 _]
              tunnel: w2313 -> [w2317 w2328]
              tunnel: [w2316 w2328] -> w2314
              frame False {
                n1039 = Greater?(x=w2321, y=10.0) -> (0:w2319:bool)
                n1040 = case shown="True" w2319 {
                  tunnel: [FALSE FALSE] -> w2318
                  tunnel: w2317 -> [_ w2325]
                  tunnel: [errorcluster {"status"=TRUE, "code"=5002, "source"="355 Laser"} ("error out") w2325] -> w2316
                  frame False {
                    n1041 = property on="355 Laser" class="Bool (strict)"("Blinking"=FALSE) -> ()  [unwired: 2 in, 2 out]
                  }
                  frame True {
                    n1042 = property on="355 Laser" class="Bool (strict)"("Blinking"=FALSE) -> ()  [unwired: 2 in, 2 out]
                  }
                }
              }
              frame True {
                n1043 = property on="355 Laser" class="Bool (strict)"("Blinking"=FALSE) -> ()  [unwired: 2 in, 2 out]
              }
            }
          }
          frame Error {
          }
        }
        "laser EM lamp V" <- w2297
        n1044 = Bundle By Name(cluster=w2294, "System Status.355 Laser"=w2300) -> (w2295:T22)
        n1045 = call <vilib>:"Add State(s) to Queue__JKI_lib_State_Machine.vi"("State(s) in (\"\")"=w2308) -> ("States Out"=w2307:string)  [unwired: 14 in]
      }
      frame "355 Laser: CheckPWMStatus" {
        # "Check 355 laser PWM status\n(Read LJ DIO#EF_ENABLE register to determine PWM status)"
        n1046 = Unbundle By Name(w2340) -> ("LJ Pinout.355 PWM"=w2341:string)
        n1047 = call "LabJack_FGV.vi"("Operation(Read)"=enum16{"Write", "Read"}."Read" ("Operation"), "error in (no error)"=w2344) -> ("error out"=w2347:errorcluster, "Read data"=w2348:i32)  [unwired: 8 in]
        n1048 = Concatenate Strings(w2341, "_EF_ENABLE" ("string")) -> (w2346:string)
        n1049 = call "LJM_eReadName.vi"("Handle In"=w2348, "Name"=w2346, "error in"=w2347) -> ("Value"=w2343:dbl, "error out"=w2345:errorcluster)  [unwired: 10 in, 1 out]
        n1050 = Greater Than 0?(x=w2343) -> (x > 0?=w2342:bool)
        n1051 = case shown="False" w2342 {
          frame False {
            # "PWM is off\nset color to gray"
            n1052 = local write "355nm Laser toggle"(FALSE ("355nm Laser")) -> ()
          }
          frame True {
            # "PWM is on\nset color to light green"
            n1053 = local write "355nm Laser toggle"(TRUE ("355nm Laser")) -> ()
          }
        }
        n1054 = call <vilib>:"Add State(s) to Queue__JKI_lib_State_Machine.vi"("State(s) in (\"\")"=w2353) -> ("States Out"=w2352:string)  [unwired: 14 in]
      }
      frame "355 Laser: Start" {
        # "Template Separator\n(You can make a copy of, or modify, this frame)"
        n1055 = call <vilib>:"Add State(s) to Queue__JKI_lib_State_Machine.vi"("State(s) in Front (\"\")"="LabJack: 355_PWM_Start", "State(s) in (\"\")"=w2361) -> ("States Out"=w2360:string)  [unwired: 13 in]
      }
      frame "355 Laser: Stop" {
        # "Template Separator\n(You can make a copy of, or modify, this frame)"
        n1056 = call <vilib>:"Add State(s) to Queue__JKI_lib_State_Machine.vi"("State(s) in Front (\"\")"="LabJack: 355_PWM_Stop", "State(s) in (\"\")"=w2367) -> ("States Out"=w2366:string)  [unwired: 13 in]
      }
      frame "---------- Utility ----------" {
        # "Template Separator\n(You can make a copy of, or modify, this frame)"
        n1057 = call <vilib>:"Add State(s) to Queue__JKI_lib_State_Machine.vi"("State(s) in (\"\")"=w2372) -> ("States Out"=w2371:string)  [unwired: 14 in]
      }
      frame "Utility: EnableGain?" {
        # "Enable or disable control V numeric control\n(Utility: EnableGain? >> True|False)"
        n1058 = case shown="\"True\", Default" w2373 {
          frame "False" {
            n1059 = property on="Ctrl V" class="DigNum (strict)"("DisabledEnum"=T11."Disabled and Grayed Out" ("Disabled")) -> ()  [unwired: 2 in, 2 out]
          }
          frame "True", Default {
            n1060 = property on="Ctrl V" class="DigNum (strict)"("DisabledEnum"=T11."Enabled" ("Disabled")) -> ()  [unwired: 2 in, 2 out]
          }
        }
        n1061 = call <vilib>:"Add State(s) to Queue__JKI_lib_State_Machine.vi"("State(s) in (\"\")"=w2378) -> ("States Out"=w2377:string)  [unwired: 14 in]
      }
      frame "Utility: SetDefaultMaxV" {
        # "Template Separator\n(You can make a copy of, or modify, this frame)"
        n1062 = local read "Ch1 Max CtrlV"() -> (w2381:dbl)
        n1063 = local write "Gain High"(w2381) -> ()
        n1064 = call <vilib>:"Add State(s) to Queue__JKI_lib_State_Machine.vi"("State(s) in (\"\")"=w2386) -> ("States Out"=w2385:string)  [unwired: 14 in]
      }
      frame "Utility: setSaveFlag" {
        # "Template Separator\n(You can make a copy of, or modify, this frame)"
        n1065 = Fract/Exp String To Number(string=w2387, default (0 dbl)=u8 0) -> (number=w2389:u8)  [unwired: 2 in, 1 out]
        n1066 = case shown="0, Default" w2389 {
          tunnel: [FALSE TRUE] -> w2388
          frame 0, Default {
          }
          frame 1 {
          }
        }
        n1067 = local write "SaveData?"(w2388) -> ()
        n1068 = call <vilib>:"Add State(s) to Queue__JKI_lib_State_Machine.vi"("State(s) in (\"\")"=w2395) -> ("States Out"=w2394:string)  [unwired: 14 in]
      }
      frame "Utility: Dewelling" {
        # "Main loop dewell\n(Dewelling >> #)"
        n1069 = Fract/Exp String To Number(string=w2400, default (0 dbl)=0) -> (number=w2398:i32)  [unwired: 2 in, 1 out]
        n1070 = Wait (ms)(milliseconds to wait=w2398) -> ()  [unwired: 1 out]
        n1071 = call <vilib>:"Add State(s) to Queue__JKI_lib_State_Machine.vi"("State(s) in (\"\")"=w2405) -> ("States Out"=w2404:string)  [unwired: 14 in]
      }
      frame "Utility: SetAllChanManualGain" {
        # "Template Separator\n(You can make a copy of, or modify, this frame)"
        n1072 = property on="Auto gain" class="Bool (strict)"("Val(Sgnl)"=FALSE ("Value (Signaling)")) -> ()  [unwired: 2 in, 2 out]
        n1073 = call <vilib>:"Add State(s) to Queue__JKI_lib_State_Machine.vi"("State(s) in (\"\")"=w2411) -> ("States Out"=w2410:string)  [unwired: 14 in]
      }
      frame "Utility: SetAllChanAutoGain" {
        # "Template Separator\n(You can make a copy of, or modify, this frame)"
        n1074 = property on="Auto gain" class="Bool (strict)"("Val(Sgnl)"=TRUE ("Value (Signaling)")) -> ()  [unwired: 2 in, 2 out]
        n1075 = call <vilib>:"Add State(s) to Queue__JKI_lib_State_Machine.vi"("State(s) in (\"\")"=w2417) -> ("States Out"=w2416:string)  [unwired: 14 in]
      }
      frame "---------- Graph ----------" {
        # "Template Separator\n(You can make a copy of, or modify, this frame)"
        n1076 = call <vilib>:"Add State(s) to Queue__JKI_lib_State_Machine.vi"("State(s) in (\"\")"=w2422) -> ("States Out"=w2421:string)  [unwired: 14 in]
      }
      frame "Graph: ClearHistory" {
        # "Clear intensity trace history\n(You can make a copy of, or modify, this frame)"
        n1077 = property on="Waveform Chart" class="WFChart (strict)"("History Data"=dbl[] []) -> ()  [unwired: 2 in, 2 out]
        n1078 = call <vilib>:"Add State(s) to Queue__JKI_lib_State_Machine.vi"("State(s) in (\"\")"=w2428) -> ("States Out"=w2427:string)  [unwired: 14 in]
      }
      frame "Graph: SetXScale" {
        # "Set X scale multiplier\n(Check digitizer aquisition speed and update x scale)"
        n1079 = local read "Channel"() -> (w2433:enum32{"Ch1", "Ch2", "Ch3"})
        n1080 = case shown="\"Ch1\", \"Ch2\", Default" w2433 {
          tunnel: w2432 -> [w2444 w2447]
          tunnel: [w2443 w2445] -> w2431
          tunnel: [w2442 w2446] -> w2430
          frame "Ch1", "Ch2", Default {
            n1081 = call "Digitizer1_FGV.vi"("error in (no error)"=w2444) -> ("error out"=w2443:errorcluster, "Read data"=w2442:refnum<k15>)  [unwired: 9 in]
          }
          frame "Ch3" {
            n1082 = call "Digitizer2_FGV.vi"("error in (no error)"=w2447) -> ("error out"=w2445:errorcluster, "Read data"=w2446:refnum<k15>)  [unwired: 9 in]
          }
        }
        n1083 = property on="Property Node" class="niScope"(reference=w2430, error in=w2431) -> (error out=w2435:errorcluster, "Min Sample Rate"=w2437:dbl)  [unwired: 1 out]
        n1084 = Divide(x=1.0, y=w2437) -> (x/y=w2436:dbl)
        "dt (s)" <- w2436
        n1085 = property on="Waveform (no average)" class="WFGraph (strict)"(error in=w2435, "XScale.Multiplier"=w2436) -> (error out=w2434:errorcluster)  [unwired: 1 in, 1 out]
        n1086 = call <vilib>:"Add State(s) to Queue__JKI_lib_State_Machine.vi"("State(s) in (\"\")"=w2441) -> ("States Out"=w2440:string)  [unwired: 14 in]
      }
      frame "Graph: AddCursors" {
        # "Add BG and DC cursor to all graphs\n(You can make a copy of, or modify, this frame)"
        n1087 = property on="Waveform (no average)" class="WFGraph (strict)"(error in=w2469) -> ("CrsrList"=w2455:T35, "XScale.Maximum"=w2463:dbl)  [unwired: 1 in, 2 out]
        n1088 = Multiply(x=w2463, y=0.8) -> (x*y=w2466:dbl)
        n1089 = Multiply(x=w2463, y=0.1) -> (x*y=w2459:dbl)
        n1090 = Multiply(x=w2463, y=0.9) -> (x*y=w2461:dbl)
        n1091 = Multiply(x=w2463, y=0.2) -> (x*y=w2458:dbl)
        n1092 = Build Array(w2466, w2461, w2459, w2458) -> (w2460:dbl[])
        n1093 = Index Array(array=w2455, index=4) -> (element=w2453:T36)
        n1094 = for {
          N: 4 -> [_]
          tunnel: w2455 -> [w2479] mode=indexing
          tunnel: w2460 -> [w2477] mode=indexing
          tunnel: [w2478] -> w2450 mode=indexing
          tunnel: u32[] [6618880, 6618880, 16711680, 16711680] -> [w2476] mode=indexing
          n1095 = Bundle By Name(cluster=w2479, "Position.X"=w2477, "Color"=w2476) -> (w2478:T36)
        }
        n1096 = Bundle By Name(cluster=w2453, "Position.Y"=0.0, "Color"=u32 6618880) -> (w2449:T36)
        n1097 = Build Array (concatenate)(w2450, w2449) -> (w2448:T37)
        n1098 = control-ref of="Waveform (no average)"() -> (w2457:refnum<vi>)
        n1099 = property on="Waveform (no average)" class="WFGraph (strict)"("CrsrList"=w2448) -> (error out=w2468:errorcluster)  [unwired: 2 in, 1 out]
        n1100 = call "UpdateCurserIdx(SubVI).vi"("error in (no error)"=w2468, "WaveformGraph in"=w2457) -> ("error out"=w2470:errorcluster)  [unwired: 9 in]
        n1101 = call <vilib>:"Add State(s) to Queue__JKI_lib_State_Machine.vi"("State(s) in (\"\")"=w2475) -> ("States Out"=w2474:string)  [unwired: 14 in]
      }
      frame "---------- APD ----------" {
        # "Template Separator\n(You can make a copy of, or modify, this frame)"
        n1102 = call <vilib>:"Add State(s) to Queue__JKI_lib_State_Machine.vi"("State(s) in (\"\")"=w2484) -> ("States Out"=w2483:string)  [unwired: 14 in]
      }
      frame "APD: Initialize" {
        w2490 = enum16{"Read", "Write"}."Write" ("Operation (Read)")
        w2491 = refnum<class "APDClass.lvclass"> refnum  # APDClass.lvclass
        # "Initialize APD FVG\n(You can make a copy of, or modify, this frame)"
        n1103 = call "APD2FGV.vi"("Error In"=w2488, "Operation (Read)"=w2490, "APDClass in"=w2491) -> ("Error Out"=w2485:errorcluster)  [unwired: 7 in, 1 out]
        n1104 = call "APD1FGV.vi"("Error In"=w2488, "Operation (Read)"=w2490, "APDClass in"=w2491) -> ("Error Out"=w2486:errorcluster)  [unwired: 7 in, 1 out]
        n1105 = call "APD3FGV.vi"("Error In"=w2488, "Operation (Read)"=w2490, "APDClass in"=w2491) -> ("Error Out"=w2489:errorcluster)  [unwired: 7 in, 1 out]
        n1106 = Merge Errors(w2486, w2485, w2489) -> (w2487:errorcluster)
        n1107 = call <vilib>:"Add State(s) to Queue__JKI_lib_State_Machine.vi"("State(s) in (\"\")"=w2495) -> ("States Out"=w2494:string)  [unwired: 14 in]
      }
      frame "APD: LoadFromSerial" {
        w2512 = enum16{"Read", "Write"}."Write" ("Operation (Read)")
        # "Load APD info based on serial numbers\n(update FGV)"
        n1108 = call "readAPDSerial.vi"("Error In"=w2497) -> ("Error Out"=w2496:errorcluster, "output cluster"=w2498:T38)  [unwired: 9 in]
        n1109 = Unbundle By Name(w2498) -> ("Ch1APDSerial#"=w2510:string, "Ch2APDSerial#"=w2508:string, "Ch3APDSerial#"=w2505:string)
        n1110 = Bundle By Name(cluster=w2501, "APDSerials"=w2498) -> (w2502:T22)
        n1111 = call "CreatFromSerialNum.vi"("error in (no error)"=w2496, "APD Serial #"=w2510) -> ("error out"=w2499:errorcluster, "APDClass out"=w2509:refnum<class "APDClass.lvclass">)  [unwired: 8 in]
        n1112 = call "CreatFromSerialNum.vi"("error in (no error)"=w2496, "APD Serial #"=w2508) -> ("error out"=w2507:errorcluster, "APDClass out"=w2503:refnum<class "APDClass.lvclass">)  [unwired: 8 in]
        n1113 = call "CreatFromSerialNum.vi"("error in (no error)"=w2496, "APD Serial #"=w2505) -> ("error out"=w2506:errorcluster, "APDClass out"=w2504:refnum<class "APDClass.lvclass">)  [unwired: 8 in]
        n1114 = call "APD1FGV.vi"("Error In"=w2499, "Operation (Read)"=w2512, "APDClass in"=w2509) -> ("Error Out"=w2511:errorcluster)  [unwired: 7 in, 1 out]
        n1115 = call "APD2FGV.vi"("Error In"=w2507, "Operation (Read)"=w2512, "APDClass in"=w2503) -> ("Error Out"=w2513:errorcluster)  [unwired: 7 in, 1 out]
        n1116 = call "APD3FGV.vi"("Error In"=w2506, "Operation (Read)"=w2512, "APDClass in"=w2504) -> ("Error Out"=w2514:errorcluster)  [unwired: 7 in, 1 out]
        n1117 = call <vilib>:"Add State(s) to Queue__JKI_lib_State_Machine.vi"("State(s) in (\"\")"=w2517) -> ("States Out"=w2516:string)  [unwired: 14 in]
        n1118 = Merge Errors(w2511, w2513, w2514) -> (w2500:errorcluster)
      }
      frame "APD: LoadFromSerialNoRawData" {
        w2534 = enum16{"Read", "Write"}."Write" ("Operation (Read)")
        # "Load APD info based on serial numbers\n(update FGV)"
        n1119 = disable-structure shown="Disabled" {
          frame Disabled {
            w2540 = T39 {"Ch1APDSerial#"="", "Ch2APDSerial#"="", "Ch3APDSerial#"=""}  # APD Serials
            n1120 = call <vilib>:"Application Directory.vi"() -> ("Application Directory"=w2547:path)
            n1121 = Build Path(base path=w2547, name or relative path="ConfigFiles\\APDSerial.txt") -> (appended path=w2545:path)
            n1122 = Read from Text File(file (use dialog)=w2545) -> (text=w2543:string, error out=w2544:errorcluster)  [unwired: 3 in, 2 out]
            n1123 = call <vilib>:"Unflatten From JSON String.vi"("Type and Defaults"=w2540, "error in"=w2544, "JSON String"=w2543) -> ("error out"=w2541:errorcluster, "Variant"=w2542:variant)  [unwired: 7 in]
            n1124 = Variant To Data(error in=w2541, type=w2540, Variant=w2542) -> ()  [unwired: 2 out]
          }
          frame Enabled {
          }
        }
        n1125 = call "readAPDSerial.vi"("Error In"=w2519) -> ("Error Out"=w2518:errorcluster, "output cluster"=w2520:T38)  [unwired: 9 in]
        n1126 = Unbundle By Name(w2520) -> ("Ch1APDSerial#"=w2532:string, "Ch2APDSerial#"=w2530:string, "Ch3APDSerial#"=w2527:string)
        n1127 = Bundle By Name(cluster=w2523, "APDSerials"=w2520) -> (w2524:T22)
        n1128 = call "CreatFromSerialNumNoRaw.vi"("error in (no error)"=w2518, "APD Serial #"=w2532) -> ("error out"=w2521:errorcluster, "APDClass out"=w2531:refnum<class "APDClass.lvclass">)  [unwired: 8 in]
        n1129 = call "CreatFromSerialNumNoRaw.vi"("error in (no error)"=w2518, "APD Serial #"=w2530) -> ("error out"=w2529:errorcluster, "APDClass out"=w2525:refnum<class "APDClass.lvclass">)  [unwired: 8 in]
        n1130 = call "CreatFromSerialNumNoRaw.vi"("error in (no error)"=w2518, "APD Serial #"=w2527) -> ("error out"=w2528:errorcluster, "APDClass out"=w2526:refnum<class "APDClass.lvclass">)  [unwired: 8 in]
        n1131 = call "APD1FGV.vi"("Error In"=w2521, "Operation (Read)"=w2534, "APDClass in"=w2531) -> ("Error Out"=w2533:errorcluster)  [unwired: 7 in, 1 out]
        n1132 = call "APD2FGV.vi"("Error In"=w2529, "Operation (Read)"=w2534, "APDClass in"=w2525) -> ("Error Out"=w2535:errorcluster)  [unwired: 7 in, 1 out]
        n1133 = call "APD3FGV.vi"("Error In"=w2528, "Operation (Read)"=w2534, "APDClass in"=w2526) -> ("Error Out"=w2536:errorcluster)  [unwired: 7 in, 1 out]
        n1134 = call <vilib>:"Add State(s) to Queue__JKI_lib_State_Machine.vi"("State(s) in (\"\")"=w2539) -> ("States Out"=w2538:string)  [unwired: 14 in]
        n1135 = Merge Errors(w2533, w2535, w2536) -> (w2522:errorcluster)
      }
      frame "APD: GetGainLimits" {
        w2562 = enum16{"Read", "Write"}."Read" ("Operation (Read)")
        # "Template Separator\n(You can make a copy of, or modify, this frame)"
        n1136 = call "APD1FGV.vi"("Error In"=w2548, "Operation (Read)"=w2562) -> ("Error Out"=w2560:errorcluster, "APDClass out"=w2561:refnum<class "APDClass.lvclass">)  [unwired: 8 in]
        n1137 = call "APD2FGV.vi"("Error In"=w2548, "Operation (Read)"=w2562) -> ("Error Out"=w2557:errorcluster, "APDClass out"=w2558:refnum<class "APDClass.lvclass">)  [unwired: 8 in]
        n1138 = call "APD3FGV.vi"("Error In"=w2548, "Operation (Read)"=w2562) -> ("Error Out"=w2555:errorcluster, "APDClass out"=w2556:refnum<class "APDClass.lvclass">)  [unwired: 8 in]
        n1139 = call-dynamic "Read Gain Limits(Log).vi"("error in (no error)"=w2560, "APDClass in"=w2561) -> ("error out"=w2552:errorcluster, "GainLimits(Log)"=w2559:cluster{"GainMax":dbl, "GainMin":dbl})  [unwired: 7 in, 1 out]
        n1140 = call-dynamic "Read Gain Limits(Log).vi"("error in (no error)"=w2557, "APDClass in"=w2558) -> ("error out"=w2551:errorcluster, "GainLimits(Log)"=w2554:cluster{"GainMax":dbl, "GainMin":dbl})  [unwired: 7 in, 1 out]
        n1141 = call-dynamic "Read Gain Limits(Log).vi"("error in (no error)"=w2555, "APDClass in"=w2556) -> ("error out"=w2550:errorcluster, "GainLimits(Log)"=w2553:cluster{"GainMax":dbl, "GainMin":dbl})  [unwired: 7 in, 1 out]
        n1142 = global write "GlobalVariables.vi" "Ch1GainLim(Log)"(w2559) -> ()
        n1143 = global write "GlobalVariables.vi" "Ch2GainLim(Log)"(w2554) -> ()
        n1144 = global write "GlobalVariables.vi" "Ch3GainLim(Log)"(w2553) -> ()
        n1145 = Merge Errors(w2552, w2551, w2550) -> (w2549:errorcluster)
        n1146 = call <vilib>:"Add State(s) to Queue__JKI_lib_State_Machine.vi"("State(s) in (\"\")"=w2566) -> ("States Out"=w2565:string)  [unwired: 14 in]
      }
      frame "APD: UpdateIndicator" {
        # "Update APD module front panel indicators\n(Read data, update FGV, update plot)"
        n1147 = call "APD3FGV.vi"() -> ("Error Out"=w2604:errorcluster, "APDClass out"=w2605:refnum<class "APDClass.lvclass">)  [unwired: 10 in]
        n1148 = call "APD2FGV.vi"() -> ("Error Out"=w2612:errorcluster, "APDClass out"=w2613:refnum<class "APDClass.lvclass">)  [unwired: 10 in]
        n1149 = call "APD1FGV.vi"() -> ("Error Out"=w2625:errorcluster, "APDClass out"=w2626:refnum<class "APDClass.lvclass">)  [unwired: 10 in]
        n1150 = call-dynamic "Read APD Serial.vi"("error in (no error)"=w2604, "APDClass in"=w2605) -> ("error out"=w2590:errorcluster, "APD Serial #"=w2597:string, "APDClass out"=w2591:refnum<class "APDClass.lvclass">)  [unwired: 7 in]
        n1151 = call-dynamic "Read APD Serial.vi"("error in (no error)"=w2612, "APDClass in"=w2613) -> ("error out"=w2584:errorcluster, "APD Serial #"=w2611:string, "APDClass out"=w2586:refnum<class "APDClass.lvclass">)  [unwired: 7 in]
        n1152 = call-dynamic "Read APD Serial.vi"("error in (no error)"=w2625, "APDClass in"=w2626) -> ("error out"=w2579:errorcluster, "APD Serial #"=w2622:string, "APDClass out"=w2581:refnum<class "APDClass.lvclass">)  [unwired: 7 in]
        n1153 = call-dynamic "Read DateTime.vi"("error in (no error)"=w2590, "APDClass in"=w2591) -> ("error out"=w2588:errorcluster, "DateTime"=→"DateTimeCh1":string, "APDClass out"=w2589:refnum<class "APDClass.lvclass">)  [unwired: 7 in]
        n1154 = call-dynamic "Read DateTime.vi"("error in (no error)"=w2584, "APDClass in"=w2586) -> ("error out"=w2583:errorcluster, "DateTime"=→"DateTimeCh2":string, "APDClass out"=w2585:refnum<class "APDClass.lvclass">)  [unwired: 7 in]
        n1155 = call-dynamic "Read DateTime.vi"("error in (no error)"=w2579, "APDClass in"=w2581) -> ("error out"=w2578:errorcluster, "DateTime"=→"DateTimeCh3":string, "APDClass out"=w2580:refnum<class "APDClass.lvclass">)  [unwired: 7 in]
        n1156 = local write "Serial Number Ch3"(w2597) -> ()
        n1157 = local write "Serial Number Ch2"(w2611) -> ()
        n1158 = local write "Serial Number Ch1"(w2622) -> ()
        n1159 = call-dynamic "Read GainData.vi"("error in (no error)"=w2588, "APDClass in"=w2589) -> ("error out"=w2603:errorcluster, "GainData"=w2576:T40, "APDClass out"=w2614:refnum<class "APDClass.lvclass">)  [unwired: 7 in]
        n1160 = call-dynamic "Read GainData.vi"("error in (no error)"=w2583, "APDClass in"=w2585) -> ("error out"=w2615:errorcluster, "GainData"=w2595:T40, "APDClass out"=w2616:refnum<class "APDClass.lvclass">)  [unwired: 7 in]
        n1161 = call-dynamic "Read GainData.vi"("error in (no error)"=w2578, "APDClass in"=w2580) -> ("error out"=w2623:errorcluster, "GainData"=w2593:T40, "APDClass out"=w2624:refnum<class "APDClass.lvclass">)  [unwired: 7 in]
        n1162 = Unbundle By Name(w2595) -> ("CtrlV"=w2572:dbl[], "Gain"=w2571:dbl[])
        n1163 = Unbundle By Name(w2576) -> ("CtrlV"=w2575:dbl[], "Gain"=w2574:dbl[])
        n1164 = Unbundle By Name(w2593) -> ("CtrlV"=w2569:dbl[], "Gain"=w2568:dbl[])
        n1165 = Array Max & Min(array=w2575) -> (max value=→"Ch1 Max CtrlV":dbl)  [unwired: 3 out]
        n1166 = Bundle("CtrlV"=w2569, "Gain"=w2568) -> (→"Ch1 Gain":cluster{"CtrlV":dbl[], "Gain":dbl[]})  [unwired: 1 in]
        n1167 = Bundle("CtrlV"=w2572, "Gain"=w2571) -> (→"Ch2 Gain":cluster{"CtrlV":dbl[], "Gain":dbl[]})  [unwired: 1 in]
        n1168 = Bundle("CtrlV"=w2575, "Gain"=w2574) -> (→"Ch3 Gain":cluster{"CtrlV":dbl[], "Gain":dbl[]})  [unwired: 1 in]
        n1169 = call-dynamic "Read iRFData.vi"("error in (no error)"=w2603, "APDClass in"=w2614) -> ("error out"=w2602:errorcluster, "iRFData"=w2598:T41)  [unwired: 7 in, 1 out]
        n1170 = call-dynamic "Read iRFData.vi"("error in (no error)"=w2615, "APDClass in"=w2616) -> ("error out"=w2607:errorcluster, "iRFData"=w2610:T41)  [unwired: 7 in, 1 out]
        n1171 = call-dynamic "Read iRFData.vi"("error in (no error)"=w2623, "APDClass in"=w2624) -> ("error out"=w2618:errorcluster, "iRFData"=w2621:T41)  [unwired: 7 in, 1 out]
        n1172 = Array Max & Min(array=w2572) -> (max value=→"Ch2 Max CtrlV":dbl)  [unwired: 3 out]
        n1173 = Array Max & Min(array=w2569) -> (max value=→"Ch3 Max CtrlV":dbl)  [unwired: 3 out]
        n1174 = Unbundle By Name(w2610) -> ("iRFWFsAvg"=→"Ch2 iRF Graph":dbl[][], "dt"=w2608:dbl)
        n1175 = Unbundle By Name(w2598) -> ("iRFWFsAvg"=→"Ch3 iRF Graph":dbl[][], "dt"=w2600:dbl)
        n1176 = Unbundle By Name(w2621) -> ("iRFWFsAvg"=→"Ch1 iRF Graph":dbl[][], "dt"=w2619:dbl)
        n1177 = property on="Ch3 iRF Graph" class="WFGraph (strict)"(error in=w2602, "XScale.Multiplier"=w2600) -> (error out=w2601:errorcluster)  [unwired: 1 in, 1 out]
        n1178 = property on="Ch2 iRF Graph" class="WFGraph (strict)"(error in=w2607, "XScale.Multiplier"=w2608) -> (error out=w2606:errorcluster)  [unwired: 1 in, 1 out]
        n1179 = property on="Ch1 iRF Graph" class="WFGraph (strict)"(error in=w2618, "XScale.Multiplier"=w2619) -> (error out=w2617:errorcluster)  [unwired: 1 in, 1 out]
        n1180 = call <vilib>:"Add State(s) to Queue__JKI_lib_State_Machine.vi"("State(s) in (\"\")"=w2631) -> ("States Out"=w2630:string)  [unwired: 14 in]
        n1181 = Merge Errors(w2617, w2606, w2601) -> (w2627:errorcluster)
      }
      frame "APD: writeGain" {
        w2632 = T40 {"CtrlV"=[], "NumOfWFs"=0, "WF length"=0, "Gain"=[], "GainRaw"=[], "GainBGRaw"=[]}  # GainData
        # "Parse all data for all gain\n(parse data all gain)"
        n1182 = Flush Queue(queue=w2644, error in (no error)=w2645) -> (remaining elements=w2641:cluster{"CtrlV":dbl, "WFs":dbl[][]}[], error out=w2639:errorcluster)  [unwired: 1 out]
        n1183 = for {
          tunnel: w2641 -> [w2680] mode=indexing
          tunnel: [w2679] -> w2638 mode=indexing
          tunnel: [w2676] -> w2634
          tunnel: [w2673] -> w2633
          # "Reshape gain WF array to vectors"
          n1184 = Unbundle By Name(w2680) -> ("WFs"=w2678:dbl[][])
          n1185 = Array Size(array=w2678) -> (size(s)=w2677:i32[])
          n1186 = for {
            tunnel: w2678 -> [w2681] mode=indexing
            tunnel: [w2681] -> w2679 mode=concatenating
          }
          n1187 = Index Array(array=w2677, index #1=0 ("index"), index #2=1 ("index")) -> (element #1=w2673:i32, element #2=w2676:i32)
        }
        n1188 = local read "Ctrl V"() -> (w2636:dbl[])
        n1189 = local read "Gain"() -> (w2635:dbl[])
        n1190 = Bundle By Name(cluster=w2632, "CtrlV"=w2636, "Gain"=w2635, "WF length"=w2634, "NumOfWFs"=w2633, "GainRaw"=w2638) -> (w2637:T40)
        n1191 = local read "Channel"() -> (w2640:enum32{"Ch1", "Ch2", "Ch3"})
        n1192 = case shown="\"Ch1\", Default" w2640 {
          tunnel: [w2650 w2657 w2665] -> w2643
          tunnel: w2639 -> [w2656 w2664 w2672]
          tunnel: w2637 -> [w2654 w2661 w2669]
          frame "Ch1", Default {
            n1193 = call "APD1FGV.vi"("Error In"=w2656) -> ("Error Out"=w2655:errorcluster, "APDClass out"=w2653:refnum<class "APDClass.lvclass">)  [unwired: 9 in]
            n1194 = call-dynamic "Write GainData.vi"("error in (no error)"=w2655, "GainData"=w2654, "APDClass in"=w2653) -> ("error out"=w2651:errorcluster, "APDClass out"=w2652:refnum<class "APDClass.lvclass">)  [unwired: 7 in]
            n1195 = call "APD1FGV.vi"("Error In"=w2651, "Operation (Read)"=enum16{"Read", "Write"}."Write", "APDClass in"=w2652) -> ("Error Out"=w2650:errorcluster)  [unwired: 7 in, 1 out]
          }
          frame "Ch2" {
            n1196 = call "APD2FGV.vi"("Error In"=w2664) -> ("Error Out"=w2662:errorcluster, "APDClass out"=w2663:refnum<class "APDClass.lvclass">)  [unwired: 9 in]
            n1197 = call-dynamic "Write GainData.vi"("error in (no error)"=w2662, "GainData"=w2661, "APDClass in"=w2663) -> ("error out"=w2658:errorcluster, "APDClass out"=w2660:refnum<class "APDClass.lvclass">)  [unwired: 7 in]
            n1198 = call "APD2FGV.vi"("Error In"=w2658, "Operation (Read)"=enum16{"Read", "Write"}."Write", "APDClass in"=w2660) -> ("Error Out"=w2657:errorcluster)  [unwired: 7 in, 1 out]
          }
          frame "Ch3" {
            n1199 = call "APD3FGV.vi"("Error In"=w2672) -> ("Error Out"=w2670:errorcluster, "APDClass out"=w2671:refnum<class "APDClass.lvclass">)  [unwired: 9 in]
            n1200 = call-dynamic "Write GainData.vi"("error in (no error)"=w2670, "GainData"=w2669, "APDClass in"=w2671) -> ("error out"=w2666:errorcluster, "APDClass out"=w2668:refnum<class "APDClass.lvclass">)  [unwired: 7 in]
            n1201 = call "APD3FGV.vi"("Error In"=w2666, "Operation (Read)"=enum16{"Read", "Write"}."Write", "APDClass in"=w2668) -> ("Error Out"=w2665:errorcluster)  [unwired: 7 in, 1 out]
          }
        }
        n1202 = call <vilib>:"Add State(s) to Queue__JKI_lib_State_Machine.vi"("State(s) in (\"\")"=w2648) -> ("States Out"=w2647:string)  [unwired: 14 in]
      }
      frame "APD: writeiRF" {
        w2691 = T41 {"dt"=0.0, "NumOfWFs"=0, "WFLength"=0, "iRFCtrlV"=[], "iRFWFsAvg"=[], "iRFRaw"=[]}  # iRF
        # "Parse all data for all gain\n(parse data all gain)"
        n1203 = Flush Queue(queue=w2700, error in (no error)=w2698) -> (remaining elements=w2696:T42, error out=w2693:errorcluster)  [unwired: 1 out]
        n1204 = for {
          tunnel: w2696 -> [w2739] mode=indexing
          tunnel: [w2737] -> w2689 mode=indexing
          tunnel: [w2738] -> w2688 mode=indexing
          tunnel: [w2736] -> w2690 mode=indexing
          shift-right: [w2732] -> w2687
          shift-left: i32[] [] -> [w2731]
          i -> [w2735]
          n1205 = Equal To 0?(x=w2735) -> (x = 0?=w2734:bool)
          n1206 = Unbundle By Name(w2739) -> ("CtrlV"=w2737:dbl, "WFavg"=w2738:dbl[], "WFs"=w2733:dbl[][])
          n1207 = case shown="True" w2734 {
            tunnel: w2733 -> [_ w2742]
            tunnel: [w2740 w2741] -> w2732
            tunnel: w2731 -> [w2740 _]
            frame False {
            }
            frame True {
              n1208 = Array Size(array=w2742) -> (size(s)=w2741:i32[])
            }
          }
          n1209 = for {
            tunnel: w2733 -> [w2743] mode=indexing
            tunnel: [w2743] -> w2736 mode=concatenating
          }
        }
        n1210 = Index Array(array=w2687, index #1=0 ("index (row)"), index #2=1 ("disabled index (col)")) -> (element #1=w2683:i32, element #2=w2682:i32)
        n1211 = Bundle By Name(cluster=w2691, "dt"=0.2, "NumOfWFs"=w2683, "WFLength"=w2682, "iRFCtrlV"=w2689, "iRFWFsAvg"=w2688, "iRFRaw"=w2690) -> (w2692:T41)
        n1212 = local read "Channel"() -> (w2694:enum32{"Ch1", "Ch2", "Ch3"})
        n1213 = case shown="\"Ch3\"" w2694 {
          tunnel: w2693 -> [w2712 w2720 w2729]
          tunnel: w2688 -> [w2711 w2721 w2730]
          tunnel: w2692 -> [w2709 w2717 w2724]
          tunnel: [w2704 w2713 w2722] -> w2699
          frame "Ch1", Default {
            n1214 = local write "Ch1 iRF Graph"(w2711) -> ()
            n1215 = call "APD1FGV.vi"("Error In"=w2712) -> ("Error Out"=w2710:errorcluster, "APDClass out"=w2708:refnum<class "APDClass.lvclass">)  [unwired: 9 in]
            n1216 = call-dynamic "Write iRFData.vi"("error in (no error)"=w2710, "iRFData"=w2709, "APDClass in"=w2708) -> ("error out"=w2707:errorcluster, "APDClass out"=w2706:refnum<class "APDClass.lvclass">)  [unwired: 7 in]
            n1217 = call "APD1FGV.vi"("Error In"=w2707, "Operation (Read)"=enum16{"Read", "Write"}."Write", "APDClass in"=w2706) -> ("Error Out"=w2704:errorcluster)  [unwired: 7 in, 1 out]
          }
          frame "Ch2" {
            n1218 = local write "Ch2 iRF Graph"(w2721) -> ()
            n1219 = call "APD2FGV.vi"("Error In"=w2720) -> ("Error Out"=w2719:errorcluster, "APDClass out"=w2718:refnum<class "APDClass.lvclass">)  [unwired: 9 in]
            n1220 = call-dynamic "Write iRFData.vi"("error in (no error)"=w2719, "iRFData"=w2717, "APDClass in"=w2718) -> ("error out"=w2715:errorcluster, "APDClass out"=w2716:refnum<class "APDClass.lvclass">)  [unwired: 7 in]
            n1221 = call "APD2FGV.vi"("Error In"=w2715, "Operation (Read)"=enum16{"Read", "Write"}."Write", "APDClass in"=w2716) -> ("Error Out"=w2713:errorcluster)  [unwired: 7 in, 1 out]
          }
          frame "Ch3" {
            n1222 = local write "Ch3 iRF Graph"(w2730) -> ()
            n1223 = call "APD3FGV.vi"("Error In"=w2729) -> ("Error Out"=w2728:errorcluster, "APDClass out"=w2726:refnum<class "APDClass.lvclass">)  [unwired: 9 in]
            n1224 = call-dynamic "Write iRFData.vi"("error in (no error)"=w2728, "iRFData"=w2724, "APDClass in"=w2726) -> ("error out"=w2727:errorcluster, "APDClass out"=w2725:refnum<class "APDClass.lvclass">)  [unwired: 7 in]
            n1225 = call "APD3FGV.vi"("Error In"=w2727, "Operation (Read)"=enum16{"Read", "Write"}."Write", "APDClass in"=w2725) -> ("Error Out"=w2722:errorcluster)  [unwired: 7 in, 1 out]
          }
        }
        n1226 = call <vilib>:"Add State(s) to Queue__JKI_lib_State_Machine.vi"("State(s) in (\"\")"=w2703) -> ("States Out"=w2702:string)  [unwired: 14 in]
      }
      frame "APD: SaveNew" {
        # "Save APD info\n(You can make a copy of, or modify, this frame)"
        n1227 = local read "Channel"() -> (w2748:enum32{"Ch1", "Ch2", "Ch3"})
        n1228 = case shown="\"Ch1\", Default" w2748 {
          tunnel: [w2757 w2760 w2763] -> w2747
          tunnel: w2746 -> [w2756 w2758 w2761]
          tunnel: [w2755 w2759 w2762] -> w2745
          frame "Ch1", Default {
            n1229 = call "APD1FGV.vi"("Error In"=w2756) -> ("Error Out"=w2755:errorcluster, "APDClass out"=w2757:refnum<class "APDClass.lvclass">)  [unwired: 9 in]
          }
          frame "Ch2" {
            n1230 = call "APD2FGV.vi"("Error In"=w2758) -> ("Error Out"=w2759:errorcluster, "APDClass out"=w2760:refnum<class "APDClass.lvclass">)  [unwired: 9 in]
          }
          frame "Ch3" {
            n1231 = call "APD3FGV.vi"("Error In"=w2761) -> ("Error Out"=w2762:errorcluster, "APDClass out"=w2763:refnum<class "APDClass.lvclass">)  [unwired: 9 in]
          }
        }
        n1232 = call "Write to File.vi"("Error In"=w2745, "APDClass.lvclass"=w2747) -> ("Error Out"=w2744:errorcluster)  [unwired: 9 in]
        n1233 = case shown="Error .." w2744 {
          frame No Error {
            n1234 = One Button Dialog(message="Data saved successfully!") -> ()  [unwired: 1 in, 1 out]
          }
          frame Error {
            n1235 = One Button Dialog(message="Error saving to APD file!") -> ()  [unwired: 1 in, 1 out]
          }
        }
        n1236 = call <vilib>:"Add State(s) to Queue__JKI_lib_State_Machine.vi"("State(s) in (\"\")"=w2752) -> ("States Out"=w2751:string)  [unwired: 14 in]
      }
      frame "---------- Aquisition ----------" {
        # "Template Separator\n(You can make a copy of, or modify, this frame)"
        n1237 = call <vilib>:"Add State(s) to Queue__JKI_lib_State_Machine.vi"("State(s) in (\"\")"=w2768) -> ("States Out"=w2767:string)  [unwired: 14 in]
      }
      frame "Aquisition: EnqueueV" {
        # "Enqueue aquisition V\n(You can make a copy of, or modify, this frame)"
        n1238 = while {
          tunnel: w2773 -> [w2791]
          shift-right: [w2789] -> w2772
          shift-left: w2771 -> [w2790]
          shift-right: [w2783] -> _
          shift-left: "Gain low" -> [w2787]
          tunnel: "Step" -> [w2784]
          tunnel: "Gain High" -> [w2785]
          tunnel: "Gain low" -> [w2788]
          stop <- w2782 stop-if-true
          # "check gain value, stop if out of range"
          n1239 = Add(x=w2785, y=w2784) -> (x+y=w2781:dbl)
          n1240 = In Range and Coerce(upper limit=w2785, x=w2787, lower limit=w2788) -> (coerced(x)=w2786:dbl)  [unwired: 1 out]
          n1241 = Enqueue Element(queue=w2791, element=w2786, error in (no error)=w2790) -> (error out=w2789:errorcluster)  [unwired: 1 in, 2 out]
          n1242 = Subtract(x=w2781, y=0.0001) -> (x-y=w2779:dbl)
          n1243 = Add(x=w2787, y=w2784) -> (x+y=w2783:dbl)
          n1244 = Greater Or Equal?(x=w2783, y=w2779) -> (x >= y?=w2782:bool)
        }
        n1245 = call <vilib>:"Add State(s) to Queue__JKI_lib_State_Machine.vi"("State(s) in (\"\")"=w2778) -> ("States Out"=w2777:string)  [unwired: 14 in]
      }
      frame "Aquisition: RecordData" {
        # "Set gain\nstart aquisition\nask user to adjust signal level\nstop aquisition\nstart aquisition"
        # "Template Separator\n(You can make a copy of, or modify, this frame)"
        n1246 = Fract/Exp String To Number(string=w2792) -> (number=w2797:dbl)  [unwired: 3 in, 1 out]
        n1247 = call "V1FGV.vi"("Error In"=w2796, "action (write)"=enum16{"write", "read"}."write" ("action"), "V1 in"=w2797) -> ("Error Out"=w2795:errorcluster)  [unwired: 7 in, 1 out]
        n1248 = call <vilib>:"Add State(s) to Queue__JKI_lib_State_Machine.vi"("State(s) in Front (\"\")"="Queue: Flash\nUtility: setSaveFlag >> 0\nMacro: StartRun\nUI: ShowDialog\nUtility: setSaveFlag >> 1\nQueue: CheckNumOfWF\nMacro: StopRun\n" ("State(s) in Front (\"\")"), "State(s) in (\"\")"=w2801) -> ("States Out"=w2800:string)  [unwired: 13 in]
      }
      frame "---------- File ----------" {
        # "Template Separator\n(You can make a copy of, or modify, this frame)"
        n1249 = call <vilib>:"Add State(s) to Queue__JKI_lib_State_Machine.vi"("State(s) in (\"\")"=w2806) -> ("States Out"=w2805:string)  [unwired: 14 in]
      }
      frame "File: BackupOld" {
        w2814 = ".tdms" ("string")
        # ".tdms_index file is not required for storage or distribution and automatically regenerates\nno need to copy the index file"
        # "Backup old APD data file\n()"
        n1250 = local read "Channel"() -> (w2824:enum32{"Ch1", "Ch2", "Ch3"})
        n1251 = case shown="\"Ch1\", Default" w2824 {
          tunnel: [w2829 w2830 w2831] -> w2815
          frame "Ch1", Default {
            n1252 = local read "Serial Number Ch1"() -> (w2829:string)
          }
          frame "Ch2" {
            n1253 = local read "Serial Number Ch2"() -> (w2830:string)
          }
          frame "Ch3" {
            n1254 = local read "Serial Number Ch3"() -> (w2831:string)
          }
        }
        n1255 = call <vilib>:"Application Directory.vi"() -> ("Application Directory"=w2825:path)
        n1256 = Get Date/Time In Seconds() -> (seconds since 1Jan1904=w2819:timestamp)
        n1257 = Format Date/Time String(time format string (%c)="%m-%d-%Y %H-%M", seconds (now)=w2819) -> (date/time string=w2818:string)  [unwired: 1 in]
        n1258 = Build Path(base path=w2825, name or relative path="ConfigFiles") -> (appended path=w2822:path)
        n1259 = Build Path(base path=w2822, name or relative path="Backup") -> (appended path=w2821:path)
        n1260 = Concatenate Strings(w2815, w2814) -> (w2816:string)
        n1261 = Concatenate Strings(w2815, " BK " ("string"), w2818, w2814) -> (w2817:string)
        n1262 = Build Path(base path=w2822, name or relative path=w2816) -> (appended path=w2823:path)
        n1263 = Build Path(base path=w2821, name or relative path=w2817) -> (appended path=w2820:path)
        n1264 = Copy(8:w2809, 10:w2820, 11:w2823) -> (0:w2808:errorcluster)  [unwired: 2 in, 2 out]
        n1265 = call <vilib>:"Add State(s) to Queue__JKI_lib_State_Machine.vi"("State(s) in (\"\")"=w2828) -> ("States Out"=w2827:string)  [unwired: 14 in]
      }
      frame "---------- PID ----------" {
        # "Template Separator\n(You can make a copy of, or modify, this frame)"
        n1266 = call <vilib>:"Add State(s) to Queue__JKI_lib_State_Machine.vi"("State(s) in (\"\")"=w2836) -> ("States Out"=w2835:string)  [unwired: 14 in]
      }
      frame "PID: loadPID" {
        # "Template Separator\n(You can make a copy of, or modify, this frame)"
        n1267 = call "readPIDSetting.vi"("Error In"=w2840) -> ("Error Out"=w2841:errorcluster, "Ch3 PID out"=w2837:T6, "Ch2 PID out"=w2838:T6, "Ch1 PID out"=w2839:T6)  [unwired: 7 in]
        n1268 = local write "Ch1 PID gains"(w2839) -> ()
        n1269 = local write "Ch2 PID gains"(w2838) -> ()
        n1270 = local write "Ch3 PID gains"(w2837) -> ()
        n1271 = call <vilib>:"Add State(s) to Queue__JKI_lib_State_Machine.vi"("State(s) in (\"\")"=w2845) -> ("States Out"=w2844:string)  [unwired: 14 in]
      }
      frame "---------- Template ----------" {
        # "Template Separator\n(You can make a copy of, or modify, this frame)"
        n1272 = call <vilib>:"Add State(s) to Queue__JKI_lib_State_Machine.vi"("State(s) in (\"\")"=w2850) -> ("States Out"=w2849:string)  [unwired: 14 in]
      }
    }
  }
  n1273 = while {
    tunnel: w39 -> [w2883]
    shift-right: [w2865] -> _
    shift-left: w26 -> [w2864]
    tunnel: w36 -> [w2876]
    tunnel: [w2874] -> w35
    shift-right: [w2873] -> _
    shift-left: w23 -> [w2872]
    i -> [w2868]
    stop <- w2867 stop-if-true
    # "stop on error"
    # "Gain adjustment and Data processing"
    n1274 = Wait on Notification(notifier=w2883, ignore previous (F)=TRUE) -> (notification=w2881:cluster{"idx":i32, "CH1&2":dbl[][]}, error out=w2858:errorcluster)  [unwired: 2 in, 2 out]
    n1275 = call <vilib>:"High Resolution Relative Seconds.vi"() -> ("relative seconds"=w2873:dbl)
    n1276 = flat-sequence {
      tunnel: [w2993] -> w2852
      tunnel: w2858 -> [_]
      frame #0 {
        # "make sure it is read after data arrive"
        n1277 = local read "Auto gain"() -> (w2993:bool)
      }
    }
    n1278 = Subtract(x=w2873, y=w2872) -> (x-y=w2871:dbl)
    n1279 = Unbundle(w2881) -> ("CH1&2"=w2863:dbl[][])  [unwired: 1 out]
    n1280 = call "AvgArrayTimeCritical.vi"("2D array"=w2863) -> ("1D Avg"=w2862:dbl[])  [unwired: 10 in]
    n1281 = Multiply(x=w2871, y=1000.0) -> (x*y=→"processing loop timing(ms)":dbl)
    n1282 = Array Max & Min(array=w2862) -> (max value=w2855:dbl)  [unwired: 3 out]
    n1283 = local read "Channel"() -> (w2851:enum32{"Ch1", "Ch2", "Ch3"})
    n1284 = case shown="True" w2852 {
      tunnel: [w2888 w2918] -> w2859
      tunnel: w2858 -> [w2889 w2917]
      tunnel: [w2889 w2916] -> w2857
      tunnel: "V target(1.0)" -> [_ w2915]
      tunnel: w2855 -> [_ w2914]
      tunnel: [w2884 w2912] -> w2854
      tunnel: [w2885 w2911] -> w2853
      tunnel: w2851 -> [w2887 w2910]
      frame False {
        n1285 = case shown="\"Ch1\", Default" w2887 {
          tunnel: [w2892 w2894 w2896] -> w2888
          tunnel: [enum16{"Ch1", "Ch2", "Ch3"}."Ch1" ("Channel") enum16{"Ch1", "Ch2", "Ch3"}."Ch2" ("Channel") enum16{"Ch1", "Ch2", "Ch3"}."Ch3" ("Channel")] -> w2886
          frame "Ch1", Default {
            n1286 = global read "GlobalVariables.vi" "Ch1 LJ pin"() -> (w2892:string)
          }
          frame "Ch2" {
            n1287 = global read "GlobalVariables.vi" "Ch2 LJ pin"() -> (w2894:string)
          }
          frame "Ch3" {
            n1288 = global read "GlobalVariables.vi" "Ch3 LJ pin"() -> (w2896:string)
          }
        }
        n1289 = call "V1FGV.vi"("action (write)"=enum16{"write", "read"}."read" ("action")) -> ("V1 out"=w2885:dbl)  [unwired: 9 in, 1 out]
        n1290 = call "CtrlVtoGain.vi"("CtrlV(V)"=w2885, "Channel"=w2886) -> ("Gain"=w2884:dbl)  [unwired: 8 in, 1 out]
      }
      frame True {
        n1291 = case shown="\"Ch1\", Default" w2910 {
          tunnel: [w2943 w2967 w2991] -> w2918
          tunnel: w2917 -> [w2942 w2966 w2990]
          tunnel: [w2942 w2966 w2990] -> w2916
          tunnel: [w2941 w2965 w2989] -> _
          tunnel: w2915 -> [w2930 w2954 w2978]
          tunnel: w2914 -> [w2929 w2953 w2977]
          tunnel: "autotune? (F)" -> [w2936 w2960 w2984]
          tunnel: [w2940 w2964 w2988] -> w2912
          tunnel: [w2922 w2945 w2969] -> w2911
          tunnel: "PID dt (s)" -> [w2932 w2956 w2980]
          tunnel: "autotuning parameters" -> [w2928 w2952 w2976]
          tunnel: [w2931 w2955 w2979] -> w2908
          tunnel: "Accept?" -> [w2927 w2951 w2975]
          tunnel: "Gain(Log)" -> [w2926 w2950 w2974]
          tunnel: [w2925 w2949 w2973] -> w2904
          tunnel: [w2925 w2949 w2973] -> w2903
          tunnel: [w2924 w2948 w2972] -> w2902
          tunnel: [w2919 w2947 w2971] -> w2901
          tunnel: [w2923 w2946 w2970] -> w2900
          tunnel: [w2922 w2945 w2969] -> w2899
          tunnel: "gamma" -> [w2921 _ _]
          tunnel: "alpha" -> [w2920 _ _]
          frame "Ch1", Default {
            w2941 = enum16{"Ch1", "Ch2", "Ch3"}."Ch1" ("Enum")
            n1292 = global read "GlobalVariables.vi" "Ch1GainLim(Log)"() -> (w2934:cluster{"GainMax":dbl, "GainMin":dbl})
            n1293 = call-poly <vilib>:"PID Online Autotuning.vi"("setpoint"=w2930, "manipulated variable"=w2926, "autotuning parameters"=w2928, "process variable"=w2929, "PID gains in"="Ch1 PID gains", "dt (s)"=w2932, "autotune? (F)"=w2936) -> ("setpoint out"=w2938:dbl, "process variable out"=w2937:dbl, "tuning completed?"=w2923:bool, "PID gains out"=w2935:T6, "tuned PID gains"=w2919:T6)  [unwired: 4 in]
            n1294 = case shown="True" w2927 {
              tunnel: w2919 -> [_ w2944]
              frame False {
              }
              frame True {
                n1295 = local write "Ch1 PID gains"(w2944) -> ()
              }
            }
            n1296 = call-poly <vilib>:"PID Advanced.vi"("setpoint"=w2938, "output range"=w2934, "auto? (T)"=TRUE, "process variable"=w2937, "gamma"=w2921, "alpha"=w2920, "PID gains"=w2935, "dt (s)"=w2932) -> ("output"=w2925:dbl, "dt out (s)"=w2931:dbl)  [unwired: 6 in]
            n1297 = Power Of 10(x=w2925) -> (10^x=w2940:dbl)
            n1298 = call "GainToCtrlV.vi"("Gain"=w2940, "Channel"=w2941) -> ("CtrlV"=w2922:dbl)  [unwired: 8 in, 1 out]
            n1299 = global read "GlobalVariables.vi" "Ch1 LJ pin"() -> (w2943:string)
            n1300 = Bundle("V target(1.0)"=w2930, w2929) -> (w2924:cluster{"V target(1.0)":dbl, dbl})  [unwired: 1 in]
          }
          frame "Ch2" {
            w2965 = enum16{"Ch1", "Ch2", "Ch3"}."Ch2" ("Enum")
            n1301 = global read "GlobalVariables.vi" "Ch2GainLim(Log)"() -> (w2958:cluster{"GainMax":dbl, "GainMin":dbl})
            n1302 = call-poly <vilib>:"PID Online Autotuning.vi"("setpoint"=w2954, "manipulated variable"=w2950, "autotuning parameters"=w2952, "process variable"=w2953, "PID gains in"="Ch2 PID gains", "dt (s)"=w2956, "autotune? (F)"=w2960) -> ("setpoint out"=w2962:dbl, "process variable out"=w2961:dbl, "tuning completed?"=w2946:bool, "PID gains out"=w2959:T6, "tuned PID gains"=w2947:T6)  [unwired: 4 in]
            n1303 = case shown="True" w2951 {
              tunnel: w2947 -> [_ w2968]
              frame False {
              }
              frame True {
                n1304 = local write "Ch2 PID gains"(w2968) -> ()
              }
            }
            n1305 = call-poly <vilib>:"PID Advanced.vi"("setpoint"=w2962, "output range"=w2958, "auto? (T)"=TRUE, "process variable"=w2961, "PID gains"=w2959, "dt (s)"=w2956) -> ("output"=w2949:dbl, "dt out (s)"=w2955:dbl)  [unwired: 8 in]
            n1306 = Power Of 10(x=w2949) -> (10^x=w2964:dbl)
            n1307 = call "GainToCtrlV.vi"("Gain"=w2964, "Channel"=w2965) -> ("CtrlV"=w2945:dbl)  [unwired: 8 in, 1 out]
            n1308 = global read "GlobalVariables.vi" "Ch2 LJ pin"() -> (w2967:string)
            n1309 = Bundle("V target(1.0)"=w2954, w2953) -> (w2948:cluster{"V target(1.0)":dbl, dbl})  [unwired: 1 in]
          }
          frame "Ch3" {
            w2989 = enum16{"Ch1", "Ch2", "Ch3"}."Ch3" ("Enum")
            n1310 = global read "GlobalVariables.vi" "Ch3GainLim(Log)"() -> (w2982:cluster{"GainMax":dbl, "GainMin":dbl})
            n1311 = call-poly <vilib>:"PID Online Autotuning.vi"("setpoint"=w2978, "manipulated variable"=w2974, "autotuning parameters"=w2976, "process variable"=w2977, "PID gains in"="Ch3 PID gains", "dt (s)"=w2980, "autotune? (F)"=w2984) -> ("setpoint out"=w2986:dbl, "process variable out"=w2985:dbl, "tuning completed?"=w2970:bool, "PID gains out"=w2983:T6, "tuned PID gains"=w2971:T6)  [unwired: 4 in]
            n1312 = case shown="True" w2975 {
              tunnel: w2971 -> [_ w2992]
              frame False {
              }
              frame True {
                n1313 = local write "Ch3 PID gains"(w2992) -> ()
              }
            }
            n1314 = call-poly <vilib>:"PID Advanced.vi"("setpoint"=w2986, "output range"=w2982, "auto? (T)"=TRUE, "process variable"=w2985, "PID gains"=w2983, "dt (s)"=w2980) -> ("output"=w2973:dbl, "dt out (s)"=w2979:dbl)  [unwired: 8 in]
            n1315 = Power Of 10(x=w2973) -> (10^x=w2988:dbl)
            n1316 = call "GainToCtrlV.vi"("Gain"=w2988, "Channel"=w2989) -> ("CtrlV"=w2969:dbl)  [unwired: 8 in, 1 out]
            n1317 = global read "GlobalVariables.vi" "Ch3 LJ pin"() -> (w2991:string)
            n1318 = Bundle("V target(1.0)"=w2978, w2977) -> (w2972:cluster{"V target(1.0)":dbl, dbl})  [unwired: 1 in]
          }
        }
        "dt out (s)" <- w2908
        "Gain(Log10)" <- w2903
        "Targer and Max" <- w2902
        "tuned PID gains" <- w2901
        "Completed?" <- w2900
        n1319 = local write "Ctrl V"(w2899) -> ()
        n1320 = local write "Gain(Log)"(w2904) -> ()
        n1321 = call "V1FGV.vi"("V1 in"=w2899) -> ()  [unwired: 9 in, 2 out]
      }
    }
    n1322 = local write "GainIndicator"(w2854) -> ()
    n1323 = call "LabJack_FGV.vi"("Operation(Read)"=enum16{"Write", "Read"}."Read" ("Operation"), "error in (no error)"=w2857) -> ("error out"=w2880:errorcluster, "Read data"=w2879:i32)  [unwired: 8 in]
    n1324 = Not Equal?(x=w2853, y=w2864) -> (x != y?=w2866:bool)
    n1325 = case shown="True" w2866 {
      tunnel: w2880 -> [w2995 w2996]
      tunnel: w2879 -> [_ w3000]
      tunnel: [w2995 w2999] -> w2860
      tunnel: w2853 -> [w2994 w2997]
      tunnel: [w2994 w2997] -> w2865
      tunnel: w2859 -> [_ w2998]
      frame False {
      }
      frame True {
        n1326 = call "LJM_eWriteName.vi"("Handle In"=w3000, "Name"=w2998, "Value"=w2997, "error in"=w2996) -> ("error out"=w2999:errorcluster)  [unwired: 10 in, 1 out]
      }
    }
    n1327 = Build Array(w2862) -> (w2861:dbl[][])
    n1328 = Bundle(w2861) -> (w2877:cluster{dbl[][]})  [unwired: 1 in]
    n1329 = Send Notification(notification=w2877, notifier=w2876) -> (notifier out=w2874:refnum<notifier>, error out=w2875:errorcluster)  [unwired: 1 in]
    n1330 = Merge Errors(w2860, w2875) -> (w2867:errorcluster)
    "processing Error Out" <- w2867
    "processing loop" <- w2868
  }
  n1331 = while {
    tunnel: w54 -> [w3013]
    tunnel: w44 -> [w3012]
    tunnel: [w3011] -> w52
    tunnel: w39 -> [w3010]
    tunnel: [w3009] -> w48
    tunnel: w27 -> [w3007]
    tunnel: w32 -> [w3006]
    tunnel: w24 -> [w3001]
    stop <- w3004 stop-if-true
    # "acquire data and send it to processing loop"
    # "Data Aquisition Loop"
    n1332 = event shown="[1] <Start digitizer>: User Event" {
      selector: w3012 -> [_ _]
      dyn-events: [_ _] -> w3011
      timeout: 20 -> [_ _]
      tunnel: w3013 -> [w3019 w3031]
      tunnel: [w3014 _] -> w3004
      tunnel: w3010 -> [w3018 w3037]
      tunnel: [w3018 w3036] -> w3009
      tunnel: w3007 -> [_ w3035]
      tunnel: w3006 -> [w3017 w3030]
      tunnel: w3001 -> [_ w3028]
      event Timeout {
        # "use queue to stop data loop\nwhen queue ref is released, error will stop this loop"
        n1333 = event-data() -> ()  [unwired: 1 in, 3 out]
        n1334 = Get Queue Status(queue=w3019) -> (error out=w3016:errorcluster)  [unwired: 2 in, 7 out]
        n1335 = Get Queue Status(queue=w3017) -> (error out=w3015:errorcluster)  [unwired: 2 in, 7 out]
        n1336 = Merge Errors(w3016, w3015) -> (w3014:errorcluster)
      }
      event User Event {
        n1337 = event-data() -> ()  [unwired: 1 in, 4 out]
        n1338 = local read "Channel"() -> (w3023:enum32{"Ch1", "Ch2", "Ch3"})
        n1339 = case shown="\"Ch1\", Default" w3023 {
          tunnel: [w3046 w3054 w3057] -> w3034
          tunnel: [w3044 w3052 w3059] -> w3027
          tunnel: [w3043 w3051 w3062] -> w3026
          tunnel: [w3042 w3050 w3061] -> w3025
          tunnel: [w3041 w3049 w3060] -> w3024
          tunnel: [w3040 w3048 w3056] -> w3022
          frame "Ch1", Default {
            w3040 = "0" ("Active Channel")
            w3047 = enum16{"Write", "Read"}."Read" ("Operation")
            n1340 = call "Digitizer1_FGV.vi"("Operation (Read)"=w3047) -> ("Read data"=w3045:refnum<k15>)  [unwired: 9 in, 1 out]
            n1341 = call "Digitizer2_FGV.vi"("Operation (Read)"=w3047) -> ("Read data"=w3046:refnum<k15>)  [unwired: 9 in, 1 out]
            n1342 = property on="Property Node" class="niScope"(reference=w3045, "Active Channel"=w3040) -> (reference out=w3044:refnum<k15>, error out=w3042:errorcluster, "Vertical Range"=w3041:dbl, "Vertical Offset"=w3043:dbl)  [unwired: 1 in]
          }
          frame "Ch2" {
            w3048 = "1" ("Active Channel")
            w3055 = enum16{"Write", "Read"}."Read" ("Operation")
            n1343 = call "Digitizer1_FGV.vi"("Operation (Read)"=w3055) -> ("Read data"=w3053:refnum<k15>)  [unwired: 9 in, 1 out]
            n1344 = call "Digitizer2_FGV.vi"("Operation (Read)"=w3055) -> ("Read data"=w3054:refnum<k15>)  [unwired: 9 in, 1 out]
            n1345 = property on="Property Node" class="niScope"(reference=w3053, "Active Channel"=w3048) -> (reference out=w3052:refnum<k15>, error out=w3050:errorcluster, "Vertical Range"=w3049:dbl, "Vertical Offset"=w3051:dbl)  [unwired: 1 in]
          }
          frame "Ch3" {
            w3056 = "0" ("Active Channel")
            w3063 = enum16{"Write", "Read"}."Read" ("Operation")
            n1346 = call "Digitizer2_FGV.vi"("Operation (Read)"=w3063) -> ("Read data"=w3058:refnum<k15>)  [unwired: 9 in, 1 out]
            n1347 = call "Digitizer1_FGV.vi"("Operation (Read)"=w3063) -> ("Read data"=w3059:refnum<k15>)  [unwired: 9 in, 1 out]
            n1348 = property on="Property Node" class="niScope"(reference=w3058, "Active Channel"=w3056) -> (reference out=w3057:refnum<k15>, error out=w3061:errorcluster, "Vertical Range"=w3060:dbl, "Vertical Offset"=w3062:dbl)  [unwired: 1 in]
          }
        }
        n1349 = local read "Task"() -> (w3020:enum32{"iRFAndGain", "Alignment"})
        n1350 = case shown="\"Alignment\"" w3020 {
          tunnel: [0.25 ("timeout") 0.75 ("timeout")] -> w3021
          frame "iRFAndGain", Default {
          }
          frame "Alignment" {
          }
        }
        n1351 = call "FLImDAQ_FGV.vi"() -> ("Read data"=w3033:T4)  [unwired: 10 in, 1 out]
        n1352 = Unbundle By Name(w3033) -> ("Waveform to Avg"=w3032:i16)
        n1353 = while {
          tunnel: w3037 -> [w3101]
          tunnel: [w3100] -> w3036
          tunnel: w3034 -> [w3098]
          tunnel: w3027 -> [w3097]
          tunnel: w3035 -> [w3096]
          shift-right: [w3080] -> _
          shift-left: u32 0 ("millisecond timer value") -> [w3092]
          tunnel: w3032 -> [w3090]
          tunnel: w3031 -> [_]
          tunnel: w3030 -> [w3088]
          tunnel: w3028 -> [w3085]
          tunnel: w3024 -> [w3081]
          tunnel: w3026 -> [w3082]
          tunnel: w3025 -> [w3075]
          tunnel: w3023 -> [w3074]
          tunnel: w3022 -> [w3073]
          tunnel: w3021 -> [w3064]
          i -> [w3089]
          stop <- w3078 stop-if-true
          # "enqueue data"
          # "send data for processing"
          n1354 = Tick Count (ms)() -> (millisecond timer value=w3080:u32)
          n1355 = Subtract(x=w3080, y=w3092) -> (x-y=→"Aquisition loop timing(ms)":u32)
          n1356 = Multiply(x=w3090, y=w3089) -> (x*y=w3083:i32)
          "Fetch Record #" <- w3083
          n1357 = property on="Property Node" class="niScope"(reference=w3097, error in=w3075, "Fetch Record Number"=w3083) -> (reference out=w3103:refnum<k15>, error out=w3102:errorcluster, "Records Done"=w3067:i32)
          "Fetch:Records Done" <- w3067
          n1358 = Subtract(x=w3067, y=w3083) -> (x-y=→"Record Backlog":i32)
          n1359 = call-poly <instrlib>:"niScope Fetch (poly).vi"("timeout"=w3064, "error in"=w3102, "channels"=w3073, "instrument handle"=w3103) -> ("error out"=w3079:errorcluster, "wfm"=w3072:i16[][])  [unwired: 4 in, 2 out]
          n1360 = case shown="\"Ch3\"" w3074 {
            tunnel: w3098 -> [_ w3117]
            tunnel: [w3109 w3116] -> w3093
            tunnel: w3083 -> [_ w3115]
            tunnel: w3079 -> [w3110 w3114]
            tunnel: [w3110 w3113] -> w3069
            tunnel: w3072 -> [w3109 _]
            tunnel: w3064 -> [_ w3111]
            frame "Ch1", "Ch2", Default {
            }
            frame "Ch3" {
              n1361 = property on="Property Node" class="niScope"(reference=w3117, error in=w3114, "Fetch Record Number"=w3115) -> (reference out=w3119:refnum<k15>, error out=w3112:errorcluster)
              n1362 = call-poly <instrlib>:"niScope Fetch (poly).vi"("timeout"=w3111, "error in"=w3112, "channels"="0", "instrument handle"=w3119) -> ("error out"=w3113:errorcluster, "wfm"=w3116:i16[][])  [unwired: 4 in, 2 out]
            }
          }
          n1363 = call "V1FGV.vi"("action (write)"=enum16{"write", "read"}."read" ("action")) -> ("V1 out"=w3066:dbl)  [unwired: 9 in, 1 out]
          n1364 = Enqueue Element(queue=w3085, element=w3066, error in (no error)=w3069) -> (error out=w3084:errorcluster)  [unwired: 1 in, 2 out]
          n1365 = Divide(x=w3093, y=65536) -> (x/y=w3095:dbl[][])
          n1366 = Multiply(x=w3095, y=w3081) -> (x*y=w3094:dbl[][])
          n1367 = Add(x=w3094, y=w3082) -> (x+y=w3070:dbl[][])
          n1368 = Bundle(w3089, w3070) -> (w3068:cluster{i32, dbl[][]})  [unwired: 1 in]
          n1369 = case shown="True" "SaveData?" {
            tunnel: w3088 -> [_ w3108]
            tunnel: [w3104 w3107] -> w3077
            tunnel: w3070 -> [_ w3106]
            tunnel: w3069 -> [w3104 w3105]
            frame False {
            }
            frame True {
              n1370 = Enqueue Element(queue=w3108, element=w3106, error in (no error)=w3105) -> (error out=w3107:errorcluster)  [unwired: 1 in, 2 out]
            }
          }
          n1371 = Send Notification(notification=w3068, notifier=w3101, error in (no error)=w3077) -> (notifier out=w3100:refnum<notifier>, error out=w3076:errorcluster)
          n1372 = Merge Errors(w3084, w3076) -> (w3087:errorcluster)
          n1373 = case shown="Error .." w3087 {
            selector: w3087 -> [w3120 w3121]
            tunnel: w3096 -> [_ w3124]
            tunnel: [w3120 w3121] -> w3078
            frame No Error {
            }
            frame Error {
              # "Send user event to signal aquisition has stoped"
              n1374 = Generate User Event(priority (normal)=usereventprio."high priority", user event=w3124, event data cluster=TRUE ("event data")) -> ()  [unwired: 1 in, 2 out]
            }
          }
          "aquisition loop Error Out" <- w3078
        }
      }
    }
    n1375 = Unbundle By Name(w3004) -> ("status"=w3003:bool)
    n1376 = Not(x=w3003) -> (.not. x?=w3002:bool)
    n1377 = local write "Aq Loop?"(w3002) -> ()
    "Aq Loop?" <- TRUE ("Aq L?")
  }
  n1378 = Close File(refnum=w10, error in=w11) -> (error out=w7:errorcluster)  [unwired: 1 out]
  n1379 = Release Queue(queue=w6, error in (no error)=w7) -> ()  [unwired: 1 in, 3 out]
  n1380 = call <vilib>:"PID Advanced Autotuning.vi"() -> ()  [unwired: 13 in, 3 out]
  n1381 = Unregister For Events(event registration refnum=w30, error in=w40) -> (error out=w41:errorcluster)
  n1382 = Release Notifier(notifier=w35, error in (no error)=w33) -> (error out=w34:errorcluster)  [unwired: 1 in, 2 out]
  n1383 = call <vilib>:"Simple Error Handler.vi"("error in (no error)"=w34) -> ()  [unwired: 4 in, 5 out]
  n1384 = Destroy User Event(user event=w27, error in=w41) -> ()  [unwired: 1 out]
  n1385 = Release Notifier(notifier=w48, error in (no error)=w47) -> (error out=w46:errorcluster)  [unwired: 1 in, 2 out]
  n1386 = Unregister For Events(event registration refnum=w52, error in=w50) -> (error out=w51:errorcluster)
  n1387 = call <vilib>:"Simple Error Handler.vi"("error in (no error)"=w46) -> ()  [unwired: 4 in, 5 out]
  n1388 = Destroy User Event(user event=w42, error in=w51) -> ()  [unwired: 1 out]
